vi "pickOffensiveRobots.vi"(8 "error in (no error)":errorcluster, 11 "Game in":refnum<class "Game.lvclass">) -> (0 "error out":errorcluster, 3 "Game out":refnum<class "Game.lvclass">)   [LabVIEW 2021, in "Game.lvclass"]
uses:
  Game.lvclass
  Game.lvclass/Game.ctl
  Team_class/Team.lvclass/Team.ctl
  Playbook_class/Playbook.lvclass/Playbook.ctl
  TestPlay_class/TestPlay.lvclass/TestPlay.ctl
  Robot_class/roles.ctl
  Robot_class/Robot.lvclass/Robot.ctl
  Role_class/Role.lvclass/Role.ctl
  PreparePenaltyAllyPlay_class/PreparePenaltyAllyPlay.lvclass/PreparePenaltyAllyPlay.ctl
  IndirectEnemyPlay_class/IndirectEnemyPlay.lvclass/IndirectEnemyPlay.ctl
  DirectEnemyPlay_class/DirectEnemyPlay.lvclass/DirectEnemyPlay.ctl
  NormalGamePlay_class/NormalGamePlay.lvclass/NormalGamePlay.ctl
  PreparePassInGame1_class/PreparePassInGame1.lvclass/PreparePassInGame1.ctl
  HaltPlay_class/HaltPlay.lvclass/HaltPlay.ctl
  BallOutOfFieldPlay_class/BallOutOfFieldPlay.lvclass/BallOutOfFieldPlay.ctl
  StopOffensivePlay_class/StopOffensivePlay.lvclass/StopOffensivePlay.ctl
  EnemyPossessionAtOurFieldPlay_class/EnemyPossessionAtOurFieldPlay.lvclass/EnemyPossessionAtOurFieldPlay.ctl
  PrepareKickoffAllyPlay_class/PrepareKickoffAllyPlay.lvclass/PrepareKickoffAllyPlay.ctl
  PrepareKickoffEnemyPlay_class/PrepareKickoffEnemyPlay.lvclass/PrepareKickoffEnemyPlay.ctl
  PreparePassPlay_class/PreparePassPlay.lvclass/PreparePassPlay.ctl
  PrepareDoublePassPlay_class/PrepareDoublePassPlay.lvclass/PrepareDoublePassPlay.ctl
  ACBPassPlay_class/ACBPassPlay.lvclass/ACBPassPlay.ctl
  PrepareRollToPassPlay_class/PrepareRollToPassPlay.lvclass/PrepareRollToPassPlay.ctl
  TableWithStrikerPlay_class/TableWithStrikerPlay.lvclass/TableWithStrikerPlay.ctl
  TableWith2ndStrikerPlay_class/TableWith2ndStrikerPlay.lvclass/TableWith2ndStrikerPlay.ctl
  KeeperPassToStrikerPlay_class/KeeperPassToStrikerPlay.lvclass/KeeperPassToStrikerPlay.ctl
  PreparePenaltyEnemyPlay_class/PreparePenaltyEnemyPlay.lvclass/PreparePenaltyEnemyPlay.ctl
  KickPenaltyAllyPlay_class/KickPenaltyAllyPlay.lvclass/KickPenaltyAllyPlay.ctl
  Role_class/Write RobotRef.vi
  TestPlay_class/Read Roles.vi
  Robot_class/Write role.vi
  TestPlay_class/Write Roles.vi
  Playbook_class/Write offensive_plays.vi
  Playbook_class/Read offensive_plays.vi
  TestPlay_class/Read NumberOfRobots.vi
  PreparePenaltyAllyPlay_class/Read Roles.vi
  PreparePenaltyAllyPlay_class/Write Roles.vi
  PreparePenaltyAllyPlay_class/Read NumberOfRobots.vi
  IndirectEnemyPlay_class/Read Roles.vi
  IndirectEnemyPlay_class/Write Roles.vi
  DirectEnemyPlay_class/Read Roles.vi
  DirectEnemyPlay_class/Write Roles.vi
  Read EnemyRef.vi
  Read NewParameters.vi
  Team_class/Read RobotRef.vi
  NormalGamePlay_class/Read Roles.vi
  NormalGamePlay_class/Write Roles.vi
  NormalGamePlay_class/Read NumberOfRobots.vi
  PreparePassInGame1_class/Read Roles.vi
  PreparePassInGame1_class/Write Roles.vi
  HaltPlay_class/Read Roles.vi
  HaltPlay_class/Write Roles.vi
  BallOutOfFieldPlay_class/Read Roles.vi
  BallOutOfFieldPlay_class/Write Roles.vi
  BallOutOfFieldPlay_class/Read NumberOfRobots.vi
  StopOffensivePlay_class/Read Roles.vi
  StopOffensivePlay_class/Write Roles.vi
  StopOffensivePlay_class/Read NumberOfRobots.vi
  EnemyPossessionAtOurFieldPlay_class/Read Roles.vi
  EnemyPossessionAtOurFieldPlay_class/Write Roles.vi
  PrepareKickoffAllyPlay_class/Read Roles.vi
  PrepareKickoffAllyPlay_class/Write Roles.vi
  PrepareKickoffEnemyPlay_class/Read Roles.vi
  PrepareKickoffEnemyPlay_class/Write Roles.vi
  PreparePassPlay_class/Read Roles.vi
  PreparePassPlay_class/Write Roles.vi
  PrepareDoublePassPlay_class/Read Roles.vi
  PrepareDoublePassPlay_class/Write Roles.vi
  PrepareDoublePassPlay_class/Read NumberOfRobots.vi
  ACBPassPlay_class/Read Roles.vi
  ACBPassPlay_class/Write Roles.vi
  ACBPassPlay_class/Read NumberOfRobots.vi
  PrepareRollToPassPlay_class/Read Roles.vi
  PrepareRollToPassPlay_class/Write Roles.vi
  PrepareRollToPassPlay_class/Read NumberOfRobots.vi
  TableWithStrikerPlay_class/Read Roles.vi
  TableWithStrikerPlay_class/Write Roles.vi
  TableWithStrikerPlay_class/Read NumberOfRobots.vi
  TableWith2ndStrikerPlay_class/Read Roles.vi
  TableWith2ndStrikerPlay_class/Write Roles.vi
  TableWith2ndStrikerPlay_class/Read NumberOfRobots.vi
  KeeperPassToStrikerPlay_class/Read Roles.vi
  KeeperPassToStrikerPlay_class/Write Roles.vi
  KeeperPassToStrikerPlay_class/Read NumberOfRobots.vi
  PreparePenaltyEnemyPlay_class/Read roles.vi
  PreparePenaltyEnemyPlay_class/Write roles.vi
  PreparePenaltyEnemyPlay_class/Read NumberOfRobots.vi
  KickPenaltyAllyPlay_class/Read Roles.vi
  KickPenaltyAllyPlay_class/Write Rolesvi.vi
  KickPenaltyAllyPlay_class/Read NumberOfRobots.vi
  Read OffensiveTeam.vi
  Read AllyRef.vi
  Read Referee.vi
  Read TestMode IDs.vi
  Read KeeperTeam.vi
  Team_class/Read OffensivePlay.vi
  Team_class/Write OffensivePlay.vi
  Team_class/Write RobotRef.vi
  Write OffensiveTeam.vi
  Ally_class/Ally.lvclass
  C:/Users/rdapa/Desktop/RoboIME/SSL_AI/Team_class/Team.lvclass
  TestRole_class/TestRole.lvclass
  C:/Users/rdapa/Desktop/RoboIME/SSL_AI/Role_class/Role.lvclass
  PassBestReceiverRole_class/PassBestReceiverRole.lvclass
  5RobotsRole_class/5RobotsRole.lvclass
  AttackerAimGoalRole_class/AttackerAimGoalRole.lvclass
  PenaltyDefenseRole_class/PenaltyDefenseRole.lvclass
  AttackerBlockRole_class/AttackerBlockRole.lvclass
  MarkerRole_class/MarkerRole.lvclass
  Enemy_class/Enemy.lvclass
  ShootRole_class/ShootRole.lvclass
  FollowAttackerRole_class/FollowAttackerRole.lvclass
  AttackerStopRole_class/AttackerStopRole.lvclass
  PassBestRobotRole_class/PassBestRobotRole.lvclass
  PreparePassReceiverRole_class/PreparePassReceiverRole.lvclass
  HaltRole_class/HaltRole.lvclass
  BallOutOfFieldRole_class/BallOutOfFieldRole.lvclass
  ABCFirstKickerRole_class/ABCFirstKickerRole.lvclass
  ABCSecondKicker_class/ABCSecondKicker.lvclass
  ABCThirdKicker_class/ABCThirdKicker.lvclass
  PrepareRollToPassReceiverRole_class/PrepareRollToPassReceiverRole.lvclass
  PrepareRollToPassRollerRole_class/PrepareRollToPassRollerRole.lvclass
  SimplePassReceiverRole_class/SimplePassReceiverRole.lvclass
  SimplePassRollRole_class/SimplePassRollRole.lvclass
  PassKickerRole_class/PassKickerRole.lvclass
  PassReceiverRole_class/PassReceiverRole.lvclass
  PassObserverRole_class/PassObserverRole.lvclass
  TableFinalizerRole_class/TableFinalizerRole.lvclass
  TablerRole_class/TablerRole.lvclass
  WaitPassRole_class/WaitPassRole.lvclass
  PenaltyAttackerRole_class/PenaltyAttackerRole.lvclass
  Referee_class/Referee.lvclass
  Playbook_class/Playbook.lvclass
  Robot_class/Robot.lvclass
  Play_class/Play.lvclass
  TestPlay_class/TestPlay.lvclass
  EnemyPossessionAtEnemyFieldPlay_class/EnemyPossessionAtEnemyFieldPlay.lvclass
  EnemyPossessionAtOurFieldPlay_class/EnemyPossessionAtOurFieldPlay.lvclass
  NormalGamePlay_class/NormalGamePlay.lvclass
  IndirectEnemyPlay_class/IndirectEnemyPlay.lvclass
  PrepareKickoffAllyPlay_class/PrepareKickoffAllyPlay.lvclass
  PrepareKickoffEnemyPlay_class/PrepareKickoffEnemyPlay.lvclass
  KickPenaltyAllyPlay_class/KickPenaltyAllyPlay.lvclass
  PreparePenaltyAllyPlay_class/PreparePenaltyAllyPlay.lvclass
  DirectEnemyPlay_class/DirectEnemyPlay.lvclass
  PreparePenaltyEnemyPlay_class/PreparePenaltyEnemyPlay.lvclass
  BallOutOfFieldPlay_class/BallOutOfFieldPlay.lvclass
  StopOffensivePlay_class/StopOffensivePlay.lvclass
  PassPlay_class/PassPlay.lvclass
  DirectKickPlay_class/DirectKickPlay.lvclass
  HaltPlay_class/HaltPlay.lvclass
  PreparePassPlay_class/PreparePassPlay.lvclass
  PassToStriker_class/PassToStriker.lvclass
  PassTo2ndStriker_class/PassTo2ndStriker.lvclass
  SimplePass_class/SimplePass.lvclass
  PrepareRollToPassPlay_class/PrepareRollToPassPlay.lvclass
  PrepareDoublePassPlay_class/PrepareDoublePassPlay.lvclass
  TableWith2ndStrikerPlay_class/TableWith2ndStrikerPlay.lvclass
  TableWithStrikerPlay_class/TableWithStrikerPlay.lvclass
  PrepareTriplePassPlay_class/PrepareTriplePassPlay.lvclass
  ABCPassPlay_class/ABCPassPlay.lvclass
  PreparePassInGame1_class/PreparePassInGame1.lvclass
  ACBPassPlay_class/ACBPassPlay.lvclass
  PrepareKeeperPassPlay_class/PrepareKeeperPassPlay.lvclass
  KeeperPassToStrikerPlay_class/KeeperPassToStrikerPlay.lvclass
  5RobotsNormalGamePlay_class/5RobotsNormalGamePlay.lvclass
  5RobotsPassGamePlay_class/5RobotsPassGamePlay.lvclass
  5RobotsKeeperGame_class/5RobotsKeeperGame.lvclass
  5PreparePassGamePlay_class/5PreparePassGamePlay.lvclass
  Role_class/Role.lvclass
  SecondMarkerRole_class/SecondMarkerRole.lvclass
  MarkerSkill_class/MarkerSkill.lvclass
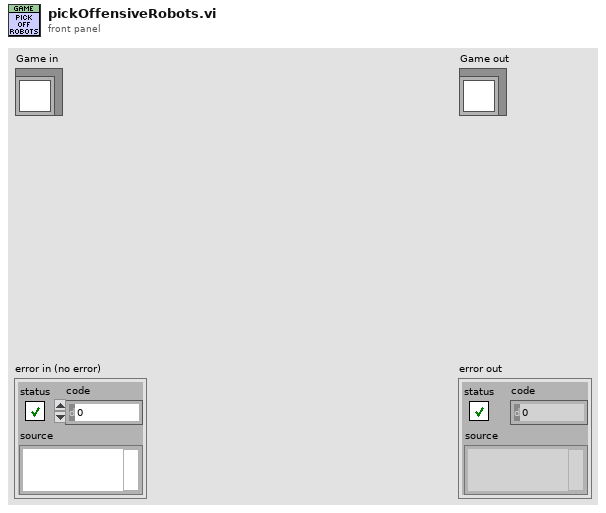
[diagram p1: front panel]
types:
  T1 = typedef "roles.ctl" = enum16{"SimpleBallPlacement", "BallPlacementAllyPasser", "BallPlacementAllyReceiver", "BallPlacementEnemy", "5Robots5th", "PassBestReceiver", "5Robots4th", "5Robots3rd", "5Robots2nd", "5Robots1st", "PassBestRobot", "WaitPass", "ABCThirdKicker", "ABCFirstKicker", "ABCSecondKicker", "Tabler", "TableFinalizer", "PrepareRollToPassRoller", "PrepareRollToPassReceiver", "SimplePassRoll", "SimplePassRollReceiver", "PenaltyDefense", "PreparePassReceiver 2", "PreparePassReceiver 1", "PassObserver", "Timeout", "Goto", "ZigZag", "None", "BallOutOfField", "DefenderArea", "Duelist", "AttackerStop", "FollowAttacker", "KeeperRole", "KickPenalty", "AttackerAimGoal", "AttackerBlock", "Marker", "Halt", "Shoot", "PassKicker", "PassReceiver", "TestRole", "PenaltyAttacker"}
  T2 = typedef "NewParameters.ctl" = cluster{"PenaltyDistance":dbl, "DistanceAttackerToBackBall":dbl, "Division":enum16{"Div B", "Div A"}, "DistanceToAvoidyEnemyRobot":dbl, "BallPlacementDistance":dbl, "DisatanceBehindBallToStealBall":dbl, "MaxDistanceToPositionKickoff":dbl, "BlockEnemyTarget":bool, "MaxStopVAng":dbl, "DistanceMarkerToEnemy":dbl, "IgnoreDribblerContact":bool, "DistanceToBeginEnemyPosession":dbl, "GoToBallWhenEnemyNotMoving":bool, "EnemyDistanceToReduceVelocity":dbl, "TurnOnEnemyDistanceToReduceVelocity":bool, "EnemyDistanceToShootOutBall":dbl, "DefenseKickBall":bool, "MoreKickToGoal? (0-0.3)":dbl, "ChipKickInEnemyField":bool, "ShootOutRobotId":dbl, "FieldLenghtDenominatorInShootOut":dbl, "AdjustPositionInBallPlacement":bool, "PowerGodPass":dbl, "VelocityAbortEnemyPos":dbl, "MaxDistToBeginPass":dbl, "MinDistToBeginPass":dbl, "VelocityInDirects":dbl, "BadDribblerIDs":i32[], "NewKickToDistanceAroundBall":dbl, "PowerAvoidColisionMarker":dbl, "DistanceToAvoidColisionMarker":dbl, "AvoidBallKick":dbl, "DistanceTryKick":dbl, "SuicideKickDIstance":dbl, "FirstKickAtck":bool, "AdjustFirstKickDistance":dbl, "FirstKickDefense":bool, "AvoidAimLessKick":dbl, "DistanceToAvoidyEnemyShootRobot ":dbl, "NumberOfMarkers":dbl, "PotField":bool, "PIDLateral":bool, "MinDistanceFirstKickX":dbl, "MinDistanceFirstKickY":dbl, "FractionOfDistToTouchGround\nAfterChipKick":dbl, "FractionOfKickxWhen\nComposedWithKickz":dbl, "Style":T3, "MoveInTurnState":bool, "DistFromEnemyToConsider\nMoveInTurnState":dbl, "CascadePID":bool, "TurnAroundParameters":cluster{"Radius":dbl, "Multiplier":dbl, "ChordAngle":dbl}, "SafeDriveVel":dbl, "DistanceToGoToBackBall":dbl, "minDistanceToNotFinishEnemyPossession":dbl, "TheBestKickers":i32[]}
  T3 = typedef "Style.ctl" = enum16{"Insanity", "Offensive", "Defensive"}
  T4 = typedef "OffensivePlay.ctl" = enum16{"5RobotsPassGamePlay", "5PreparePassGame", "5RobotsKeeperGame", "KeeperPassToStriker", "5RobotsNormalGamePlay", "PrepareKeeperPass", "ACBPass", "ABCPass", "PrepareTriplePass", "TableWithStriker", "TableWith2ndStrikerPlay", "PrepareDoublePass", "PrepareRollToPass", "SimplePass", "PreparePass", "PassToStriker", "BallOutOfField", "PassTo2ndStriker", "StopOffensive", "Prepare Penalty Enemy", "EnemyPossessionAtEnemyField", "EnemyPossesionAtOurField", "TestPlay", "PreparePenaltyAlly", "KickPenaltyAlly", "PrepareKickoffAlly", "PrepareKickoffEnemy", "IndirectEnemy", "DirectEnemy", "PreparePassInGame1", "NormalGame", "DirectKick", "Pass", "Halt", "Timeout", "PassPlay", "PenaltyEnemy"}
  T5 = typedef "offensive_plays.ctl" = cluster{"Play":refnum<class "Play.lvclass">, "TestPlay":refnum<class "TestPlay.lvclass">, "EnemyPossessionAtEnemyFieldPlay":refnum<class "EnemyPossessionAtEnemyFieldPlay.lvclass">, "EnemyPossessionAtOurFieldPlay":refnum<class "EnemyPossessionAtOurFieldPlay.lvclass">, "NormalGamePlay":refnum<class "NormalGamePlay.lvclass">, "IndirectEnemyPlay":refnum<class "IndirectEnemyPlay.lvclass">, "PrepareKickoffAllyPlay":refnum<class "PrepareKickoffAllyPlay.lvclass">, "PrepareKickoffEnemyPlay":refnum<class "PrepareKickoffEnemyPlay.lvclass">, "KickPenaltyAllyPlay":refnum<class "KickPenaltyAllyPlay.lvclass">, "PreparePenaltyAllyPlay":refnum<class "PreparePenaltyAllyPlay.lvclass">, "DirectEnemyPlay":refnum<class "DirectEnemyPlay.lvclass">, "PreparePenaltyEnemyPlay":refnum<class "PreparePenaltyEnemyPlay.lvclass">, "BallOutOfFieldPlay":refnum<class "BallOutOfFieldPlay.lvclass">, "StopOffensivePlay":refnum<class "StopOffensivePlay.lvclass">, "PassPlay":refnum<class "PassPlay.lvclass">, "DirectKickPlay":refnum<class "DirectKickPlay.lvclass">, "HaltPlay":refnum<class "HaltPlay.lvclass">, "PreparePassPlay":refnum<class "PreparePassPlay.lvclass">, "PassToStrikerPlay":refnum<class "PassToStriker.lvclass">, "PassTo2ndStrikerPlay":refnum<class "PassTo2ndStriker.lvclass">, "SimplePassPlay":refnum<class "SimplePass.lvclass">, "PrepareRollToPassPlay":refnum<class "PrepareRollToPassPlay.lvclass">, "PrepareDoublePassPlay":refnum<class "PrepareDoublePassPlay.lvclass">, "TableWith2ndStrikerPlay":refnum<class "TableWith2ndStrikerPlay.lvclass">, "TableWithStrikerPlay":refnum<class "TableWithStrikerPlay.lvclass">, "PrepareTriplePassPlay":refnum<class "PrepareTriplePassPlay.lvclass">, "ABCPassPlay":refnum<class "ABCPassPlay.lvclass">, "PreparePassInGame1":refnum<class "PreparePassInGame1.lvclass">, "ACBPassPlay":refnum<class "ACBPassPlay.lvclass">, "PrepareKeeperPassPlay":refnum<class "PrepareKeeperPassPlay.lvclass">, "KeeperPassToStrikerPlay":refnum<class "KeeperPassToStrikerPlay.lvclass">, "SimplePass":refnum<class "SimplePass.lvclass">, "SimplePass 2":refnum<class "SimplePass.lvclass">, "5RobotsNormalGamePlay":refnum<class "5RobotsNormalGamePlay.lvclass">, "5RobotsPassGamePlay":refnum<class "5RobotsPassGamePlay.lvclass">, "5RobotsKeeperGame":refnum<class "5RobotsKeeperGame.lvclass">, "5PreparePassGamePlay":refnum<class "5PreparePassGamePlay.lvclass">}
  T6 = cluster{"TestRole 1":refnum<class "TestRole.lvclass">, "Role":refnum<class "Role.lvclass">, "TestRole 2":refnum<class "TestRole.lvclass">, "TestRole 3":refnum<class "TestRole.lvclass">}
  T7 = cluster{"5RobotsRole3rd":refnum<class "5RobotsRole.lvclass">, "5RobotsRole2nd":refnum<class "5RobotsRole.lvclass">, "5RobotsRole1st":refnum<class "5RobotsRole.lvclass">, "5RobotsRole4th":refnum<class "5RobotsRole.lvclass">, "PassBestReceiverRole":refnum<class "PassBestReceiverRole.lvclass">}
  T8 = cluster{"AttackerAimGoalRole":refnum<class "AttackerAimGoalRole.lvclass">, "PenaltyDefenseRole 4":refnum<class "PenaltyDefenseRole.lvclass">, "PenaltyDefenseRole 1":refnum<class "PenaltyDefenseRole.lvclass">, "PenaltyDefenseRole 2":refnum<class "PenaltyDefenseRole.lvclass">, "PenaltyDefenseRole 3":refnum<class "PenaltyDefenseRole.lvclass">}
  T9 = cluster{"AttackerBlockRole":refnum<class "AttackerBlockRole.lvclass">, "MarkerRole":refnum<class "MarkerRole.lvclass">}
  T10 = typedef "directEnemyRoles.ctl" = cluster{"AttackerBlockRole":refnum<class "AttackerBlockRole.lvclass">, "MarkerRole":refnum<class "MarkerRole.lvclass">, "SecondMarkerRole":refnum<class "SecondMarkerRole.lvclass">}
  T11 = cluster{"ShootRole":refnum<class "ShootRole.lvclass">, "FollowAttackerRole":refnum<class "FollowAttackerRole.lvclass">}
  T12 = cluster{"5RobotsRole1st":refnum<class "5RobotsRole.lvclass">, "5RobotsRole2nd ":refnum<class "5RobotsRole.lvclass">, "5RobotsRole3rd":refnum<class "5RobotsRole.lvclass">, "5RobotsRole4th":refnum<class "5RobotsRole.lvclass">, "ShootRole":refnum<class "ShootRole.lvclass">}
  T13 = cluster{"5RobotsRole1st":refnum<class "5RobotsRole.lvclass">, "5RobotsRole2nd ":refnum<class "5RobotsRole.lvclass">, "5RobotsRole3rd":refnum<class "5RobotsRole.lvclass">, "5RobotsRole4th":refnum<class "5RobotsRole.lvclass">, "AttackerStopRole":refnum<class "AttackerStopRole.lvclass">}
  T14 = cluster{"PassBestRobotRole":refnum<class "PassBestRobotRole.lvclass">, "5RobotsRole3rd":refnum<class "5RobotsRole.lvclass">, "5RobotsRole2nd":refnum<class "5RobotsRole.lvclass">, "5RobotsRole1st":refnum<class "5RobotsRole.lvclass">, "PassBestReceiverRole":refnum<class "PassBestReceiverRole.lvclass">}
  T15 = cluster{"PreparePassReceiverRole1":refnum<class "PreparePassReceiverRole.lvclass">, "PreparePassReceiverRole 2":refnum<class "PreparePassReceiverRole.lvclass">}
  T16 = cluster{"ShootRole":refnum<class "ShootRole.lvclass">, "PreparePassReceiverRole1":refnum<class "PreparePassReceiverRole.lvclass">, "PreparePassReceiverRole2":refnum<class "PreparePassReceiverRole.lvclass">}
  T17 = cluster{"HaltRole 1":refnum<class "HaltRole.lvclass">, "HaltRole 2":refnum<class "HaltRole.lvclass">, "HaltRole 3":refnum<class "HaltRole.lvclass">, "HaltRole 4":refnum<class "HaltRole.lvclass">, "HaltRole 5":refnum<class "HaltRole.lvclass">, "HaltRole 6":refnum<class "HaltRole.lvclass">}
  T18 = cluster{"BallOutOfFieldRole":refnum<class "BallOutOfFieldRole.lvclass">, "FollowAttackerRole":refnum<class "FollowAttackerRole.lvclass">}
  T19 = cluster{"MarkerRole":refnum<class "MarkerRole.lvclass">, "AttackerStopRole":refnum<class "AttackerStopRole.lvclass">}
  T20 = typedef "EnemyPossessionAtOurFieldRoles.ctl" = cluster{"ShootRole":refnum<class "ShootRole.lvclass">, "MarkerRole":refnum<class "MarkerRole.lvclass">}
  T21 = cluster{"AttackerAimGoalRole":refnum<class "AttackerAimGoalRole.lvclass">, "FollowAttackerRole":refnum<class "FollowAttackerRole.lvclass">}
  T22 = cluster{"AttackerBlockRole":refnum<class "AttackerBlockRole.lvclass">, "FollowAttackerRole":refnum<class "FollowAttackerRole.lvclass">}
  T23 = cluster{"PreparePassReceiverRole 1":refnum<class "PreparePassReceiverRole.lvclass">, "AttackerStopRole":refnum<class "AttackerStopRole.lvclass">, "PreparePassReceiverRole 2":refnum<class "PreparePassReceiverRole.lvclass">}
  T24 = cluster{"AttackerStopRole":refnum<class "AttackerStopRole.lvclass">, "PreparePassReceiverRole 1":refnum<class "PreparePassReceiverRole.lvclass">, "PreparePassReceiverRole 2":refnum<class "PreparePassReceiverRole.lvclass">}
  T25 = cluster{"PreparePassReceiverRole 1":refnum<class "PreparePassReceiverRole.lvclass">, "PreparePassReceiverRole 2":refnum<class "PreparePassReceiverRole.lvclass">, "AttackerStopRole":refnum<class "AttackerStopRole.lvclass">}
  T26 = cluster{"ABCSecondKicker":refnum<class "ABCSecondKicker.lvclass">, "ABCThirdKicker":refnum<class "ABCThirdKicker.lvclass">, "ABCFirstKickerRole":refnum<class "ABCFirstKickerRole.lvclass">}
  T27 = cluster{"PreparePassReceiverRole 1":refnum<class "PreparePassReceiverRole.lvclass">, "PreparePassReceiverRole 2":refnum<class "PreparePassReceiverRole.lvclass">, "PrepareRollToPassReceiverRole":refnum<class "PrepareRollToPassReceiverRole.lvclass">, "PrepareRollToPassRollerRole":refnum<class "PrepareRollToPassRollerRole.lvclass">}
  T28 = cluster{"SimplePassRollRole":refnum<class "SimplePassRollRole.lvclass">, "SimplePassReceiverRole":refnum<class "SimplePassReceiverRole.lvclass">}
  T29 = cluster{"PassKickerRole":refnum<class "PassKickerRole.lvclass">, "PassReceiverRole":refnum<class "PassReceiverRole.lvclass">, "PassObserverRole":refnum<class "PassObserverRole.lvclass">}
  T30 = cluster{"TableFinalizerRole":refnum<class "TableFinalizerRole.lvclass">, "TablerRole":refnum<class "TablerRole.lvclass">, "PassObserverRole":refnum<class "PassObserverRole.lvclass">}
  T31 = cluster{"WaitPassRole":refnum<class "WaitPassRole.lvclass">, "FollowAttackerRole":refnum<class "FollowAttackerRole.lvclass">}
  T32 = cluster{"PenaltyDefenseRole 1":refnum<class "PenaltyDefenseRole.lvclass">, "PenaltyDefenseRole 2":refnum<class "PenaltyDefenseRole.lvclass">, "PenaltyDefenseRole 3":refnum<class "PenaltyDefenseRole.lvclass">, "PenaltyDefenseRole 4":refnum<class "PenaltyDefenseRole.lvclass">, "PenaltyDefenseRole 5":refnum<class "PenaltyDefenseRole.lvclass">}
  T33 = typedef "kickPenaltyAllyRoles.ctl" = cluster{"PenaltyAttackerRole":refnum<class "PenaltyAttackerRole.lvclass">, "HaltRole":refnum<class "HaltRole.lvclass">, "HaltRole 2":refnum<class "HaltRole.lvclass">, "HaltRole 3":refnum<class "HaltRole.lvclass">, "HaltRole 4":refnum<class "HaltRole.lvclass">, "HaltRole 5":refnum<class "HaltRole.lvclass">}
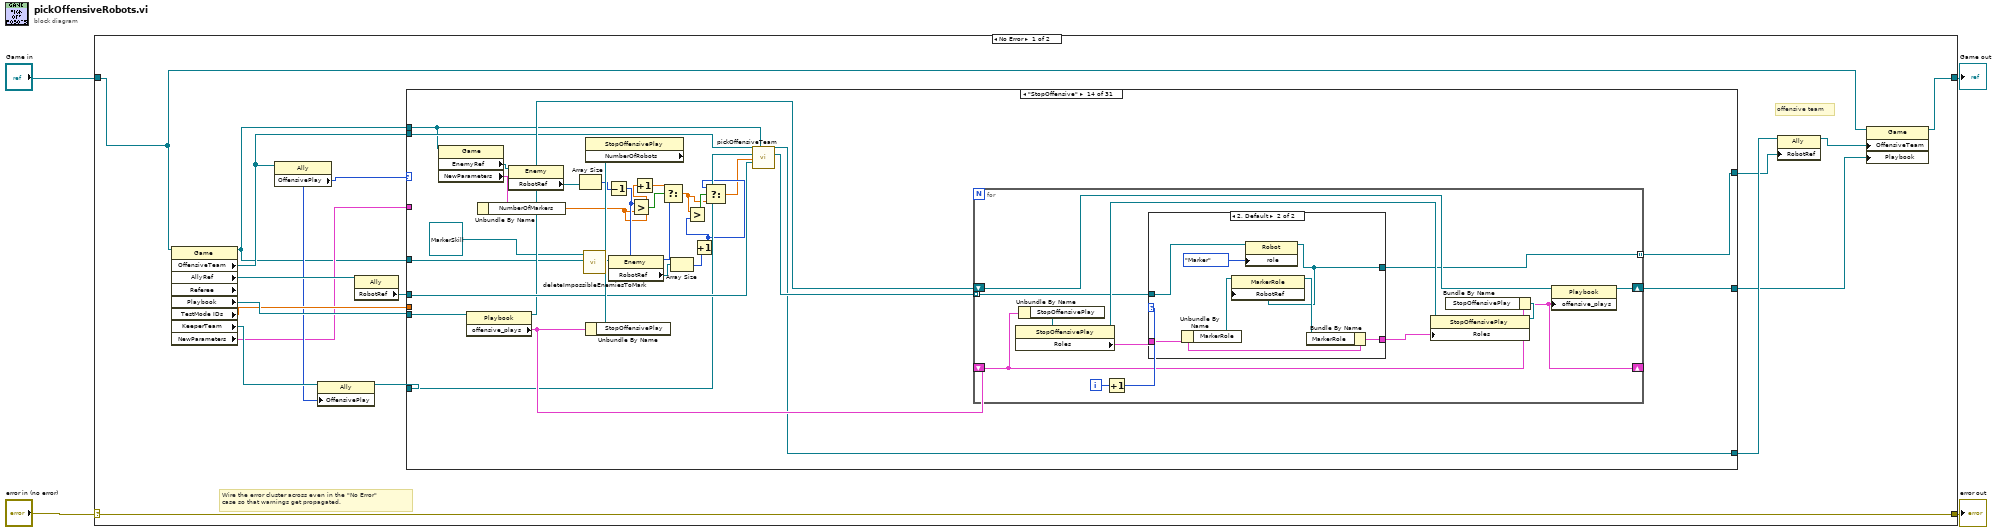
[diagram p0: block diagram]
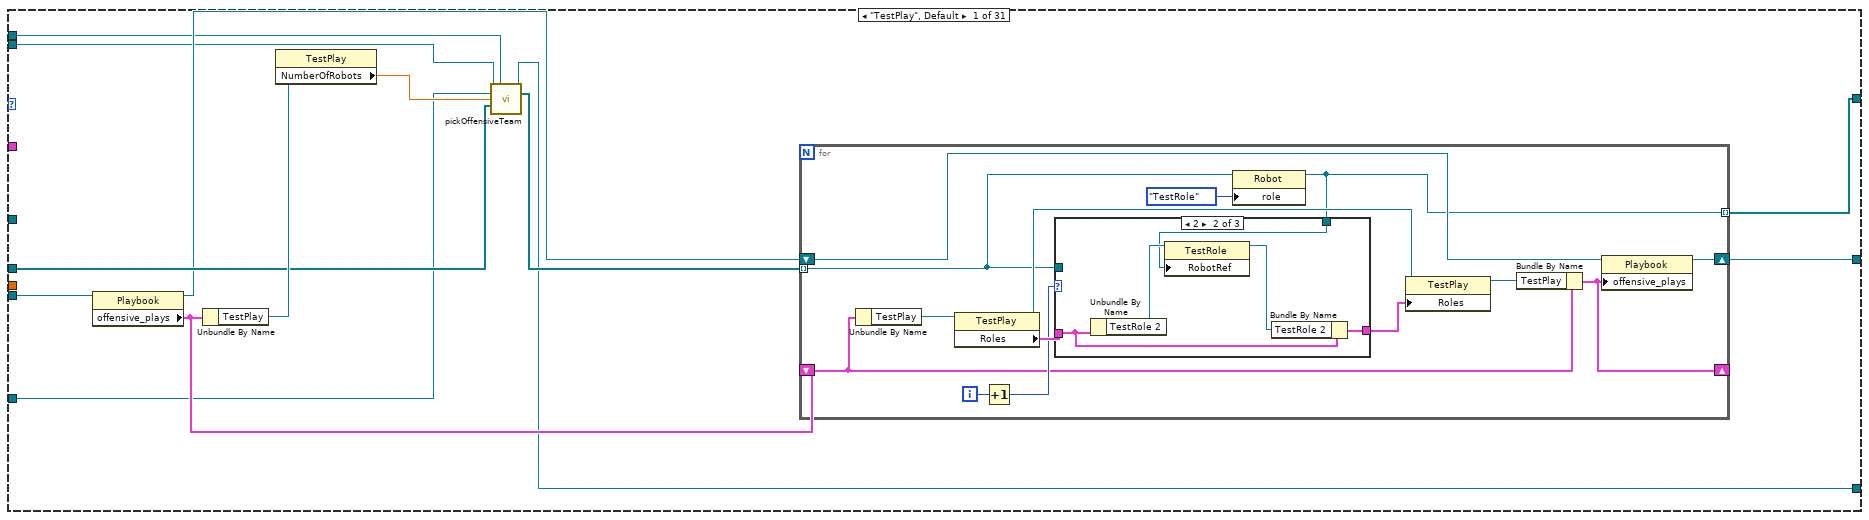
[diagram p2: hidden frame]
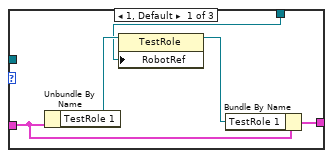
[diagram p3: hidden frame]
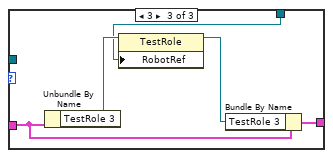
[diagram p4: hidden frame]
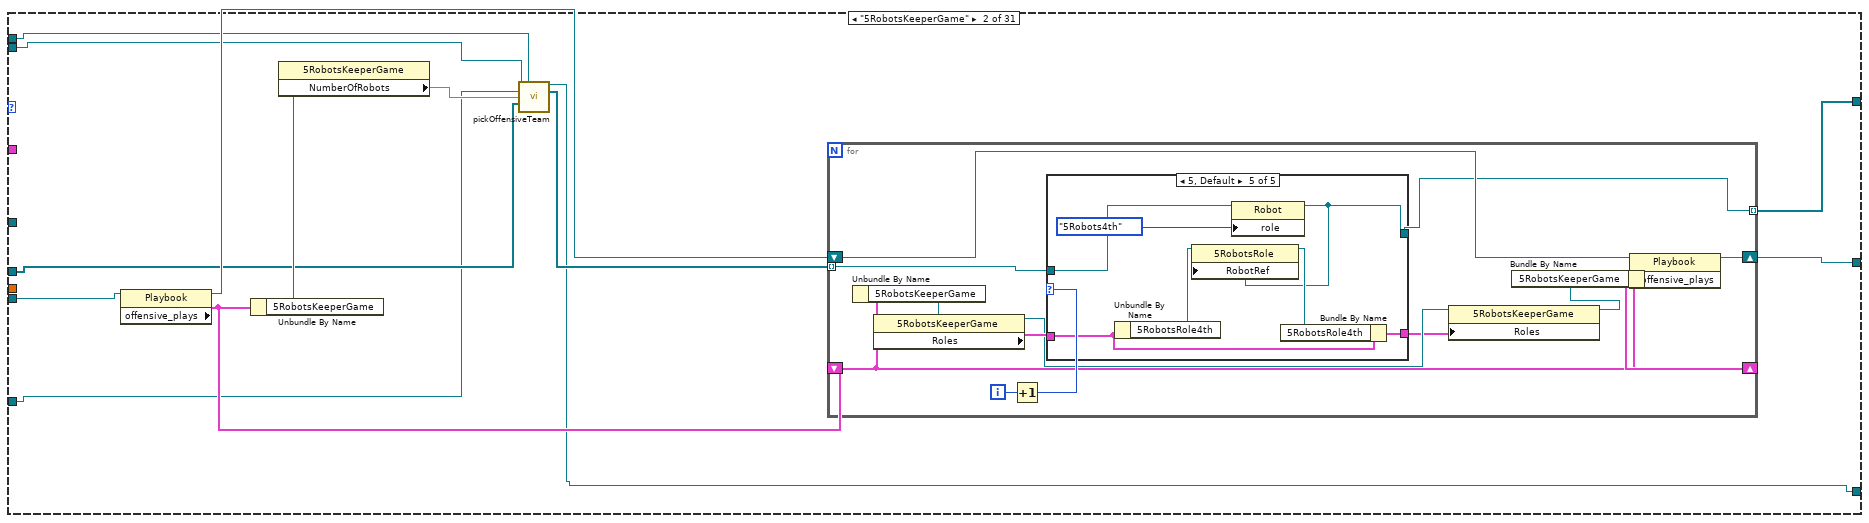
[diagram p5: hidden frame]
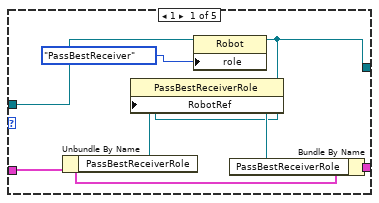
[diagram p6: hidden frame]
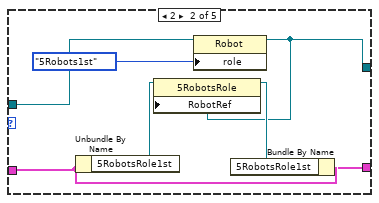
[diagram p7: hidden frame]
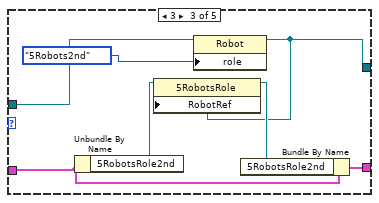
[diagram p8: hidden frame]
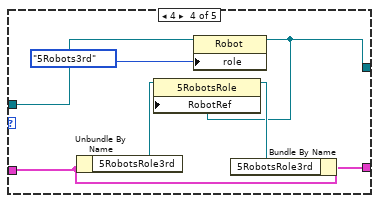
[diagram p9: hidden frame]
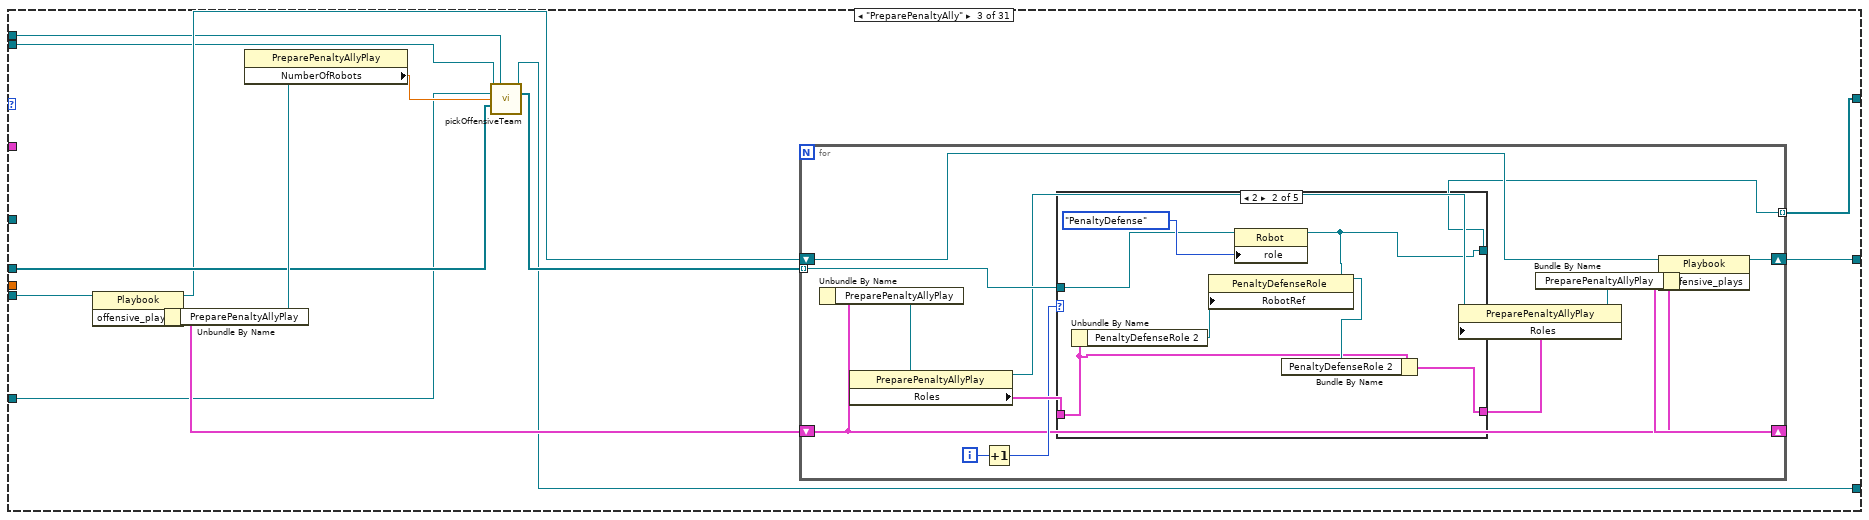
[diagram p10: hidden frame]
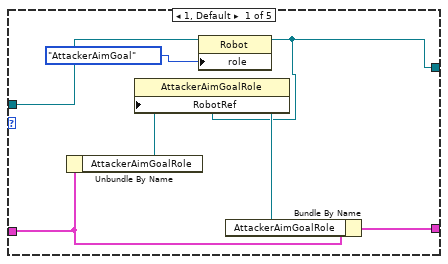
[diagram p11: hidden frame]
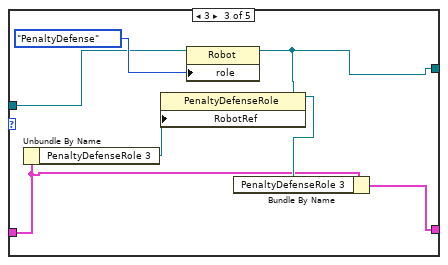
[diagram p12: hidden frame]
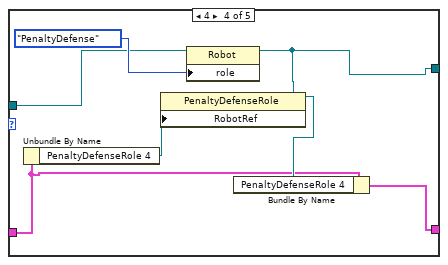
[diagram p13: hidden frame]
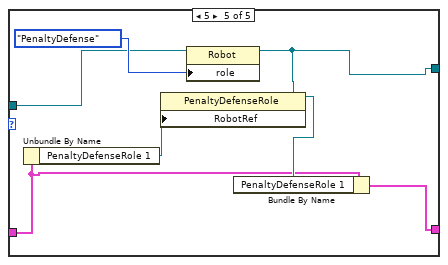
[diagram p14: hidden frame]
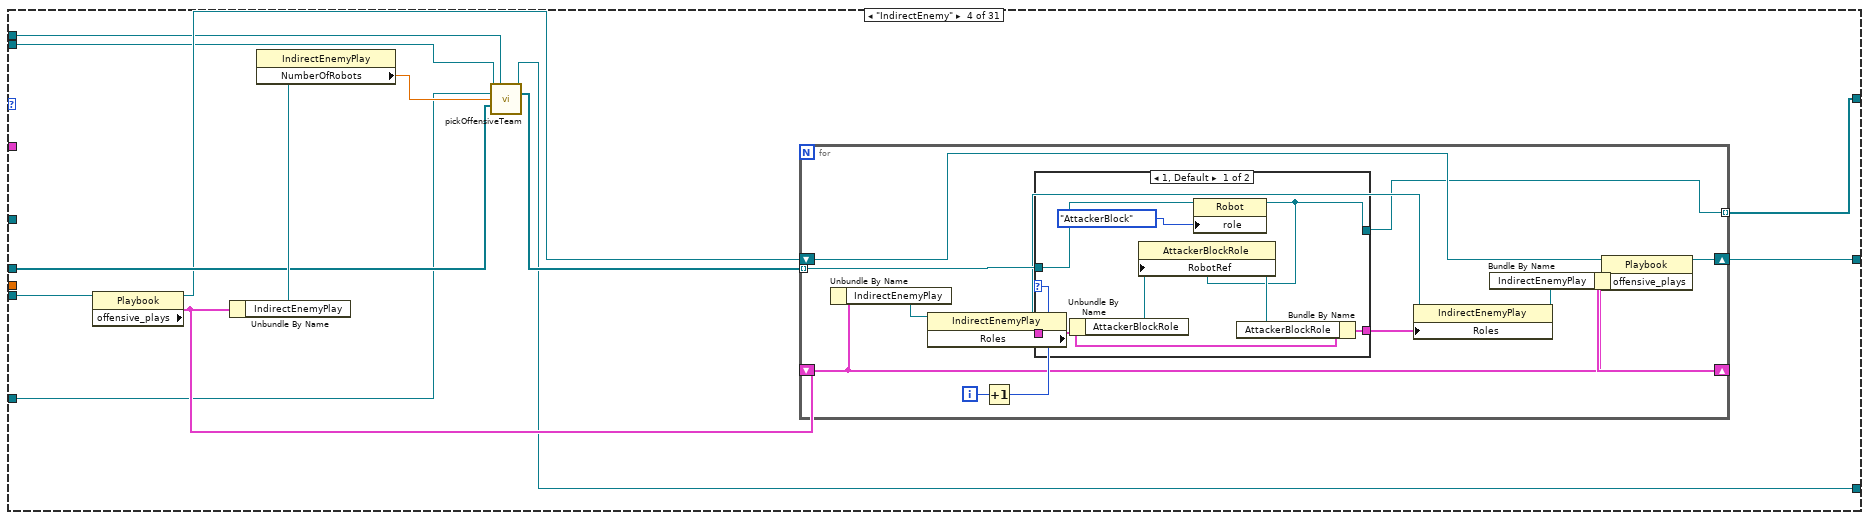
[diagram p15: hidden frame]
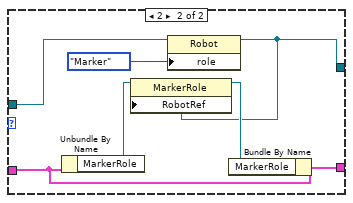
[diagram p16: hidden frame]
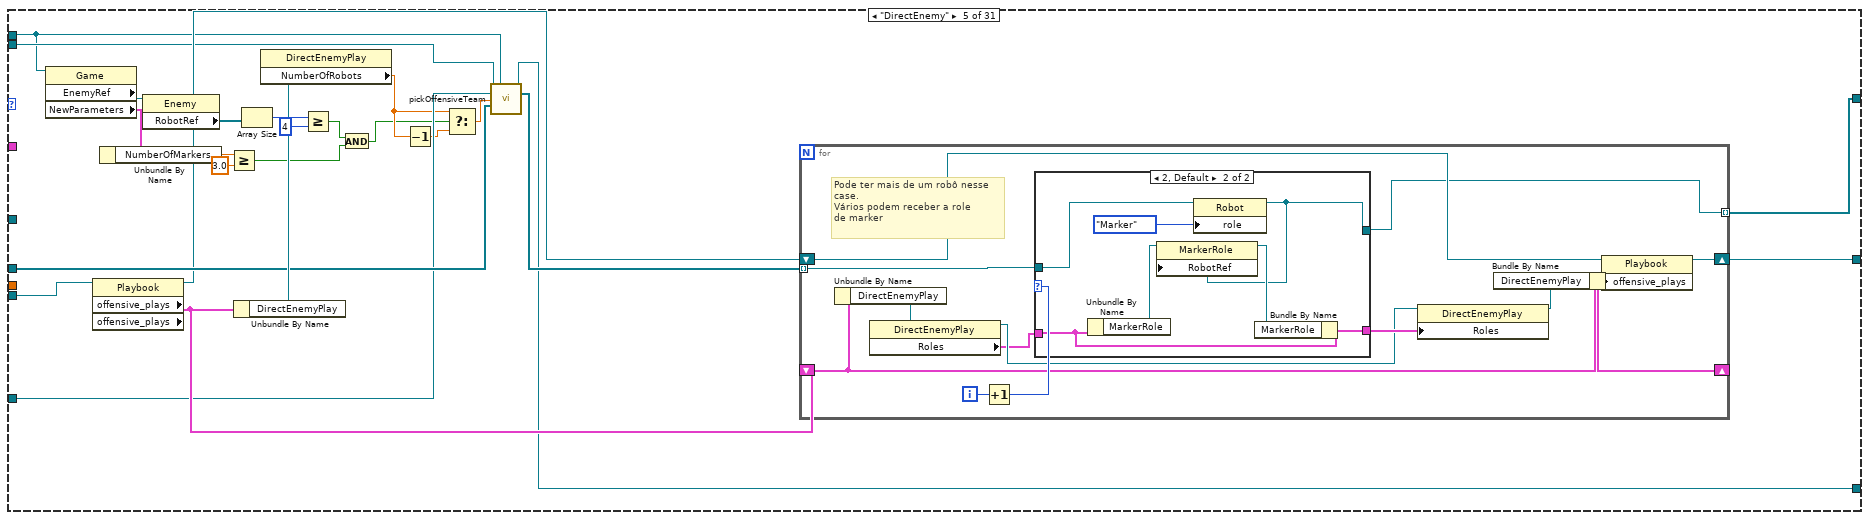
[diagram p17: hidden frame]
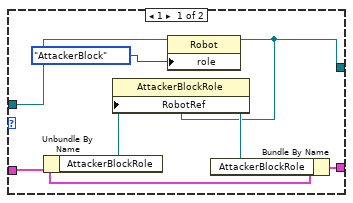
[diagram p18: hidden frame]
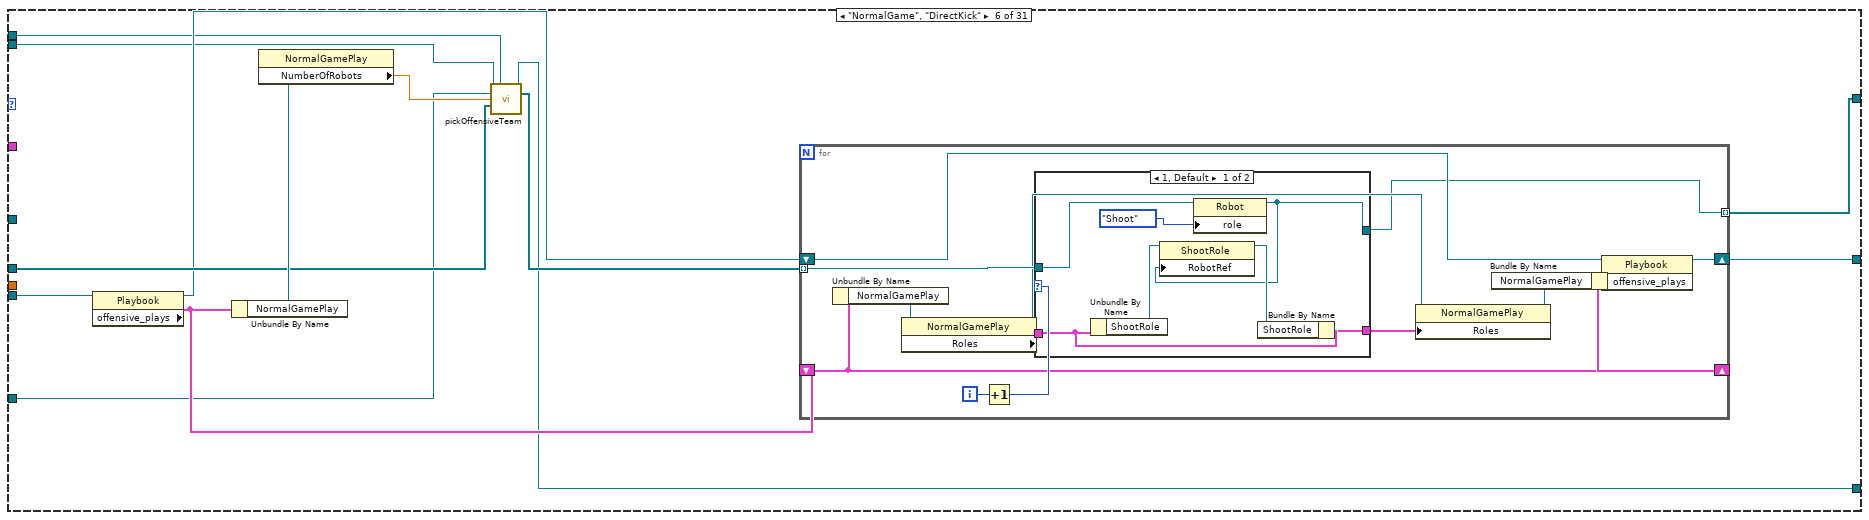
[diagram p19: hidden frame]
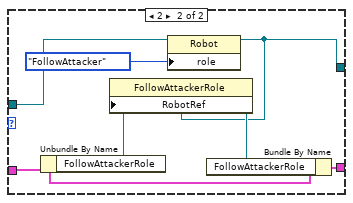
[diagram p20: hidden frame]
diagram:
  n1 = case shown="No Error" "error in (no error)" {
    selector: "error in (no error)" -> [w21 w1560]
    tunnel: [w21 w1560] -> w3
    tunnel: [w14 w1559] -> w1
    tunnel: "Game in" -> [w15 w1559]
    frame No Error {
      # "offensive team"
      # "Wire the error cluster across even in the \"No Error\"\ncase so that warnings get propagated."
      n2 = property class="Game" props=["OffensiveTeam", "AllyRef", "Referee", "Playbook", "TestMode IDs", "KeeperTeam", "NewParameters"](reference=w15) -> (reference out=w5:refnum<class "Game.lvclass">, "OffensiveTeam"=w8:refnum<class "Ally.lvclass">, "AllyRef"=w10:refnum<class "Ally.lvclass">, "Playbook"=w16:refnum<class "Playbook.lvclass">, "TestMode IDs"=w11:dbl[], "KeeperTeam"=w12:refnum<class "Ally.lvclass">, "NewParameters"=w6:T2)  [unwired: 1 in, 2 out]
      n3 = property class="Ally"(reference=w8) -> ("OffensivePlay"=w7:T4)  [unwired: 1 in, 2 out]
      n4 = property class="Ally"(reference=w12, "OffensivePlay"=w7) -> (reference out=w13:refnum<class "Ally.lvclass">)  [unwired: 1 in, 1 out]
      n5 = property class="Ally"(reference=w10) -> ("RobotRef"=w9:refnum<class "Robot.lvclass">[])  [unwired: 1 in, 2 out]
      n6 = case shown="\"StopOffensive\"" w7 {
        tunnel: w16 -> [w34 w68 w137 w198 w250 w290 w321 w384 w447 w519 w559 w608 w676 w732 w772 w812 w852 w887 w934 w981 w1028 w1075 w1123 w1176 w1212 w1263 w1310 w1357 w1404 w1437 w1510]
        tunnel: w9 -> [w28 w69 w131 w192 w245 w284 w326 w389 w452 w513 w553 w598 w670 w727 w767 w806 w846 w886 w933 w980 w1027 w1074 w1122 w1175 w1213 w1264 w1311 w1358 w1405 w1442 w1504]
        tunnel: [w32 w65 w135 w196 w248 w288 w323 w386 w449 w517 w557 w606 w674 w730 w770 w810 w850 w881 w928 w975 w1022 w1069 w1117 w1170 w1215 w1257 w1304 w1351 w1398 w1440 w1508] -> w17
        tunnel: [w31 w64 w134 w195 w247 w287 w322 w385 w448 w516 w556 w605 w673 w729 w769 w809 w849 w880 w927 w974 w1021 w1068 w1116 w1169 w1214 w1256 w1303 w1350 w1397 w1439 w1507] -> w19
        tunnel: [w25 w66 w128 w189 w242 w281 w324 w387 w450 w510 w550 w602 w667 w724 w764 w803 w843 w882 w929 w976 w1023 w1070 w1118 w1171 w1216 w1258 w1305 w1352 w1399 w1441 w1501] -> w20
        tunnel: w13 -> [w24 w67 w127 w188 w241 w280 w325 w388 w451 w509 w549 w601 w666 w723 w763 w802 w842 w888 w935 w982 w1029 w1076 w1124 w1177 w1211 w1262 w1309 w1356 w1403 w1443 w1500]
        tunnel: w8 -> [w23 w70 w126 w187 w240 w279 w327 w390 w453 w508 w548 w600 w665 w722 w762 w801 w841 w885 w932 w979 w1026 w1073 w1121 w1174 w1210 w1259 w1306 w1353 w1400 w1444 w1499]
        tunnel: w5 -> [w22 w71 w125 w186 w239 w278 w328 w391 w454 w507 w547 w599 w664 w718 w761 w800 w840 w884 w931 w978 w1025 w1072 w1120 w1173 w1209 w1260 w1307 w1354 w1401 w1445 w1498]
        tunnel: w11 -> [_ _ _ _ _ _ _ _ _ _ _ w597 _ _ _ _ _ _ _ _ _ _ _ _ _ _ _ _ _ _ _]
        tunnel: w6 -> [_ _ _ _ _ _ w320 w383 w446 _ _ _ _ _ _ _ _ _ _ _ _ _ _ _ _ _ _ _ _ _ _]
        tunnel: w5 -> [_ _ _ _ _ _ _ _ _ _ _ _ _ w712 _ _ _ _ _ _ _ _ _ _ _ _ _ _ _ _ _]
        frame "TestPlay", Default {
          n7 = property class="Playbook"(reference=w34) -> (reference out=w27:refnum<class "Playbook.lvclass">, "offensive_plays"=w33:T5)  [unwired: 1 in, 1 out]
          n8 = Unbundle By Name(w33) -> ("TestPlay"=w30:refnum<class "TestPlay.lvclass">)
          n9 = property class="TestPlay"(reference=w30) -> ("NumberOfRobots"=w29:dbl)  [unwired: 1 in, 2 out]
          n10 = call-dynamic "pickOffensiveTeam.vi"("OffensiveTeam in"=w23, "Game"=w22, "KeeperTeam"=w24, "number_of_robots"=w29, "RobotRef"=w28) -> ("OffensiveTeam out"=w25:refnum<class "Ally.lvclass">, "RobotRef"=w26:refnum<class "Robot.lvclass">[])  [unwired: 8 in, 1 out]
          n11 = for {
            tunnel: [w35] -> w31 mode=indexing
            tunnel: w26 -> [w41] mode=indexing
            shift-right: [w43] -> w32
            shift-left: w27 -> [w44]
            shift-right: [w38] -> _
            shift-left: w33 -> [w37]
            i -> [w40]
            n12 = Unbundle By Name(w37) -> ("TestPlay"=w36:refnum<class "TestPlay.lvclass">)
            n13 = property class="TestPlay"(reference=w36) -> (reference out=w46:refnum<class "TestPlay.lvclass">, "Roles"=w48:T6)  [unwired: 1 in, 1 out]
            n14 = Increment(x=w40) -> (x+1=w39:i32)
            n15 = property class="Robot"(reference=w41, "role"=roles."TestRole") -> (reference out=w35:refnum<class "Robot.lvclass">)  [unwired: 1 in, 1 out]
            n16 = case shown="2" w39 {
              tunnel: w48 -> [w52 w57 w62]
              tunnel: [w50 w55 w60] -> w47
              tunnel: w41 -> [_ _ _]
              tunnel: w35 -> [w49 w54 w59]
              frame 1, Default {
                n17 = Unbundle By Name(w52) -> ("TestRole 1"=w53:refnum<class "TestRole.lvclass">)
                n18 = property class="TestRole"(reference=w53, "RobotRef"=w49) -> (reference out=w51:refnum<class "TestRole.lvclass">)  [unwired: 1 in, 1 out]
                n19 = Bundle By Name(cluster=w52, "TestRole 1"=w51) -> (w50:T6)
              }
              frame 2 {
                n20 = Unbundle By Name(w57) -> ("TestRole 2"=w58:refnum<class "TestRole.lvclass">)
                n21 = property class="TestRole"(reference=w58, "RobotRef"=w54) -> (reference out=w56:refnum<class "TestRole.lvclass">)  [unwired: 1 in, 1 out]
                n22 = Bundle By Name(cluster=w57, "TestRole 2"=w56) -> (w55:T6)
              }
              frame 3 {
                n23 = Unbundle By Name(w62) -> ("TestRole 3"=w63:refnum<class "TestRole.lvclass">)
                n24 = property class="TestRole"(reference=w63, "RobotRef"=w59) -> (reference out=w61:refnum<class "TestRole.lvclass">)  [unwired: 1 in, 1 out]
                n25 = Bundle By Name(cluster=w62, "TestRole 3"=w61) -> (w60:T6)
              }
            }
            n26 = property class="TestPlay"(reference=w46, "Roles"=w47) -> (reference out=w45:refnum<class "TestPlay.lvclass">)  [unwired: 1 in, 1 out]
            n27 = Bundle By Name(cluster=w37, "TestPlay"=w45) -> (w38:T5)
            n28 = property class="Playbook"(reference=w44, "offensive_plays"=w38) -> (reference out=w43:refnum<class "Playbook.lvclass">)  [unwired: 1 in, 1 out]
          }
        }
        frame "5RobotsKeeperGame" {
          n29 = property class="Playbook"(reference=w68) -> (reference out=w74:refnum<class "Playbook.lvclass">, "offensive_plays"=w72:T5)  [unwired: 1 in, 1 out]
          n30 = Unbundle By Name(w72) -> ("5RobotsKeeperGame"=w73:refnum<class "5RobotsKeeperGame.lvclass">)
          n31 = property class="5RobotsKeeperGame"(reference=w73) -> ("NumberOfRobots"=w76:dbl)  [unwired: 1 in, 2 out]
          n32 = call-dynamic "pickOffensiveTeam.vi"("OffensiveTeam in"=w70, "Game"=w71, "KeeperTeam"=w67, "number_of_robots"=w76, "RobotRef"=w69) -> ("OffensiveTeam out"=w66:refnum<class "Ally.lvclass">, "RobotRef"=w75:refnum<class "Robot.lvclass">[])  [unwired: 8 in, 1 out]
          n33 = for {
            tunnel: [w80] -> w64 mode=indexing
            tunnel: w75 -> [w86] mode=indexing
            shift-right: [w87] -> w65
            shift-left: w74 -> [w88]
            shift-right: [w83] -> _
            shift-left: w72 -> [w82]
            i -> [w85]
            n34 = Unbundle By Name(w82) -> ("5RobotsKeeperGame"=w81:refnum<class "5RobotsKeeperGame.lvclass">)
            n35 = property class="5RobotsKeeperGame"(reference=w81) -> (reference out=w78:refnum<class "5RobotsKeeperGame.lvclass">, "Roles"=w89:T7)  [unwired: 1 in, 1 out]
            n36 = Increment(x=w85) -> (x+1=w84:i32)
            n37 = case shown="5, Default" w84 {
              tunnel: w89 -> [w95 w102 w109 w116 w123]
              tunnel: [w93 w100 w107 w114 w121] -> w77
              tunnel: w86 -> [w92 w99 w106 w113 w120]
              tunnel: [w90 w98 w105 w112 w119] -> w80
              frame 1 {
                n38 = Unbundle By Name(w95) -> ("PassBestReceiverRole"=w96:refnum<class "PassBestReceiverRole.lvclass">)
                n39 = property class="Robot"(reference=w92, "role"=roles."PassBestReceiver") -> (reference out=w90:refnum<class "Robot.lvclass">)  [unwired: 1 in, 1 out]
                n40 = property class="PassBestReceiverRole"(reference=w96, "RobotRef"=w90) -> (reference out=w94:refnum<class "PassBestReceiverRole.lvclass">)  [unwired: 1 in, 1 out]
                n41 = Bundle By Name(cluster=w95, "PassBestReceiverRole"=w94) -> (w93:T7)
              }
              frame 2 {
                n42 = Unbundle By Name(w102) -> ("5RobotsRole1st"=w103:refnum<class "5RobotsRole.lvclass">)
                n43 = property class="Robot"(reference=w99, "role"=roles."5Robots1st") -> (reference out=w98:refnum<class "Robot.lvclass">)  [unwired: 1 in, 1 out]
                n44 = property class="5RobotsRole"(reference=w103, "RobotRef"=w98) -> (reference out=w101:refnum<class "5RobotsRole.lvclass">)  [unwired: 1 in, 1 out]
                n45 = Bundle By Name(cluster=w102, "5RobotsRole1st"=w101) -> (w100:T7)
              }
              frame 3 {
                n46 = Unbundle By Name(w109) -> ("5RobotsRole2nd"=w110:refnum<class "5RobotsRole.lvclass">)
                n47 = property class="Robot"(reference=w106, "role"=roles."5Robots2nd") -> (reference out=w105:refnum<class "Robot.lvclass">)  [unwired: 1 in, 1 out]
                n48 = property class="5RobotsRole"(reference=w110, "RobotRef"=w105) -> (reference out=w108:refnum<class "5RobotsRole.lvclass">)  [unwired: 1 in, 1 out]
                n49 = Bundle By Name(cluster=w109, "5RobotsRole2nd"=w108) -> (w107:T7)
              }
              frame 4 {
                n50 = Unbundle By Name(w116) -> ("5RobotsRole3rd"=w117:refnum<class "5RobotsRole.lvclass">)
                n51 = property class="Robot"(reference=w113, "role"=roles."5Robots3rd") -> (reference out=w112:refnum<class "Robot.lvclass">)  [unwired: 1 in, 1 out]
                n52 = property class="5RobotsRole"(reference=w117, "RobotRef"=w112) -> (reference out=w115:refnum<class "5RobotsRole.lvclass">)  [unwired: 1 in, 1 out]
                n53 = Bundle By Name(cluster=w116, "5RobotsRole3rd"=w115) -> (w114:T7)
              }
              frame 5, Default {
                n54 = Unbundle By Name(w123) -> ("5RobotsRole4th"=w124:refnum<class "5RobotsRole.lvclass">)
                n55 = property class="Robot"(reference=w120, "role"=roles."5Robots4th") -> (reference out=w119:refnum<class "Robot.lvclass">)  [unwired: 1 in, 1 out]
                n56 = property class="5RobotsRole"(reference=w124, "RobotRef"=w119) -> (reference out=w122:refnum<class "5RobotsRole.lvclass">)  [unwired: 1 in, 1 out]
                n57 = Bundle By Name(cluster=w123, "5RobotsRole4th"=w122) -> (w121:T7)
              }
            }
            n58 = property class="5RobotsKeeperGame"(reference=w78, "Roles"=w77) -> (reference out=w79:refnum<class "5RobotsKeeperGame.lvclass">)  [unwired: 1 in, 1 out]
            n59 = Bundle By Name(cluster=w82, "5RobotsKeeperGame"=w79) -> (w83:T5)
            n60 = property class="Playbook"(reference=w88, "offensive_plays"=w83) -> (reference out=w87:refnum<class "Playbook.lvclass">)  [unwired: 1 in, 1 out]
          }
        }
        frame "PreparePenaltyAlly" {
          n61 = property class="Playbook"(reference=w137) -> (reference out=w130:refnum<class "Playbook.lvclass">, "offensive_plays"=w136:T5)  [unwired: 1 in, 1 out]
          n62 = Unbundle By Name(w136) -> ("PreparePenaltyAllyPlay"=w133:refnum<class "PreparePenaltyAllyPlay.lvclass">)
          n63 = property class="PreparePenaltyAllyPlay"(reference=w133) -> ("NumberOfRobots"=w132:dbl)  [unwired: 1 in, 2 out]
          n64 = call-dynamic "pickOffensiveTeam.vi"("OffensiveTeam in"=w126, "Game"=w125, "KeeperTeam"=w127, "number_of_robots"=w132, "RobotRef"=w131) -> ("OffensiveTeam out"=w128:refnum<class "Ally.lvclass">, "RobotRef"=w129:refnum<class "Robot.lvclass">[])  [unwired: 8 in, 1 out]
          n65 = for {
            tunnel: [w138] -> w134 mode=indexing
            tunnel: w129 -> [w145] mode=indexing
            shift-right: [w146] -> w135
            shift-left: w130 -> [w147]
            shift-right: [w142] -> _
            shift-left: w136 -> [w141]
            i -> [w144]
            n66 = Unbundle By Name(w141) -> ("PreparePenaltyAllyPlay"=w140:refnum<class "PreparePenaltyAllyPlay.lvclass">)
            n67 = property class="PreparePenaltyAllyPlay"(reference=w140) -> (reference out=w139:refnum<class "PreparePenaltyAllyPlay.lvclass">, "Roles"=w150:T8)  [unwired: 1 in, 1 out]
            n68 = Increment(x=w144) -> (x+1=w143:i32)
            n69 = case shown="2" w143 {
              tunnel: w150 -> [w156 w158 w165 w172 w179]
              tunnel: [w154 w159 w166 w173 w180] -> w149
              tunnel: w145 -> [w153 w161 w168 w175 w182]
              tunnel: [w151 w160 w167 w174 w181] -> w138
              frame 1, Default {
                n70 = Unbundle By Name(w156) -> ("AttackerAimGoalRole"=w157:refnum<class "AttackerAimGoalRole.lvclass">)
                n71 = property class="Robot"(reference=w153, "role"=roles."AttackerAimGoal") -> (reference out=w151:refnum<class "Robot.lvclass">)  [unwired: 1 in, 1 out]
                n72 = property class="AttackerAimGoalRole"(reference=w157, "RobotRef"=w151) -> (reference out=w155:refnum<class "AttackerAimGoalRole.lvclass">)  [unwired: 1 in, 1 out]
                n73 = Bundle By Name(cluster=w156, "AttackerAimGoalRole"=w155) -> (w154:T8)
              }
              frame 2 {
                n74 = Unbundle By Name(w158) -> ("PenaltyDefenseRole 2"=w163:refnum<class "PenaltyDefenseRole.lvclass">)
                n75 = property class="Robot"(reference=w161, "role"=roles."PenaltyDefense") -> (reference out=w160:refnum<class "Robot.lvclass">)  [unwired: 1 in, 1 out]
                n76 = property class="PenaltyDefenseRole"(reference=w163, "RobotRef"=w160) -> (reference out=w164:refnum<class "PenaltyDefenseRole.lvclass">)  [unwired: 1 in, 1 out]
                n77 = Bundle By Name(cluster=w158, "PenaltyDefenseRole 2"=w164) -> (w159:T8)
              }
              frame 3 {
                n78 = Unbundle By Name(w165) -> ("PenaltyDefenseRole 3"=w170:refnum<class "PenaltyDefenseRole.lvclass">)
                n79 = property class="Robot"(reference=w168, "role"=roles."PenaltyDefense") -> (reference out=w167:refnum<class "Robot.lvclass">)  [unwired: 1 in, 1 out]
                n80 = property class="PenaltyDefenseRole"(reference=w170, "RobotRef"=w167) -> (reference out=w171:refnum<class "PenaltyDefenseRole.lvclass">)  [unwired: 1 in, 1 out]
                n81 = Bundle By Name(cluster=w165, "PenaltyDefenseRole 3"=w171) -> (w166:T8)
              }
              frame 4 {
                n82 = Unbundle By Name(w172) -> ("PenaltyDefenseRole 4"=w177:refnum<class "PenaltyDefenseRole.lvclass">)
                n83 = property class="Robot"(reference=w175, "role"=roles."PenaltyDefense") -> (reference out=w174:refnum<class "Robot.lvclass">)  [unwired: 1 in, 1 out]
                n84 = property class="PenaltyDefenseRole"(reference=w177, "RobotRef"=w174) -> (reference out=w178:refnum<class "PenaltyDefenseRole.lvclass">)  [unwired: 1 in, 1 out]
                n85 = Bundle By Name(cluster=w172, "PenaltyDefenseRole 4"=w178) -> (w173:T8)
              }
              frame 5 {
                n86 = Unbundle By Name(w179) -> ("PenaltyDefenseRole 1"=w184:refnum<class "PenaltyDefenseRole.lvclass">)
                n87 = property class="Robot"(reference=w182, "role"=roles."PenaltyDefense") -> (reference out=w181:refnum<class "Robot.lvclass">)  [unwired: 1 in, 1 out]
                n88 = property class="PenaltyDefenseRole"(reference=w184, "RobotRef"=w181) -> (reference out=w185:refnum<class "PenaltyDefenseRole.lvclass">)  [unwired: 1 in, 1 out]
                n89 = Bundle By Name(cluster=w179, "PenaltyDefenseRole 1"=w185) -> (w180:T8)
              }
            }
            n90 = property class="PreparePenaltyAllyPlay"(reference=w139, "Roles"=w149) -> (reference out=w148:refnum<class "PreparePenaltyAllyPlay.lvclass">)  [unwired: 1 in, 1 out]
            n91 = Bundle By Name(cluster=w141, "PreparePenaltyAllyPlay"=w148) -> (w142:T5)
            n92 = property class="Playbook"(reference=w147, "offensive_plays"=w142) -> (reference out=w146:refnum<class "Playbook.lvclass">)  [unwired: 1 in, 1 out]
          }
        }
        frame "IndirectEnemy" {
          n93 = property class="Playbook"(reference=w198) -> (reference out=w191:refnum<class "Playbook.lvclass">, "offensive_plays"=w197:T5)  [unwired: 1 in, 1 out]
          n94 = Unbundle By Name(w197) -> ("IndirectEnemyPlay"=w194:refnum<class "IndirectEnemyPlay.lvclass">)
          n95 = property class="IndirectEnemyPlay"(reference=w194) -> ("NumberOfRobots"=w193:dbl)  [unwired: 1 in, 2 out]
          n96 = call-dynamic "pickOffensiveTeam.vi"("OffensiveTeam in"=w187, "Game"=w186, "KeeperTeam"=w188, "number_of_robots"=w193, "RobotRef"=w192) -> ("OffensiveTeam out"=w189:refnum<class "Ally.lvclass">, "RobotRef"=w190:refnum<class "Robot.lvclass">[])  [unwired: 8 in, 1 out]
          n97 = for {
            tunnel: [w199] -> w195 mode=indexing
            tunnel: w190 -> [w206] mode=indexing
            shift-right: [w207] -> w196
            shift-left: w191 -> [w208]
            shift-right: [w203] -> _
            shift-left: w197 -> [w202]
            i -> [w205]
            n98 = Unbundle By Name(w202) -> ("IndirectEnemyPlay"=w201:refnum<class "IndirectEnemyPlay.lvclass">)
            n99 = property class="IndirectEnemyPlay"(reference=w201) -> (reference out=w200:refnum<class "IndirectEnemyPlay.lvclass">, "Roles"=w211:T9)  [unwired: 1 in, 1 out]
            n100 = Increment(x=w205) -> (x+1=w204:i32)
            n101 = case shown="1, Default" w204 {
              tunnel: w211 -> [w217 w224]
              tunnel: [w215 w222] -> w210
              tunnel: w206 -> [w214 w221]
              tunnel: [w212 w219] -> w199
              frame 1, Default {
                n102 = Unbundle By Name(w217) -> ("AttackerBlockRole"=w218:refnum<class "AttackerBlockRole.lvclass">)
                n103 = property class="Robot"(reference=w214, "role"=roles."AttackerBlock") -> (reference out=w212:refnum<class "Robot.lvclass">)  [unwired: 1 in, 1 out]
                n104 = property class="AttackerBlockRole"(reference=w218, "RobotRef"=w212) -> (reference out=w216:refnum<class "AttackerBlockRole.lvclass">)  [unwired: 1 in, 1 out]
                n105 = Bundle By Name(cluster=w217, "AttackerBlockRole"=w216) -> (w215:T9)
              }
              frame 2 {
                n106 = Unbundle By Name(w224) -> ("MarkerRole"=w225:refnum<class "MarkerRole.lvclass">)
                n107 = property class="Robot"(reference=w221, "role"=roles."Marker") -> (reference out=w219:refnum<class "Robot.lvclass">)  [unwired: 1 in, 1 out]
                n108 = property class="MarkerRole"(reference=w225, "RobotRef"=w219) -> (reference out=w223:refnum<class "MarkerRole.lvclass">)  [unwired: 1 in, 1 out]
                n109 = Bundle By Name(cluster=w224, "MarkerRole"=w223) -> (w222:T9)
              }
            }
            n110 = property class="IndirectEnemyPlay"(reference=w200, "Roles"=w210) -> (reference out=w209:refnum<class "IndirectEnemyPlay.lvclass">)  [unwired: 1 in, 1 out]
            n111 = Bundle By Name(cluster=w202, "IndirectEnemyPlay"=w209) -> (w203:T5)
            n112 = property class="Playbook"(reference=w208, "offensive_plays"=w203) -> (reference out=w207:refnum<class "Playbook.lvclass">)  [unwired: 1 in, 1 out]
          }
        }
        frame "DirectEnemy" {
          n113 = property class="Game"(reference=w239) -> ("EnemyRef"=w238:refnum<class "Enemy.lvclass">, "NewParameters"=w231:T2)  [unwired: 1 in, 2 out]
          n114 = property class="Playbook" props=["offensive_plays", "offensive_plays"](reference=w250) -> (reference out=w244:refnum<class "Playbook.lvclass">, "offensive_plays"=w249:T5)  [unwired: 1 in, 2 out]
          n115 = Unbundle By Name(w231) -> ("NumberOfMarkers"=w229:dbl)
          n116 = property class="Enemy"(reference=w238) -> ("RobotRef"=w237:refnum<class "Robot.lvclass">[])  [unwired: 1 in, 2 out]
          n117 = Greater Or Equal?(x=w229, y=3.0) -> (x >= y?=w227:bool)
          n118 = Unbundle By Name(w249) -> ("DirectEnemyPlay"=w246:refnum<class "DirectEnemyPlay.lvclass">)
          n119 = Array Size(array=w237) -> (size(s)=w236:i32)
          n120 = property class="DirectEnemyPlay"(reference=w246) -> ("NumberOfRobots"=w234:dbl)  [unwired: 1 in, 2 out]
          n121 = Greater Or Equal?(x=w236, y=4) -> (x >= y?=w230:bool)
          n122 = And(x=w230, y=w227) -> (x .and. y?=w226:bool)
          n123 = Decrement(x=w234) -> (x-1=w233:dbl)
          n124 = Select(t=w234, s=w226, f=w233) -> (s? t:f=w232:dbl)
          n125 = call-dynamic "pickOffensiveTeam.vi"("OffensiveTeam in"=w240, "Game"=w239, "KeeperTeam"=w241, "number_of_robots"=w232, "RobotRef"=w245) -> ("OffensiveTeam out"=w242:refnum<class "Ally.lvclass">, "RobotRef"=w243:refnum<class "Robot.lvclass">[])  [unwired: 8 in, 1 out]
          n126 = for {
            tunnel: [w252] -> w247 mode=indexing
            tunnel: w243 -> [w259] mode=indexing
            shift-right: [w260] -> w248
            shift-left: w244 -> [w261]
            shift-right: [w256] -> _
            shift-left: w249 -> [w255]
            i -> [w258]
            # "Pode ter mais de um robô nesse\ncase. \nVários podem receber a role\nde marker"
            n127 = Unbundle By Name(w255) -> ("DirectEnemyPlay"=w254:refnum<class "DirectEnemyPlay.lvclass">)
            n128 = property class="DirectEnemyPlay"(reference=w254) -> (reference out=w253:refnum<class "DirectEnemyPlay.lvclass">, "Roles"=w251:T10)  [unwired: 1 in, 1 out]
            n129 = Increment(x=w258) -> (x+1=w257:i32)
            n130 = case shown="2, Default" w257 {
              tunnel: w251 -> [w269 w276]
              tunnel: [w267 w274] -> w263
              tunnel: w259 -> [w266 w273]
              tunnel: [w264 w271] -> w252
              frame 1 {
                n131 = Unbundle By Name(w269) -> ("AttackerBlockRole"=w270:refnum<class "AttackerBlockRole.lvclass">)
                n132 = property class="Robot"(reference=w266, "role"=roles."AttackerBlock") -> (reference out=w264:refnum<class "Robot.lvclass">)  [unwired: 1 in, 1 out]
                n133 = property class="AttackerBlockRole"(reference=w270, "RobotRef"=w264) -> (reference out=w268:refnum<class "AttackerBlockRole.lvclass">)  [unwired: 1 in, 1 out]
                n134 = Bundle By Name(cluster=w269, "AttackerBlockRole"=w268) -> (w267:T10)
              }
              frame 2, Default {
                n135 = Unbundle By Name(w276) -> ("MarkerRole"=w277:refnum<class "MarkerRole.lvclass">)
                n136 = property class="Robot"(reference=w273, "role"=roles."Marker") -> (reference out=w271:refnum<class "Robot.lvclass">)  [unwired: 1 in, 1 out]
                n137 = property class="MarkerRole"(reference=w277, "RobotRef"=w271) -> (reference out=w275:refnum<class "MarkerRole.lvclass">)  [unwired: 1 in, 1 out]
                n138 = Bundle By Name(cluster=w276, "MarkerRole"=w275) -> (w274:T10)
              }
            }
            n139 = property class="DirectEnemyPlay"(reference=w253, "Roles"=w263) -> (reference out=w262:refnum<class "DirectEnemyPlay.lvclass">)  [unwired: 1 in, 1 out]
            n140 = Bundle By Name(cluster=w255, "DirectEnemyPlay"=w262) -> (w256:T5)
            n141 = property class="Playbook"(reference=w261, "offensive_plays"=w256) -> (reference out=w260:refnum<class "Playbook.lvclass">)  [unwired: 1 in, 1 out]
          }
        }
        frame "NormalGame", "DirectKick" {
          n142 = property class="Playbook"(reference=w290) -> (reference out=w283:refnum<class "Playbook.lvclass">, "offensive_plays"=w289:T5)  [unwired: 1 in, 1 out]
          n143 = Unbundle By Name(w289) -> ("NormalGamePlay"=w286:refnum<class "NormalGamePlay.lvclass">)
          n144 = property class="NormalGamePlay"(reference=w286) -> ("NumberOfRobots"=w285:dbl)  [unwired: 1 in, 2 out]
          n145 = call-dynamic "pickOffensiveTeam.vi"("OffensiveTeam in"=w279, "Game"=w278, "KeeperTeam"=w280, "number_of_robots"=w285, "RobotRef"=w284) -> ("OffensiveTeam out"=w281:refnum<class "Ally.lvclass">, "RobotRef"=w282:refnum<class "Robot.lvclass">[])  [unwired: 8 in, 1 out]
          n146 = for {
            tunnel: [w291] -> w287 mode=indexing
            tunnel: w282 -> [w298] mode=indexing
            shift-right: [w299] -> w288
            shift-left: w283 -> [w300]
            shift-right: [w295] -> _
            shift-left: w289 -> [w294]
            i -> [w297]
            n147 = Unbundle By Name(w294) -> ("NormalGamePlay"=w293:refnum<class "NormalGamePlay.lvclass">)
            n148 = property class="NormalGamePlay"(reference=w293) -> (reference out=w292:refnum<class "NormalGamePlay.lvclass">, "Roles"=w303:T11)  [unwired: 1 in, 1 out]
            n149 = Increment(x=w297) -> (x+1=w296:i32)
            n150 = case shown="1, Default" w296 {
              tunnel: w303 -> [w309 w316]
              tunnel: [w307 w314] -> w302
              tunnel: w298 -> [w306 w313]
              tunnel: [w304 w311] -> w291
              frame 1, Default {
                n151 = Unbundle By Name(w309) -> ("ShootRole"=w310:refnum<class "ShootRole.lvclass">)
                n152 = property class="Robot"(reference=w306, "role"=roles."Shoot") -> (reference out=w304:refnum<class "Robot.lvclass">)  [unwired: 1 in, 1 out]
                n153 = property class="ShootRole"(reference=w310, "RobotRef"=w304) -> (reference out=w308:refnum<class "ShootRole.lvclass">)  [unwired: 1 in, 1 out]
                n154 = Bundle By Name(cluster=w309, "ShootRole"=w308) -> (w307:T11)
              }
              frame 2 {
                n155 = Unbundle By Name(w316) -> ("FollowAttackerRole"=w317:refnum<class "FollowAttackerRole.lvclass">)
                n156 = property class="Robot"(reference=w313, "role"=roles."FollowAttacker") -> (reference out=w311:refnum<class "Robot.lvclass">)  [unwired: 1 in, 1 out]
                n157 = property class="FollowAttackerRole"(reference=w317, "RobotRef"=w311) -> (reference out=w315:refnum<class "FollowAttackerRole.lvclass">)  [unwired: 1 in, 1 out]
                n158 = Bundle By Name(cluster=w316, "FollowAttackerRole"=w315) -> (w314:T11)
              }
            }
            n159 = property class="NormalGamePlay"(reference=w292, "Roles"=w302) -> (reference out=w301:refnum<class "NormalGamePlay.lvclass">)  [unwired: 1 in, 1 out]
            n160 = Bundle By Name(cluster=w294, "NormalGamePlay"=w301) -> (w295:T5)
            n161 = property class="Playbook"(reference=w300, "offensive_plays"=w295) -> (reference out=w299:refnum<class "Playbook.lvclass">)  [unwired: 1 in, 1 out]
          }
        }
        frame "5RobotsNormalGamePlay" {
          n162 = property class="Playbook"(reference=w321) -> (reference out=w330:refnum<class "Playbook.lvclass">, "offensive_plays"=w332:T5)  [unwired: 1 in, 1 out]
          n163 = Unbundle By Name(w320) -> ("TheBestKickers"=w319:i32[])
          n164 = Unbundle By Name(w332) -> ("5RobotsPassGamePlay"=w331:refnum<class "5RobotsPassGamePlay.lvclass">)
          n165 = property class="5RobotsPassGamePlay" props=["NumberOfRobots"](reference=w331) -> ()  [unwired: 1 in, 3 out]
          n166 = Array Size(array=w319) -> (size(s)=w318:i32)
          n167 = call-dynamic "pickOffensiveTeam.vi"("OffensiveTeam in"=w327, "Game"=w328, "KeeperTeam"=w325, "number_of_robots"=w318, "RobotRef"=w326) -> ("OffensiveTeam out"=w324:refnum<class "Ally.lvclass">, "RobotRef"=w329:refnum<class "Robot.lvclass">[])  [unwired: 8 in, 1 out]
          n168 = for {
            tunnel: [w336] -> w322 mode=indexing
            tunnel: w329 -> [w342] mode=indexing
            shift-right: [w343] -> w323
            shift-left: w330 -> [w344]
            shift-right: [w339] -> _
            shift-left: w332 -> [w338]
            i -> [w341]
            n169 = Unbundle By Name(w338) -> ("5RobotsNormalGamePlay"=w337:refnum<class "5RobotsNormalGamePlay.lvclass">)
            n170 = property class="5RobotsNormalGamePlay"(reference=w337) -> (reference out=w334:refnum<class "5RobotsNormalGamePlay.lvclass">, "Roles"=w345:T12)  [unwired: 1 in, 1 out]
            n171 = Increment(x=w341) -> (x+1=w340:i32)
            n172 = case shown="1, Default" w340 {
              tunnel: w345 -> [w351 w358 w365 w372 w379]
              tunnel: [w349 w356 w363 w370 w377] -> w333
              tunnel: w342 -> [w348 w355 w362 w369 w376]
              tunnel: [w346 w354 w361 w368 w375] -> w336
              frame 1, Default {
                n173 = Unbundle By Name(w351) -> ("ShootRole"=w352:refnum<class "ShootRole.lvclass">)
                n174 = property class="Robot"(reference=w348, "role"=roles."Shoot") -> (reference out=w346:refnum<class "Robot.lvclass">)  [unwired: 1 in, 1 out]
                n175 = property class="ShootRole"(reference=w352, "RobotRef"=w346) -> (reference out=w350:refnum<class "ShootRole.lvclass">)  [unwired: 1 in, 1 out]
                n176 = Bundle By Name(cluster=w351, "ShootRole"=w350) -> (w349:T12)
              }
              frame 2 {
                n177 = Unbundle By Name(w358) -> ("5RobotsRole1st"=w359:refnum<class "5RobotsRole.lvclass">)
                n178 = property class="Robot"(reference=w355, "role"=roles."5Robots1st") -> (reference out=w354:refnum<class "Robot.lvclass">)  [unwired: 1 in, 1 out]
                n179 = property class="5RobotsRole"(reference=w359, "RobotRef"=w354) -> (reference out=w357:refnum<class "5RobotsRole.lvclass">)  [unwired: 1 in, 1 out]
                n180 = Bundle By Name(cluster=w358, "5RobotsRole1st"=w357) -> (w356:T12)
              }
              frame 3 {
                n181 = Unbundle By Name(w365) -> ("5RobotsRole2nd"=w366:refnum<class "5RobotsRole.lvclass">)
                n182 = property class="Robot"(reference=w362, "role"=roles."5Robots2nd") -> (reference out=w361:refnum<class "Robot.lvclass">)  [unwired: 1 in, 1 out]
                n183 = property class="5RobotsRole"(reference=w366, "RobotRef"=w361) -> (reference out=w364:refnum<class "5RobotsRole.lvclass">)  [unwired: 1 in, 1 out]
                n184 = Bundle By Name(cluster=w365, "5RobotsRole2nd"=w364) -> (w363:T12)
              }
              frame 4 {
                n185 = Unbundle By Name(w372) -> ("5RobotsRole3rd"=w373:refnum<class "5RobotsRole.lvclass">)
                n186 = property class="Robot"(reference=w369, "role"=roles."5Robots3rd") -> (reference out=w368:refnum<class "Robot.lvclass">)  [unwired: 1 in, 1 out]
                n187 = property class="5RobotsRole"(reference=w373, "RobotRef"=w368) -> (reference out=w371:refnum<class "5RobotsRole.lvclass">)  [unwired: 1 in, 1 out]
                n188 = Bundle By Name(cluster=w372, "5RobotsRole3rd"=w371) -> (w370:T12)
              }
              frame 5 {
                n189 = Unbundle By Name(w379) -> ("5RobotsRole4th"=w380:refnum<class "5RobotsRole.lvclass">)
                n190 = property class="Robot"(reference=w376, "role"=roles."5Robots4th") -> (reference out=w375:refnum<class "Robot.lvclass">)  [unwired: 1 in, 1 out]
                n191 = property class="5RobotsRole"(reference=w380, "RobotRef"=w375) -> (reference out=w378:refnum<class "5RobotsRole.lvclass">)  [unwired: 1 in, 1 out]
                n192 = Bundle By Name(cluster=w379, "5RobotsRole4th"=w378) -> (w377:T12)
              }
            }
            n193 = property class="5RobotsNormalGamePlay"(reference=w334, "Roles"=w333) -> (reference out=w335:refnum<class "5RobotsNormalGamePlay.lvclass">)  [unwired: 1 in, 1 out]
            n194 = Bundle By Name(cluster=w338, "5RobotsNormalGamePlay"=w335) -> (w339:T5)
            n195 = property class="Playbook"(reference=w344, "offensive_plays"=w339) -> (reference out=w343:refnum<class "Playbook.lvclass">)  [unwired: 1 in, 1 out]
          }
        }
        frame "5PreparePassGame" {
          n196 = property class="Playbook"(reference=w384) -> (reference out=w393:refnum<class "Playbook.lvclass">, "offensive_plays"=w395:T5)  [unwired: 1 in, 1 out]
          n197 = Unbundle By Name(w383) -> ("TheBestKickers"=w382:i32[])
          n198 = Unbundle By Name(w395) -> ("5RobotsPassGamePlay"=w394:refnum<class "5RobotsPassGamePlay.lvclass">)
          n199 = property class="5RobotsPassGamePlay" props=["NumberOfRobots"](reference=w394) -> ()  [unwired: 1 in, 3 out]
          n200 = Array Size(array=w382) -> (size(s)=w381:i32)
          n201 = call-dynamic "pickOffensiveTeam.vi"("OffensiveTeam in"=w390, "Game"=w391, "KeeperTeam"=w388, "number_of_robots"=w381, "RobotRef"=w389) -> ("OffensiveTeam out"=w387:refnum<class "Ally.lvclass">, "RobotRef"=w392:refnum<class "Robot.lvclass">[])  [unwired: 8 in, 1 out]
          n202 = for {
            tunnel: [w399] -> w385 mode=indexing
            tunnel: w392 -> [w405] mode=indexing
            shift-right: [w406] -> w386
            shift-left: w393 -> [w407]
            shift-right: [w402] -> _
            shift-left: w395 -> [w401]
            i -> [w404]
            n203 = Unbundle By Name(w401) -> ("5PreparePassGamePlay"=w400:refnum<class "5PreparePassGamePlay.lvclass">)
            n204 = property class="5PreparePassGamePlay"(reference=w400) -> (reference out=w397:refnum<class "5PreparePassGamePlay.lvclass">, "Roles"=w408:T13)  [unwired: 1 in, 1 out]
            n205 = Increment(x=w404) -> (x+1=w403:i32)
            n206 = case shown="5" w403 {
              tunnel: w408 -> [w414 w421 w428 w435 w442]
              tunnel: [w412 w419 w426 w433 w440] -> w396
              tunnel: w405 -> [w411 w418 w425 w432 w439]
              tunnel: [w409 w417 w424 w431 w438] -> w399
              frame 1, Default {
                n207 = Unbundle By Name(w414) -> ("AttackerStopRole"=w415:refnum<class "AttackerStopRole.lvclass">)
                n208 = property class="Robot"(reference=w411, "role"=roles."AttackerStop") -> (reference out=w409:refnum<class "Robot.lvclass">)  [unwired: 1 in, 1 out]
                n209 = property class="AttackerStopRole"(reference=w415, "RobotRef"=w409) -> (reference out=w413:refnum<class "AttackerStopRole.lvclass">)  [unwired: 1 in, 1 out]
                n210 = Bundle By Name(cluster=w414, "AttackerStopRole"=w413) -> (w412:T13)
              }
              frame 2 {
                n211 = Unbundle By Name(w421) -> ("5RobotsRole1st"=w422:refnum<class "5RobotsRole.lvclass">)
                n212 = property class="Robot"(reference=w418, "role"=roles."5Robots1st") -> (reference out=w417:refnum<class "Robot.lvclass">)  [unwired: 1 in, 1 out]
                n213 = property class="5RobotsRole"(reference=w422, "RobotRef"=w417) -> (reference out=w420:refnum<class "5RobotsRole.lvclass">)  [unwired: 1 in, 1 out]
                n214 = Bundle By Name(cluster=w421, "5RobotsRole1st"=w420) -> (w419:T13)
              }
              frame 3 {
                n215 = Unbundle By Name(w428) -> ("5RobotsRole2nd"=w429:refnum<class "5RobotsRole.lvclass">)
                n216 = property class="Robot"(reference=w425, "role"=roles."5Robots2nd") -> (reference out=w424:refnum<class "Robot.lvclass">)  [unwired: 1 in, 1 out]
                n217 = property class="5RobotsRole"(reference=w429, "RobotRef"=w424) -> (reference out=w427:refnum<class "5RobotsRole.lvclass">)  [unwired: 1 in, 1 out]
                n218 = Bundle By Name(cluster=w428, "5RobotsRole2nd"=w427) -> (w426:T13)
              }
              frame 4 {
                n219 = Unbundle By Name(w435) -> ("5RobotsRole3rd"=w436:refnum<class "5RobotsRole.lvclass">)
                n220 = property class="Robot"(reference=w432, "role"=roles."5Robots3rd") -> (reference out=w431:refnum<class "Robot.lvclass">)  [unwired: 1 in, 1 out]
                n221 = property class="5RobotsRole"(reference=w436, "RobotRef"=w431) -> (reference out=w434:refnum<class "5RobotsRole.lvclass">)  [unwired: 1 in, 1 out]
                n222 = Bundle By Name(cluster=w435, "5RobotsRole3rd"=w434) -> (w433:T13)
              }
              frame 5 {
                n223 = Unbundle By Name(w442) -> ("5RobotsRole4th"=w443:refnum<class "5RobotsRole.lvclass">)
                n224 = property class="Robot"(reference=w439, "role"=roles."5Robots4th") -> (reference out=w438:refnum<class "Robot.lvclass">)  [unwired: 1 in, 1 out]
                n225 = property class="5RobotsRole"(reference=w443, "RobotRef"=w438) -> (reference out=w441:refnum<class "5RobotsRole.lvclass">)  [unwired: 1 in, 1 out]
                n226 = Bundle By Name(cluster=w442, "5RobotsRole4th"=w441) -> (w440:T13)
              }
            }
            n227 = property class="5PreparePassGamePlay"(reference=w397, "Roles"=w396) -> (reference out=w398:refnum<class "5PreparePassGamePlay.lvclass">)  [unwired: 1 in, 1 out]
            n228 = Bundle By Name(cluster=w401, "5PreparePassGamePlay"=w398) -> (w402:T5)
            n229 = property class="Playbook"(reference=w407, "offensive_plays"=w402) -> (reference out=w406:refnum<class "Playbook.lvclass">)  [unwired: 1 in, 1 out]
          }
        }
        frame "5RobotsPassGamePlay" {
          n230 = property class="Playbook"(reference=w447) -> (reference out=w456:refnum<class "Playbook.lvclass">, "offensive_plays"=w458:T5)  [unwired: 1 in, 1 out]
          n231 = Unbundle By Name(w446) -> ("TheBestKickers"=w445:i32[])
          n232 = Unbundle By Name(w458) -> ("5RobotsPassGamePlay"=w457:refnum<class "5RobotsPassGamePlay.lvclass">)
          n233 = property class="5RobotsPassGamePlay" props=["NumberOfRobots"](reference=w457) -> ()  [unwired: 1 in, 3 out]
          n234 = Array Size(array=w445) -> (size(s)=w444:i32)
          n235 = call-dynamic "pickOffensiveTeam.vi"("OffensiveTeam in"=w453, "Game"=w454, "KeeperTeam"=w451, "number_of_robots"=w444, "RobotRef"=w452) -> ("OffensiveTeam out"=w450:refnum<class "Ally.lvclass">, "RobotRef"=w455:refnum<class "Robot.lvclass">[])  [unwired: 8 in, 1 out]
          n236 = for {
            tunnel: [w462] -> w448 mode=indexing
            tunnel: w455 -> [w468] mode=indexing
            shift-right: [w469] -> w449
            shift-left: w456 -> [w470]
            shift-right: [w465] -> _
            shift-left: w458 -> [w464]
            i -> [w467]
            n237 = Unbundle By Name(w464) -> ("5RobotsPassGamePlay"=w463:refnum<class "5RobotsPassGamePlay.lvclass">)
            n238 = property class="5RobotsPassGamePlay"(reference=w463) -> (reference out=w460:refnum<class "5RobotsPassGamePlay.lvclass">, "Roles"=w471:T14)  [unwired: 1 in, 1 out]
            n239 = Increment(x=w467) -> (x+1=w466:i32)
            n240 = case shown="2" w466 {
              tunnel: w471 -> [w477 w484 w491 w498 w505]
              tunnel: [w475 w482 w489 w496 w503] -> w459
              tunnel: w468 -> [w474 w481 w488 w495 w502]
              tunnel: [w472 w479 w487 w494 w501] -> w462
              frame 1, Default {
                n241 = Unbundle By Name(w477) -> ("PassBestRobotRole"=w478:refnum<class "PassBestRobotRole.lvclass">)
                n242 = property class="Robot"(reference=w474, "role"=roles."PassBestRobot") -> (reference out=w472:refnum<class "Robot.lvclass">)  [unwired: 1 in, 1 out]
                n243 = property class="PassBestRobotRole"(reference=w478, "RobotRef"=w472) -> (reference out=w476:refnum<class "PassBestRobotRole.lvclass">)  [unwired: 1 in, 1 out]
                n244 = Bundle By Name(cluster=w477, "PassBestRobotRole"=w476) -> (w475:T14)
              }
              frame 2 {
                n245 = Unbundle By Name(w484) -> ("PassBestReceiverRole"=w485:refnum<class "PassBestReceiverRole.lvclass">)
                n246 = property class="Robot"(reference=w481, "role"=roles."PassBestReceiver") -> (reference out=w479:refnum<class "Robot.lvclass">)  [unwired: 1 in, 1 out]
                n247 = property class="PassBestReceiverRole"(reference=w485, "RobotRef"=w479) -> (reference out=w483:refnum<class "PassBestReceiverRole.lvclass">)  [unwired: 1 in, 1 out]
                n248 = Bundle By Name(cluster=w484, "PassBestReceiverRole"=w483) -> (w482:T14)
              }
              frame 3 {
                n249 = Unbundle By Name(w491) -> ("5RobotsRole1st"=w492:refnum<class "5RobotsRole.lvclass">)
                n250 = property class="Robot"(reference=w488, "role"=roles."5Robots1st") -> (reference out=w487:refnum<class "Robot.lvclass">)  [unwired: 1 in, 1 out]
                n251 = property class="5RobotsRole"(reference=w492, "RobotRef"=w487) -> (reference out=w490:refnum<class "5RobotsRole.lvclass">)  [unwired: 1 in, 1 out]
                n252 = Bundle By Name(cluster=w491, "5RobotsRole1st"=w490) -> (w489:T14)
              }
              frame 4 {
                n253 = Unbundle By Name(w498) -> ("5RobotsRole2nd"=w499:refnum<class "5RobotsRole.lvclass">)
                n254 = property class="Robot"(reference=w495, "role"=roles."5Robots2nd") -> (reference out=w494:refnum<class "Robot.lvclass">)  [unwired: 1 in, 1 out]
                n255 = property class="5RobotsRole"(reference=w499, "RobotRef"=w494) -> (reference out=w497:refnum<class "5RobotsRole.lvclass">)  [unwired: 1 in, 1 out]
                n256 = Bundle By Name(cluster=w498, "5RobotsRole2nd"=w497) -> (w496:T14)
              }
              frame 5 {
                n257 = Unbundle By Name(w505) -> ("5RobotsRole3rd"=w506:refnum<class "5RobotsRole.lvclass">)
                n258 = property class="Robot"(reference=w502, "role"=roles."5Robots3rd") -> (reference out=w501:refnum<class "Robot.lvclass">)  [unwired: 1 in, 1 out]
                n259 = property class="5RobotsRole"(reference=w506, "RobotRef"=w501) -> (reference out=w504:refnum<class "5RobotsRole.lvclass">)  [unwired: 1 in, 1 out]
                n260 = Bundle By Name(cluster=w505, "5RobotsRole3rd"=w504) -> (w503:T14)
              }
            }
            n261 = property class="5RobotsPassGamePlay"(reference=w460, "Roles"=w459) -> (reference out=w461:refnum<class "5RobotsPassGamePlay.lvclass">)  [unwired: 1 in, 1 out]
            n262 = Bundle By Name(cluster=w464, "5RobotsPassGamePlay"=w461) -> (w465:T5)
            n263 = property class="Playbook"(reference=w470, "offensive_plays"=w465) -> (reference out=w469:refnum<class "Playbook.lvclass">)  [unwired: 1 in, 1 out]
          }
        }
        frame "PrepareKeeperPass" {
          n264 = property class="Playbook"(reference=w519) -> (reference out=w512:refnum<class "Playbook.lvclass">, "offensive_plays"=w518:T5)  [unwired: 1 in, 1 out]
          n265 = Unbundle By Name(w518) -> ("PrepareKeeperPassPlay"=w515:refnum<class "PrepareKeeperPassPlay.lvclass">)
          n266 = property class="PrepareKeeperPassPlay"(reference=w515) -> ("NumberOfRobots"=w514:dbl)  [unwired: 1 in, 2 out]
          n267 = call-dynamic "pickOffensiveTeam.vi"("OffensiveTeam in"=w508, "Game"=w507, "KeeperTeam"=w509, "number_of_robots"=w514, "RobotRef"=w513) -> ("OffensiveTeam out"=w510:refnum<class "Ally.lvclass">, "RobotRef"=w511:refnum<class "Robot.lvclass">[])  [unwired: 8 in, 1 out]
          n268 = for {
            tunnel: [w520] -> w516 mode=indexing
            tunnel: w511 -> [w527] mode=indexing
            shift-right: [w528] -> w517
            shift-left: w512 -> [w529]
            shift-right: [w524] -> _
            shift-left: w518 -> [w523]
            i -> [w526]
            n269 = Unbundle By Name(w523) -> ("PrepareKeeperPassPlay"=w522:refnum<class "PrepareKeeperPassPlay.lvclass">)
            n270 = property class="PrepareKeeperPassPlay"(reference=w522) -> (reference out=w521:refnum<class "PrepareKeeperPassPlay.lvclass">, "Roles"=w532:T15)  [unwired: 1 in, 1 out]
            n271 = Increment(x=w526) -> (x+1=w525:i32)
            n272 = case shown="1, Default" w525 {
              tunnel: w532 -> [w538 w545]
              tunnel: [w536 w543] -> w531
              tunnel: w527 -> [w535 w542]
              tunnel: [w533 w540] -> w520
              frame 1, Default {
                n273 = Unbundle By Name(w538) -> ("PreparePassReceiverRole1"=w539:refnum<class "PreparePassReceiverRole.lvclass">)
                n274 = property class="Robot"(reference=w535, "role"=roles."PreparePassReceiver 1") -> (reference out=w533:refnum<class "Robot.lvclass">)  [unwired: 1 in, 1 out]
                n275 = property class="PreparePassReceiverRole"(reference=w539, "RobotRef"=w533) -> (reference out=w537:refnum<class "PreparePassReceiverRole.lvclass">)  [unwired: 1 in, 1 out]
                n276 = Bundle By Name(cluster=w538, "PreparePassReceiverRole1"=w537) -> (w536:T15)
              }
              frame 2 {
                n277 = Unbundle By Name(w545) -> ("PreparePassReceiverRole 2"=w546:refnum<class "PreparePassReceiverRole.lvclass">)
                n278 = property class="Robot"(reference=w542, "role"=roles."PreparePassReceiver 2") -> (reference out=w540:refnum<class "Robot.lvclass">)  [unwired: 1 in, 1 out]
                n279 = property class="PreparePassReceiverRole"(reference=w546, "RobotRef"=w540) -> (reference out=w544:refnum<class "PreparePassReceiverRole.lvclass">)  [unwired: 1 in, 1 out]
                n280 = Bundle By Name(cluster=w545, "PreparePassReceiverRole 2"=w544) -> (w543:T15)
              }
            }
            n281 = property class="PrepareKeeperPassPlay"(reference=w521, "Roles"=w531) -> (reference out=w530:refnum<class "PrepareKeeperPassPlay.lvclass">)  [unwired: 1 in, 1 out]
            n282 = Bundle By Name(cluster=w523, "PrepareKeeperPassPlay"=w530) -> (w524:T5)
            n283 = property class="Playbook"(reference=w529, "offensive_plays"=w524) -> (reference out=w528:refnum<class "Playbook.lvclass">)  [unwired: 1 in, 1 out]
          }
        }
        frame "PreparePassInGame1" {
          n284 = property class="Playbook"(reference=w559) -> (reference out=w552:refnum<class "Playbook.lvclass">, "offensive_plays"=w558:T5)  [unwired: 1 in, 1 out]
          n285 = Unbundle By Name(w558) -> ("PreparePassInGame1"=w555:refnum<class "PreparePassInGame1.lvclass">)
          n286 = property class="PreparePassInGame1"(reference=w555) -> ("NumberOfRobots"=w554:dbl)  [unwired: 1 in, 2 out]
          n287 = call-dynamic "pickOffensiveTeam.vi"("OffensiveTeam in"=w548, "Game"=w547, "KeeperTeam"=w549, "number_of_robots"=w554, "RobotRef"=w553) -> ("OffensiveTeam out"=w550:refnum<class "Ally.lvclass">, "RobotRef"=w551:refnum<class "Robot.lvclass">[])  [unwired: 8 in, 1 out]
          n288 = for {
            tunnel: [w560] -> w556 mode=indexing
            tunnel: w551 -> [w567] mode=indexing
            shift-right: [w568] -> w557
            shift-left: w552 -> [w569]
            shift-right: [w564] -> _
            shift-left: w558 -> [w563]
            i -> [w566]
            n289 = Unbundle By Name(w563) -> ("PreparePassInGame1"=w562:refnum<class "PreparePassInGame1.lvclass">)
            n290 = property class="PreparePassInGame1"(reference=w562) -> (reference out=w561:refnum<class "PreparePassInGame1.lvclass">, "Roles"=w572:T16)  [unwired: 1 in, 1 out]
            n291 = Increment(x=w566) -> (x+1=w565:i32)
            n292 = case shown="1, Default" w565 {
              tunnel: w572 -> [w578 w585 w592]
              tunnel: [w576 w583 w590] -> w571
              tunnel: w567 -> [w575 w582 w589]
              tunnel: [w573 w580 w587] -> w560
              frame 1, Default {
                n293 = Unbundle By Name(w578) -> ("ShootRole"=w579:refnum<class "ShootRole.lvclass">)
                n294 = property class="Robot"(reference=w575, "role"=roles."Shoot") -> (reference out=w573:refnum<class "Robot.lvclass">)  [unwired: 1 in, 1 out]
                n295 = property class="ShootRole"(reference=w579, "RobotRef"=w573) -> (reference out=w577:refnum<class "ShootRole.lvclass">)  [unwired: 1 in, 1 out]
                n296 = Bundle By Name(cluster=w578, "ShootRole"=w577) -> (w576:T16)
              }
              frame 2 {
                n297 = Unbundle By Name(w585) -> ("PreparePassReceiverRole1"=w586:refnum<class "PreparePassReceiverRole.lvclass">)
                n298 = property class="Robot"(reference=w582, "role"=roles."PreparePassReceiver 1") -> (reference out=w580:refnum<class "Robot.lvclass">)  [unwired: 1 in, 1 out]
                n299 = property class="PreparePassReceiverRole"(reference=w586, "RobotRef"=w580) -> (reference out=w584:refnum<class "PreparePassReceiverRole.lvclass">)  [unwired: 1 in, 1 out]
                n300 = Bundle By Name(cluster=w585, "PreparePassReceiverRole1"=w584) -> (w583:T16)
              }
              frame 3 {
                n301 = Unbundle By Name(w592) -> ("PreparePassReceiverRole2"=w593:refnum<class "PreparePassReceiverRole.lvclass">)
                n302 = property class="Robot"(reference=w589, "role"=roles."PreparePassReceiver 2") -> (reference out=w587:refnum<class "Robot.lvclass">)  [unwired: 1 in, 1 out]
                n303 = property class="PreparePassReceiverRole"(reference=w593, "RobotRef"=w587) -> (reference out=w591:refnum<class "PreparePassReceiverRole.lvclass">)  [unwired: 1 in, 1 out]
                n304 = Bundle By Name(cluster=w592, "PreparePassReceiverRole2"=w591) -> (w590:T16)
              }
            }
            n305 = property class="PreparePassInGame1"(reference=w561, "Roles"=w571) -> (reference out=w570:refnum<class "PreparePassInGame1.lvclass">)  [unwired: 1 in, 1 out]
            n306 = Bundle By Name(cluster=w563, "PreparePassInGame1"=w570) -> (w564:T5)
            n307 = property class="Playbook"(reference=w569, "offensive_plays"=w564) -> (reference out=w568:refnum<class "Playbook.lvclass">)  [unwired: 1 in, 1 out]
          }
        }
        frame "Halt" {
          n308 = property class="Playbook"(reference=w608) -> (reference out=w604:refnum<class "Playbook.lvclass">, "offensive_plays"=w607:T5)  [unwired: 1 in, 1 out]
          n309 = Array Size(array=w598) -> (size(s)=w596:i32)
          n310 = Array Size(array=w597) -> (size(s)=w595:i32)
          n311 = Subtract(x=w596, y=w595) -> (x-y=w594:i32)
          n312 = call-dynamic "pickOffensiveTeam.vi"("OffensiveTeam in"=w600, "Game"=w599, "KeeperTeam"=w601, "number_of_robots"=w594, "RobotRef"=w598) -> ("OffensiveTeam out"=w602:refnum<class "Ally.lvclass">, "RobotRef"=w603:refnum<class "Robot.lvclass">[])  [unwired: 8 in, 1 out]
          n313 = for {
            tunnel: [w609] -> w605 mode=indexing
            tunnel: w603 -> [w615] mode=indexing
            shift-right: [w616] -> w606
            shift-left: w604 -> [w617]
            shift-right: [w612] -> _
            shift-left: w607 -> [w611]
            i -> [w614]
            n314 = Unbundle By Name(w611) -> ("HaltPlay"=w610:refnum<class "HaltPlay.lvclass">)
            n315 = property class="HaltPlay"(reference=w610) -> (reference out=w619:refnum<class "HaltPlay.lvclass">, "Roles"=w621:T17)  [unwired: 1 in, 1 out]
            n316 = Increment(x=w614) -> (x+1=w613:i32)
            n317 = case shown="6" w613 {
              tunnel: w621 -> [w627 w634 w641 w648 w655 w662]
              tunnel: [w625 w632 w639 w646 w653 w660] -> w620
              tunnel: w615 -> [w624 w631 w638 w645 w652 w659]
              tunnel: [w622 w629 w636 w643 w650 w657] -> w609
              frame 1, Default {
                n318 = Unbundle By Name(w627) -> ("HaltRole 1"=w628:refnum<class "HaltRole.lvclass">)
                n319 = property class="Robot"(reference=w624, "role"=roles."Halt") -> (reference out=w622:refnum<class "Robot.lvclass">)  [unwired: 1 in, 1 out]
                n320 = property class="HaltRole"(reference=w628, "RobotRef"=w622) -> (reference out=w626:refnum<class "HaltRole.lvclass">)  [unwired: 1 in, 1 out]
                n321 = Bundle By Name(cluster=w627, "HaltRole 1"=w626) -> (w625:T17)
              }
              frame 2 {
                n322 = Unbundle By Name(w634) -> ("HaltRole 2"=w635:refnum<class "HaltRole.lvclass">)
                n323 = property class="Robot"(reference=w631, "role"=roles."Halt") -> (reference out=w629:refnum<class "Robot.lvclass">)  [unwired: 1 in, 1 out]
                n324 = property class="HaltRole"(reference=w635, "RobotRef"=w629) -> (reference out=w633:refnum<class "HaltRole.lvclass">)  [unwired: 1 in, 1 out]
                n325 = Bundle By Name(cluster=w634, "HaltRole 2"=w633) -> (w632:T17)
              }
              frame 3 {
                n326 = Unbundle By Name(w641) -> ("HaltRole 3"=w642:refnum<class "HaltRole.lvclass">)
                n327 = property class="Robot"(reference=w638, "role"=roles."Halt") -> (reference out=w636:refnum<class "Robot.lvclass">)  [unwired: 1 in, 1 out]
                n328 = property class="HaltRole"(reference=w642, "RobotRef"=w636) -> (reference out=w640:refnum<class "HaltRole.lvclass">)  [unwired: 1 in, 1 out]
                n329 = Bundle By Name(cluster=w641, "HaltRole 3"=w640) -> (w639:T17)
              }
              frame 4 {
                n330 = Unbundle By Name(w648) -> ("HaltRole 4"=w649:refnum<class "HaltRole.lvclass">)
                n331 = property class="Robot"(reference=w645, "role"=roles."Halt") -> (reference out=w643:refnum<class "Robot.lvclass">)  [unwired: 1 in, 1 out]
                n332 = property class="HaltRole"(reference=w649, "RobotRef"=w643) -> (reference out=w647:refnum<class "HaltRole.lvclass">)  [unwired: 1 in, 1 out]
                n333 = Bundle By Name(cluster=w648, "HaltRole 4"=w647) -> (w646:T17)
              }
              frame 5 {
                n334 = Unbundle By Name(w655) -> ("HaltRole 5"=w656:refnum<class "HaltRole.lvclass">)
                n335 = property class="Robot"(reference=w652, "role"=roles."Halt") -> (reference out=w650:refnum<class "Robot.lvclass">)  [unwired: 1 in, 1 out]
                n336 = property class="HaltRole"(reference=w656, "RobotRef"=w650) -> (reference out=w654:refnum<class "HaltRole.lvclass">)  [unwired: 1 in, 1 out]
                n337 = Bundle By Name(cluster=w655, "HaltRole 5"=w654) -> (w653:T17)
              }
              frame 6 {
                n338 = Unbundle By Name(w662) -> ("HaltRole 6"=w663:refnum<class "HaltRole.lvclass">)
                n339 = property class="Robot"(reference=w659, "role"=roles."Halt") -> (reference out=w657:refnum<class "Robot.lvclass">)  [unwired: 1 in, 1 out]
                n340 = property class="HaltRole"(reference=w663, "RobotRef"=w657) -> (reference out=w661:refnum<class "HaltRole.lvclass">)  [unwired: 1 in, 1 out]
                n341 = Bundle By Name(cluster=w662, "HaltRole 6"=w661) -> (w660:T17)
              }
            }
            n342 = property class="HaltPlay"(reference=w619, "Roles"=w620) -> (reference out=w618:refnum<class "HaltPlay.lvclass">)  [unwired: 1 in, 1 out]
            n343 = Bundle By Name(cluster=w611, "HaltPlay"=w618) -> (w612:T5)
            n344 = property class="Playbook"(reference=w617, "offensive_plays"=w612) -> (reference out=w616:refnum<class "Playbook.lvclass">)  [unwired: 1 in, 1 out]
          }
        }
        frame "BallOutOfField" {
          n345 = property class="Playbook"(reference=w676) -> (reference out=w669:refnum<class "Playbook.lvclass">, "offensive_plays"=w675:T5)  [unwired: 1 in, 1 out]
          n346 = Unbundle By Name(w675) -> ("BallOutOfFieldPlay"=w672:refnum<class "BallOutOfFieldPlay.lvclass">)
          n347 = property class="BallOutOfFieldPlay"(reference=w672) -> ("NumberOfRobots"=w671:dbl)  [unwired: 1 in, 2 out]
          n348 = call-dynamic "pickOffensiveTeam.vi"("OffensiveTeam in"=w665, "Game"=w664, "KeeperTeam"=w666, "number_of_robots"=w671, "RobotRef"=w670) -> ("OffensiveTeam out"=w667:refnum<class "Ally.lvclass">, "RobotRef"=w668:refnum<class "Robot.lvclass">[])  [unwired: 8 in, 1 out]
          n349 = for {
            tunnel: [w677] -> w673 mode=indexing
            tunnel: w668 -> [w683] mode=indexing
            shift-right: [w684] -> w674
            shift-left: w669 -> [w685]
            shift-right: [w680] -> _
            shift-left: w675 -> [w679]
            i -> [w682]
            n350 = Unbundle By Name(w679) -> ("BallOutOfFieldPlay"=w678:refnum<class "BallOutOfFieldPlay.lvclass">)
            n351 = property class="BallOutOfFieldPlay"(reference=w678) -> (reference out=w687:refnum<class "BallOutOfFieldPlay.lvclass">, "Roles"=w689:T18)  [unwired: 1 in, 1 out]
            n352 = Increment(x=w682) -> (x+1=w681:i32)
            n353 = case shown="2" w681 {
              tunnel: w689 -> [w695 w702]
              tunnel: [w693 w700] -> w688
              tunnel: w683 -> [w692 w698]
              tunnel: [w690 w697] -> w677
              frame 1, Default {
                n354 = Unbundle By Name(w695) -> ("BallOutOfFieldRole"=w696:refnum<class "BallOutOfFieldRole.lvclass">)
                n355 = property class="Robot"(reference=w692, "role"=roles."BallOutOfField") -> (reference out=w690:refnum<class "Robot.lvclass">)  [unwired: 1 in, 1 out]
                n356 = property class="BallOutOfFieldRole"(reference=w696, "RobotRef"=w690) -> (reference out=w694:refnum<class "BallOutOfFieldRole.lvclass">)  [unwired: 1 in, 1 out]
                n357 = Bundle By Name(cluster=w695, "BallOutOfFieldRole"=w694) -> (w693:T18)
              }
              frame 2 {
                n358 = Unbundle By Name(w702) -> ("FollowAttackerRole"=w703:refnum<class "FollowAttackerRole.lvclass">)
                n359 = property class="Robot"(reference=w698, "role"=roles."FollowAttacker") -> (reference out=w697:refnum<class "Robot.lvclass">)  [unwired: 1 in, 1 out]
                n360 = property class="FollowAttackerRole"(reference=w703, "RobotRef"=w697) -> (reference out=w701:refnum<class "FollowAttackerRole.lvclass">)  [unwired: 1 in, 1 out]
                n361 = Bundle By Name(cluster=w702, "FollowAttackerRole"=w701) -> (w700:T18)
              }
            }
            n362 = property class="BallOutOfFieldPlay"(reference=w687, "Roles"=w688) -> (reference out=w686:refnum<class "BallOutOfFieldPlay.lvclass">)  [unwired: 1 in, 1 out]
            n363 = Bundle By Name(cluster=w679, "BallOutOfFieldPlay"=w686) -> (w680:T5)
            n364 = property class="Playbook"(reference=w685, "offensive_plays"=w680) -> (reference out=w684:refnum<class "Playbook.lvclass">)  [unwired: 1 in, 1 out]
          }
        }
        frame "StopOffensive" {
          n365 = property class="Game"(reference=w718) -> ("EnemyRef"=w721:refnum<class "Enemy.lvclass">, "NewParameters"=w719:T2)  [unwired: 1 in, 2 out]
          n366 = property class="Playbook"(reference=w732) -> (reference out=w726:refnum<class "Playbook.lvclass">, "offensive_plays"=w731:T5)  [unwired: 1 in, 1 out]
          n367 = Unbundle By Name(w719) -> ("NumberOfMarkers"=w714:dbl)
          n368 = property class="Enemy"(reference=w721) -> ("RobotRef"=w720:refnum<class "Robot.lvclass">[])  [unwired: 1 in, 2 out]
          n369 = Array Size(array=w720) -> (size(s)=w716:i32)
          n370 = call "deleteImpossibleEnemiesToMark.vi"("Game"=w712, "MarkerSkill in"=refnum<class "MarkerSkill.lvclass"> refnum) -> ("PossibleEnemiesToMark"=w710:refnum<class "Enemy.lvclass">)  [unwired: 6 in, 3 out]
          n371 = Unbundle By Name(w731) -> ("StopOffensivePlay"=w728:refnum<class "StopOffensivePlay.lvclass">)
          n372 = property class="StopOffensivePlay" props=["NumberOfRobots"](reference=w728) -> ()  [unwired: 1 in, 3 out]
          n373 = Decrement(x=w716) -> (x-1=w715:i32)
          n374 = property class="Enemy"(reference=w710) -> ("RobotRef"=w709:refnum<class "Robot.lvclass">[])  [unwired: 1 in, 2 out]
          n375 = Greater?(x=w715, y=w714) -> (0:w717:bool)
          n376 = Increment(x=w714) -> (x+1=w713:dbl)
          n377 = Select(t=w713, s=w717, f=w715) -> (s? t:f=w705:dbl)
          n378 = Array Size(array=w709) -> (size(s)=w708:i32)
          n379 = Increment(x=w708) -> (x+1=w706:i32)
          n380 = Greater?(x=w705, y=w706) -> (0:w707:bool)
          n381 = Select(t=w706, s=w707, f=w705) -> (s? t:f=w704:dbl)
          n382 = call-dynamic "pickOffensiveTeam.vi"("OffensiveTeam in"=w722, "Game"=w718, "KeeperTeam"=w723, "number_of_robots"=w704, "RobotRef"=w727) -> ("OffensiveTeam out"=w724:refnum<class "Ally.lvclass">, "RobotRef"=w725:refnum<class "Robot.lvclass">[])  [unwired: 8 in, 1 out]
          n383 = for {
            tunnel: [w733] -> w729 mode=indexing
            tunnel: w725 -> [w739] mode=indexing
            shift-right: [w740] -> w730
            shift-left: w726 -> [w741]
            shift-right: [w736] -> _
            shift-left: w731 -> [w735]
            i -> [w738]
            n384 = Unbundle By Name(w735) -> ("StopOffensivePlay"=w734:refnum<class "StopOffensivePlay.lvclass">)
            n385 = property class="StopOffensivePlay"(reference=w734) -> (reference out=w743:refnum<class "StopOffensivePlay.lvclass">, "Roles"=w745:T19)  [unwired: 1 in, 1 out]
            n386 = Increment(x=w738) -> (x+1=w737:i32)
            n387 = case shown="2, Default" w737 {
              tunnel: w745 -> [w751 w758]
              tunnel: [w749 w756] -> w744
              tunnel: w739 -> [w748 w754]
              tunnel: [w746 w753] -> w733
              frame 1 {
                n388 = Unbundle By Name(w751) -> ("AttackerStopRole"=w752:refnum<class "AttackerStopRole.lvclass">)
                n389 = property class="Robot"(reference=w748, "role"=roles."AttackerStop") -> (reference out=w746:refnum<class "Robot.lvclass">)  [unwired: 1 in, 1 out]
                n390 = property class="AttackerStopRole"(reference=w752, "RobotRef"=w746) -> (reference out=w750:refnum<class "AttackerStopRole.lvclass">)  [unwired: 1 in, 1 out]
                n391 = Bundle By Name(cluster=w751, "AttackerStopRole"=w750) -> (w749:T19)
              }
              frame 2, Default {
                n392 = Unbundle By Name(w758) -> ("MarkerRole"=w759:refnum<class "MarkerRole.lvclass">)
                n393 = property class="Robot"(reference=w754, "role"=roles."Marker") -> (reference out=w753:refnum<class "Robot.lvclass">)  [unwired: 1 in, 1 out]
                n394 = property class="MarkerRole"(reference=w759, "RobotRef"=w753) -> (reference out=w757:refnum<class "MarkerRole.lvclass">)  [unwired: 1 in, 1 out]
                n395 = Bundle By Name(cluster=w758, "MarkerRole"=w757) -> (w756:T19)
              }
            }
            n396 = property class="StopOffensivePlay"(reference=w743, "Roles"=w744) -> (reference out=w742:refnum<class "StopOffensivePlay.lvclass">)  [unwired: 1 in, 1 out]
            n397 = Bundle By Name(cluster=w735, "StopOffensivePlay"=w742) -> (w736:T5)
            n398 = property class="Playbook"(reference=w741, "offensive_plays"=w736) -> (reference out=w740:refnum<class "Playbook.lvclass">)  [unwired: 1 in, 1 out]
          }
        }
        frame "EnemyPossesionAtOurField" {
          n399 = property class="Playbook"(reference=w772) -> (reference out=w766:refnum<class "Playbook.lvclass">, "offensive_plays"=w771:T5)  [unwired: 1 in, 1 out]
          n400 = Unbundle By Name(w771) -> ("EnemyPossessionAtOurFieldPlay"=w768:refnum<class "EnemyPossessionAtOurFieldPlay.lvclass">)
          n401 = property class="EnemyPossessionAtOurFieldPlay"(reference=w768) -> ("NumberOfRobots"=w760:dbl)  [unwired: 1 in, 2 out]
          n402 = call-dynamic "pickOffensiveTeam.vi"("OffensiveTeam in"=w762, "Game"=w761, "KeeperTeam"=w763, "number_of_robots"=w760, "RobotRef"=w767) -> ("OffensiveTeam out"=w764:refnum<class "Ally.lvclass">, "RobotRef"=w765:refnum<class "Robot.lvclass">[])  [unwired: 8 in, 1 out]
          n403 = for {
            tunnel: [w773] -> w769 mode=indexing
            tunnel: w765 -> [w779] mode=indexing
            shift-right: [w780] -> w770
            shift-left: w766 -> [w781]
            shift-right: [w776] -> _
            shift-left: w771 -> [w775]
            i -> [w778]
            # "Pode ter mais de um robô nesse\ncase. \nVários podem receber a role\nde marker"
            n404 = Unbundle By Name(w775) -> ("EnemyPossessionAtOurFieldPlay"=w774:refnum<class "EnemyPossessionAtOurFieldPlay.lvclass">)
            n405 = property class="EnemyPossessionAtOurFieldPlay"(reference=w774) -> (reference out=w783:refnum<class "EnemyPossessionAtOurFieldPlay.lvclass">, "Roles"=w785:T20)  [unwired: 1 in, 1 out]
            n406 = Increment(x=w778) -> (x+1=w777:i32)
            n407 = case shown="2, Default" w777 {
              tunnel: w785 -> [w791 w798]
              tunnel: [w789 w796] -> w784
              tunnel: w779 -> [w788 w794]
              tunnel: [w786 w793] -> w773
              frame 1 {
                n408 = Unbundle By Name(w791) -> ("ShootRole"=w792:refnum<class "ShootRole.lvclass">)
                n409 = property class="Robot"(reference=w788, "role"=roles."Shoot") -> (reference out=w786:refnum<class "Robot.lvclass">)  [unwired: 1 in, 1 out]
                n410 = property class="ShootRole"(reference=w792, "RobotRef"=w786) -> (reference out=w790:refnum<class "ShootRole.lvclass">)  [unwired: 1 in, 1 out]
                n411 = Bundle By Name(cluster=w791, "ShootRole"=w790) -> (w789:T20)
              }
              frame 2, Default {
                n412 = Unbundle By Name(w798) -> ("MarkerRole"=w799:refnum<class "MarkerRole.lvclass">)
                n413 = property class="Robot"(reference=w794, "role"=roles."Marker") -> (reference out=w793:refnum<class "Robot.lvclass">)  [unwired: 1 in, 1 out]
                n414 = property class="MarkerRole"(reference=w799, "RobotRef"=w793) -> (reference out=w797:refnum<class "MarkerRole.lvclass">)  [unwired: 1 in, 1 out]
                n415 = Bundle By Name(cluster=w798, "MarkerRole"=w797) -> (w796:T20)
              }
            }
            n416 = property class="EnemyPossessionAtOurFieldPlay"(reference=w783, "Roles"=w784) -> (reference out=w782:refnum<class "EnemyPossessionAtOurFieldPlay.lvclass">)  [unwired: 1 in, 1 out]
            n417 = Bundle By Name(cluster=w775, "EnemyPossessionAtOurFieldPlay"=w782) -> (w776:T5)
            n418 = property class="Playbook"(reference=w781, "offensive_plays"=w776) -> (reference out=w780:refnum<class "Playbook.lvclass">)  [unwired: 1 in, 1 out]
          }
        }
        frame "PrepareKickoffAlly" {
          n419 = property class="Playbook"(reference=w812) -> (reference out=w805:refnum<class "Playbook.lvclass">, "offensive_plays"=w811:T5)  [unwired: 1 in, 1 out]
          n420 = Unbundle By Name(w811) -> ("PrepareKickoffAllyPlay"=w808:refnum<class "PrepareKickoffAllyPlay.lvclass">)
          n421 = property class="PrepareKickoffAllyPlay"(reference=w808) -> ("NumberOfRobots"=w807:dbl)  [unwired: 1 in, 2 out]
          n422 = call-dynamic "pickOffensiveTeam.vi"("OffensiveTeam in"=w801, "Game"=w800, "KeeperTeam"=w802, "number_of_robots"=w807, "RobotRef"=w806) -> ("OffensiveTeam out"=w803:refnum<class "Ally.lvclass">, "RobotRef"=w804:refnum<class "Robot.lvclass">[])  [unwired: 8 in, 1 out]
          n423 = for {
            tunnel: [w813] -> w809 mode=indexing
            tunnel: w804 -> [w819] mode=indexing
            shift-right: [w820] -> w810
            shift-left: w805 -> [w821]
            shift-right: [w816] -> _
            shift-left: w811 -> [w815]
            i -> [w818]
            n424 = Unbundle By Name(w815) -> ("PrepareKickoffAllyPlay"=w814:refnum<class "PrepareKickoffAllyPlay.lvclass">)
            n425 = property class="PrepareKickoffAllyPlay"(reference=w814) -> (reference out=w823:refnum<class "PrepareKickoffAllyPlay.lvclass">, "Roles"=w825:T21)  [unwired: 1 in, 1 out]
            n426 = Increment(x=w818) -> (x+1=w817:i32)
            n427 = case shown="1, Default" w817 {
              tunnel: w825 -> [w831 w838]
              tunnel: [w829 w836] -> w824
              tunnel: w819 -> [w828 w834]
              tunnel: [w826 w833] -> w813
              frame 1, Default {
                n428 = Unbundle By Name(w831) -> ("AttackerAimGoalRole"=w832:refnum<class "AttackerAimGoalRole.lvclass">)
                n429 = property class="Robot"(reference=w828, "role"=roles."AttackerAimGoal") -> (reference out=w826:refnum<class "Robot.lvclass">)  [unwired: 1 in, 1 out]
                n430 = property class="AttackerAimGoalRole"(reference=w832, "RobotRef"=w826) -> (reference out=w830:refnum<class "AttackerAimGoalRole.lvclass">)  [unwired: 1 in, 1 out]
                n431 = Bundle By Name(cluster=w831, "AttackerAimGoalRole"=w830) -> (w829:T21)
              }
              frame 2 {
                n432 = Unbundle By Name(w838) -> ("FollowAttackerRole"=w839:refnum<class "FollowAttackerRole.lvclass">)
                n433 = property class="Robot"(reference=w834, "role"=roles."FollowAttacker") -> (reference out=w833:refnum<class "Robot.lvclass">)  [unwired: 1 in, 1 out]
                n434 = property class="FollowAttackerRole"(reference=w839, "RobotRef"=w833) -> (reference out=w837:refnum<class "FollowAttackerRole.lvclass">)  [unwired: 1 in, 1 out]
                n435 = Bundle By Name(cluster=w838, "FollowAttackerRole"=w837) -> (w836:T21)
              }
            }
            n436 = property class="PrepareKickoffAllyPlay"(reference=w823, "Roles"=w824) -> (reference out=w822:refnum<class "PrepareKickoffAllyPlay.lvclass">)  [unwired: 1 in, 1 out]
            n437 = Bundle By Name(cluster=w815, "PrepareKickoffAllyPlay"=w822) -> (w816:T5)
            n438 = property class="Playbook"(reference=w821, "offensive_plays"=w816) -> (reference out=w820:refnum<class "Playbook.lvclass">)  [unwired: 1 in, 1 out]
          }
        }
        frame "PrepareKickoffEnemy" {
          n439 = property class="Playbook"(reference=w852) -> (reference out=w845:refnum<class "Playbook.lvclass">, "offensive_plays"=w851:T5)  [unwired: 1 in, 1 out]
          n440 = Unbundle By Name(w851) -> ("PrepareKickoffEnemyPlay"=w848:refnum<class "PrepareKickoffEnemyPlay.lvclass">)
          n441 = property class="PrepareKickoffEnemyPlay"(reference=w848) -> ("NumberOfRobots"=w847:dbl)  [unwired: 1 in, 2 out]
          n442 = call-dynamic "pickOffensiveTeam.vi"("OffensiveTeam in"=w841, "Game"=w840, "KeeperTeam"=w842, "number_of_robots"=w847, "RobotRef"=w846) -> ("OffensiveTeam out"=w843:refnum<class "Ally.lvclass">, "RobotRef"=w844:refnum<class "Robot.lvclass">[])  [unwired: 8 in, 1 out]
          n443 = for {
            tunnel: [w853] -> w849 mode=indexing
            tunnel: w844 -> [w859] mode=indexing
            shift-right: [w860] -> w850
            shift-left: w845 -> [w861]
            shift-right: [w856] -> _
            shift-left: w851 -> [w855]
            i -> [w858]
            n444 = Unbundle By Name(w855) -> ("PrepareKickoffEnemyPlay"=w854:refnum<class "PrepareKickoffEnemyPlay.lvclass">)
            n445 = property class="PrepareKickoffEnemyPlay"(reference=w854) -> (reference out=w863:refnum<class "PrepareKickoffEnemyPlay.lvclass">, "Roles"=w865:T22)  [unwired: 1 in, 1 out]
            n446 = Increment(x=w858) -> (x+1=w857:i32)
            n447 = case shown="2" w857 {
              tunnel: w865 -> [w871 w878]
              tunnel: [w869 w876] -> w864
              tunnel: w859 -> [w868 w874]
              tunnel: [w866 w873] -> w853
              frame 1, Default {
                n448 = Unbundle By Name(w871) -> ("AttackerBlockRole"=w872:refnum<class "AttackerBlockRole.lvclass">)
                n449 = property class="Robot"(reference=w868, "role"=roles."AttackerBlock") -> (reference out=w866:refnum<class "Robot.lvclass">)  [unwired: 1 in, 1 out]
                n450 = property class="AttackerBlockRole"(reference=w872, "RobotRef"=w866) -> (reference out=w870:refnum<class "AttackerBlockRole.lvclass">)  [unwired: 1 in, 1 out]
                n451 = Bundle By Name(cluster=w871, "AttackerBlockRole"=w870) -> (w869:T22)
              }
              frame 2 {
                n452 = Unbundle By Name(w878) -> ("FollowAttackerRole"=w879:refnum<class "FollowAttackerRole.lvclass">)
                n453 = property class="Robot"(reference=w874, "role"=roles."FollowAttacker") -> (reference out=w873:refnum<class "Robot.lvclass">)  [unwired: 1 in, 1 out]
                n454 = property class="FollowAttackerRole"(reference=w879, "RobotRef"=w873) -> (reference out=w877:refnum<class "FollowAttackerRole.lvclass">)  [unwired: 1 in, 1 out]
                n455 = Bundle By Name(cluster=w878, "FollowAttackerRole"=w877) -> (w876:T22)
              }
            }
            n456 = property class="PrepareKickoffEnemyPlay"(reference=w863, "Roles"=w864) -> (reference out=w862:refnum<class "PrepareKickoffEnemyPlay.lvclass">)  [unwired: 1 in, 1 out]
            n457 = Bundle By Name(cluster=w855, "PrepareKickoffEnemyPlay"=w862) -> (w856:T5)
            n458 = property class="Playbook"(reference=w861, "offensive_plays"=w856) -> (reference out=w860:refnum<class "Playbook.lvclass">)  [unwired: 1 in, 1 out]
          }
        }
        frame "PreparePass" {
          n459 = property class="Playbook"(reference=w887) -> (reference out=w883:refnum<class "Playbook.lvclass">, "offensive_plays"=w892:T5)  [unwired: 1 in, 1 out]
          n460 = Unbundle By Name(w892) -> ("PreparePassPlay"=w891:refnum<class "PreparePassPlay.lvclass">)
          n461 = property class="PreparePassPlay"(reference=w891) -> ("NumberOfRobots"=w890:dbl)  [unwired: 1 in, 2 out]
          n462 = call-dynamic "pickOffensiveTeam.vi"("OffensiveTeam in"=w885, "Game"=w884, "KeeperTeam"=w888, "number_of_robots"=w890, "RobotRef"=w886) -> ("OffensiveTeam out"=w882:refnum<class "Ally.lvclass">, "RobotRef"=w889:refnum<class "Robot.lvclass">[])  [unwired: 8 in, 1 out]
          n463 = for {
            tunnel: [w893] -> w880 mode=indexing
            tunnel: w889 -> [w899] mode=indexing
            shift-right: [w900] -> w881
            shift-left: w883 -> [w901]
            shift-right: [w896] -> _
            shift-left: w892 -> [w895]
            i -> [w898]
            n464 = Unbundle By Name(w895) -> ("PreparePassPlay"=w894:refnum<class "PreparePassPlay.lvclass">)
            n465 = property class="PreparePassPlay"(reference=w894) -> (reference out=w903:refnum<class "PreparePassPlay.lvclass">, "Roles"=w905:T23)  [unwired: 1 in, 1 out]
            n466 = Increment(x=w898) -> (x+1=w897:i32)
            n467 = case shown="3" w897 {
              tunnel: w905 -> [w911 w918 w922]
              tunnel: [w909 w916 w921] -> w904
              tunnel: w899 -> [w908 w914 w923]
              tunnel: [w907 w913 w920] -> w893
              frame 1, Default {
                n468 = Unbundle By Name(w911) -> ("AttackerStopRole"=w912:refnum<class "AttackerStopRole.lvclass">)
                n469 = property class="Robot"(reference=w908, "role"=roles."AttackerStop") -> (reference out=w907:refnum<class "Robot.lvclass">)  [unwired: 1 in, 1 out]
                n470 = property class="AttackerStopRole"(reference=w912, "RobotRef"=w907) -> (reference out=w910:refnum<class "AttackerStopRole.lvclass">)  [unwired: 1 in, 1 out]
                n471 = Bundle By Name(cluster=w911, "AttackerStopRole"=w910) -> (w909:T23)
              }
              frame 2 {
                n472 = Unbundle By Name(w918) -> ("PreparePassReceiverRole 1"=w919:refnum<class "PreparePassReceiverRole.lvclass">)
                n473 = property class="Robot"(reference=w914, "role"=roles."PreparePassReceiver 1") -> (reference out=w913:refnum<class "Robot.lvclass">)  [unwired: 1 in, 1 out]
                n474 = property class="PreparePassReceiverRole"(reference=w919, "RobotRef"=w913) -> (reference out=w917:refnum<class "PreparePassReceiverRole.lvclass">)  [unwired: 1 in, 1 out]
                n475 = Bundle By Name(cluster=w918, "PreparePassReceiverRole 1"=w917) -> (w916:T23)
              }
              frame 3 {
                n476 = Unbundle By Name(w922) -> ("PreparePassReceiverRole 2"=w926:refnum<class "PreparePassReceiverRole.lvclass">)
                n477 = property class="Robot"(reference=w923, "role"=roles."PreparePassReceiver 2") -> (reference out=w920:refnum<class "Robot.lvclass">)  [unwired: 1 in, 1 out]
                n478 = property class="PreparePassReceiverRole"(reference=w926, "RobotRef"=w920) -> (reference out=w925:refnum<class "PreparePassReceiverRole.lvclass">)  [unwired: 1 in, 1 out]
                n479 = Bundle By Name(cluster=w922, "PreparePassReceiverRole 2"=w925) -> (w921:T23)
              }
            }
            n480 = property class="PreparePassPlay"(reference=w903, "Roles"=w904) -> (reference out=w902:refnum<class "PreparePassPlay.lvclass">)  [unwired: 1 in, 1 out]
            n481 = Bundle By Name(cluster=w895, "PreparePassPlay"=w902) -> (w896:T5)
            n482 = property class="Playbook"(reference=w901, "offensive_plays"=w896) -> (reference out=w900:refnum<class "Playbook.lvclass">)  [unwired: 1 in, 1 out]
          }
        }
        frame "PrepareDoublePass" {
          n483 = property class="Playbook"(reference=w934) -> (reference out=w930:refnum<class "Playbook.lvclass">, "offensive_plays"=w939:T5)  [unwired: 1 in, 1 out]
          n484 = Unbundle By Name(w939) -> ("PrepareDoublePassPlay"=w938:refnum<class "PrepareDoublePassPlay.lvclass">)
          n485 = property class="PrepareDoublePassPlay"(reference=w938) -> ("NumberOfRobots"=w937:dbl)  [unwired: 1 in, 2 out]
          n486 = call-dynamic "pickOffensiveTeam.vi"("OffensiveTeam in"=w932, "Game"=w931, "KeeperTeam"=w935, "number_of_robots"=w937, "RobotRef"=w933) -> ("OffensiveTeam out"=w929:refnum<class "Ally.lvclass">, "RobotRef"=w936:refnum<class "Robot.lvclass">[])  [unwired: 8 in, 1 out]
          n487 = for {
            tunnel: [w940] -> w927 mode=indexing
            tunnel: w936 -> [w946] mode=indexing
            shift-right: [w947] -> w928
            shift-left: w930 -> [w948]
            shift-right: [w943] -> _
            shift-left: w939 -> [w942]
            i -> [w945]
            n488 = Unbundle By Name(w942) -> ("PrepareDoublePassPlay"=w941:refnum<class "PrepareDoublePassPlay.lvclass">)
            n489 = property class="PrepareDoublePassPlay"(reference=w941) -> (reference out=w950:refnum<class "PrepareDoublePassPlay.lvclass">, "Roles"=w952:T24)  [unwired: 1 in, 1 out]
            n490 = Increment(x=w945) -> (x+1=w944:i32)
            n491 = case shown="3" w944 {
              tunnel: w952 -> [w958 w962 w972]
              tunnel: [w956 w961 w970] -> w951
              tunnel: w946 -> [w955 w963 w968]
              tunnel: [w954 w960 w967] -> w940
              frame 1, Default {
                n492 = Unbundle By Name(w958) -> ("AttackerStopRole"=w959:refnum<class "AttackerStopRole.lvclass">)
                n493 = property class="Robot"(reference=w955, "role"=roles."AttackerStop") -> (reference out=w954:refnum<class "Robot.lvclass">)  [unwired: 1 in, 1 out]
                n494 = property class="AttackerStopRole"(reference=w959, "RobotRef"=w954) -> (reference out=w957:refnum<class "AttackerStopRole.lvclass">)  [unwired: 1 in, 1 out]
                n495 = Bundle By Name(cluster=w958, "AttackerStopRole"=w957) -> (w956:T24)
              }
              frame 2 {
                n496 = Unbundle By Name(w962) -> ("PreparePassReceiverRole 1"=w966:refnum<class "PreparePassReceiverRole.lvclass">)
                n497 = property class="Robot"(reference=w963, "role"=roles."PreparePassReceiver 1") -> (reference out=w960:refnum<class "Robot.lvclass">)  [unwired: 1 in, 1 out]
                n498 = property class="PreparePassReceiverRole"(reference=w966, "RobotRef"=w960) -> (reference out=w965:refnum<class "PreparePassReceiverRole.lvclass">)  [unwired: 1 in, 1 out]
                n499 = Bundle By Name(cluster=w962, "PreparePassReceiverRole 1"=w965) -> (w961:T24)
              }
              frame 3 {
                n500 = Unbundle By Name(w972) -> ("PreparePassReceiverRole 2"=w973:refnum<class "PreparePassReceiverRole.lvclass">)
                n501 = property class="Robot"(reference=w968, "role"=roles."PreparePassReceiver 2") -> (reference out=w967:refnum<class "Robot.lvclass">)  [unwired: 1 in, 1 out]
                n502 = property class="PreparePassReceiverRole"(reference=w973, "RobotRef"=w967) -> (reference out=w971:refnum<class "PreparePassReceiverRole.lvclass">)  [unwired: 1 in, 1 out]
                n503 = Bundle By Name(cluster=w972, "PreparePassReceiverRole 2"=w971) -> (w970:T24)
              }
            }
            n504 = property class="PrepareDoublePassPlay"(reference=w950, "Roles"=w951) -> (reference out=w949:refnum<class "PrepareDoublePassPlay.lvclass">)  [unwired: 1 in, 1 out]
            n505 = Bundle By Name(cluster=w942, "PrepareDoublePassPlay"=w949) -> (w943:T5)
            n506 = property class="Playbook"(reference=w948, "offensive_plays"=w943) -> (reference out=w947:refnum<class "Playbook.lvclass">)  [unwired: 1 in, 1 out]
          }
        }
        frame "PrepareTriplePass" {
          n507 = property class="Playbook"(reference=w981) -> (reference out=w977:refnum<class "Playbook.lvclass">, "offensive_plays"=w986:T5)  [unwired: 1 in, 1 out]
          n508 = Unbundle By Name(w986) -> ("PrepareDoublePassPlay"=w985:refnum<class "PrepareDoublePassPlay.lvclass">)
          n509 = property class="PrepareDoublePassPlay"(reference=w985) -> ("NumberOfRobots"=w984:dbl)  [unwired: 1 in, 2 out]
          n510 = call-dynamic "pickOffensiveTeam.vi"("OffensiveTeam in"=w979, "Game"=w978, "KeeperTeam"=w982, "number_of_robots"=w984, "RobotRef"=w980) -> ("OffensiveTeam out"=w976:refnum<class "Ally.lvclass">, "RobotRef"=w983:refnum<class "Robot.lvclass">[])  [unwired: 8 in, 1 out]
          n511 = for {
            tunnel: [w987] -> w974 mode=indexing
            tunnel: w983 -> [w993] mode=indexing
            shift-right: [w994] -> w975
            shift-left: w977 -> [w995]
            shift-right: [w990] -> _
            shift-left: w986 -> [w989]
            i -> [w992]
            n512 = Unbundle By Name(w989) -> ("PrepareTriplePassPlay"=w988:refnum<class "PrepareTriplePassPlay.lvclass">)
            n513 = property class="PrepareTriplePassPlay"(reference=w988) -> (reference out=w997:refnum<class "PrepareTriplePassPlay.lvclass">, "Roles"=w999:T25)  [unwired: 1 in, 1 out]
            n514 = Increment(x=w992) -> (x+1=w991:i32)
            n515 = case shown="2" w991 {
              tunnel: w999 -> [w1005 w1009 w1019]
              tunnel: [w1003 w1008 w1017] -> w998
              tunnel: w993 -> [w1002 w1010 w1015]
              tunnel: [w1001 w1007 w1014] -> w987
              frame 1, Default {
                n516 = Unbundle By Name(w1005) -> ("AttackerStopRole"=w1006:refnum<class "AttackerStopRole.lvclass">)
                n517 = property class="Robot"(reference=w1002, "role"=roles."AttackerStop") -> (reference out=w1001:refnum<class "Robot.lvclass">)  [unwired: 1 in, 1 out]
                n518 = property class="AttackerStopRole"(reference=w1006, "RobotRef"=w1001) -> (reference out=w1004:refnum<class "AttackerStopRole.lvclass">)  [unwired: 1 in, 1 out]
                n519 = Bundle By Name(cluster=w1005, "AttackerStopRole"=w1004) -> (w1003:T25)
              }
              frame 2 {
                n520 = Unbundle By Name(w1009) -> ("PreparePassReceiverRole 1"=w1013:refnum<class "PreparePassReceiverRole.lvclass">)
                n521 = property class="Robot"(reference=w1010, "role"=roles."PreparePassReceiver 1") -> (reference out=w1007:refnum<class "Robot.lvclass">)  [unwired: 1 in, 1 out]
                n522 = property class="PreparePassReceiverRole"(reference=w1013, "RobotRef"=w1007) -> (reference out=w1012:refnum<class "PreparePassReceiverRole.lvclass">)  [unwired: 1 in, 1 out]
                n523 = Bundle By Name(cluster=w1009, "PreparePassReceiverRole 1"=w1012) -> (w1008:T25)
              }
              frame 3 {
                n524 = Unbundle By Name(w1019) -> ("PreparePassReceiverRole 2"=w1020:refnum<class "PreparePassReceiverRole.lvclass">)
                n525 = property class="Robot"(reference=w1015, "role"=roles."PreparePassReceiver 2") -> (reference out=w1014:refnum<class "Robot.lvclass">)  [unwired: 1 in, 1 out]
                n526 = property class="PreparePassReceiverRole"(reference=w1020, "RobotRef"=w1014) -> (reference out=w1018:refnum<class "PreparePassReceiverRole.lvclass">)  [unwired: 1 in, 1 out]
                n527 = Bundle By Name(cluster=w1019, "PreparePassReceiverRole 2"=w1018) -> (w1017:T25)
              }
            }
            n528 = property class="PrepareTriplePassPlay"(reference=w997, "Roles"=w998) -> (reference out=w996:refnum<class "PrepareTriplePassPlay.lvclass">)  [unwired: 1 in, 1 out]
            n529 = Bundle By Name(cluster=w989, "PrepareTriplePassPlay"=w996) -> (w990:T5)
            n530 = property class="Playbook"(reference=w995, "offensive_plays"=w990) -> (reference out=w994:refnum<class "Playbook.lvclass">)  [unwired: 1 in, 1 out]
          }
        }
        frame "ABCPass" {
          n531 = property class="Playbook"(reference=w1028) -> (reference out=w1024:refnum<class "Playbook.lvclass">, "offensive_plays"=w1033:T5)  [unwired: 1 in, 1 out]
          n532 = Unbundle By Name(w1033) -> ("ABCPassPlay"=w1032:refnum<class "ABCPassPlay.lvclass">)
          n533 = property class="ABCPassPlay"(reference=w1032) -> ("NumberOfRobots"=w1031:dbl)  [unwired: 1 in, 2 out]
          n534 = call-dynamic "pickOffensiveTeam.vi"("OffensiveTeam in"=w1026, "Game"=w1025, "KeeperTeam"=w1029, "number_of_robots"=w1031, "RobotRef"=w1027) -> ("OffensiveTeam out"=w1023:refnum<class "Ally.lvclass">, "RobotRef"=w1030:refnum<class "Robot.lvclass">[])  [unwired: 8 in, 1 out]
          n535 = for {
            tunnel: [w1034] -> w1021 mode=indexing
            tunnel: w1030 -> [w1040] mode=indexing
            shift-right: [w1041] -> w1022
            shift-left: w1024 -> [w1042]
            shift-right: [w1037] -> _
            shift-left: w1033 -> [w1036]
            i -> [w1039]
            n536 = Unbundle By Name(w1036) -> ("ABCPassPlay"=w1035:refnum<class "ABCPassPlay.lvclass">)
            n537 = property class="ABCPassPlay"(reference=w1035) -> (reference out=w1044:refnum<class "ABCPassPlay.lvclass">, "Roles"=w1046:T26)  [unwired: 1 in, 1 out]
            n538 = Increment(x=w1039) -> (x+1=w1038:i32)
            n539 = case shown="3" w1038 {
              tunnel: w1046 -> [w1052 w1056 w1066]
              tunnel: [w1050 w1055 w1064] -> w1045
              tunnel: w1040 -> [w1049 w1057 w1062]
              tunnel: [w1048 w1054 w1061] -> w1034
              frame 1, Default {
                n540 = Unbundle By Name(w1052) -> ("ABCFirstKickerRole"=w1053:refnum<class "ABCFirstKickerRole.lvclass">)
                n541 = property class="Robot"(reference=w1049, "role"=roles."ABCFirstKicker") -> (reference out=w1048:refnum<class "Robot.lvclass">)  [unwired: 1 in, 1 out]
                n542 = property class="ABCFirstKickerRole"(reference=w1053, "RobotRef"=w1048) -> (reference out=w1051:refnum<class "ABCFirstKickerRole.lvclass">)  [unwired: 1 in, 1 out]
                n543 = Bundle By Name(cluster=w1052, "ABCFirstKickerRole"=w1051) -> (w1050:T26)
              }
              frame 2 {
                n544 = Unbundle By Name(w1056) -> ("ABCSecondKicker"=w1060:refnum<class "ABCSecondKicker.lvclass">)
                n545 = property class="Robot"(reference=w1057, "role"=roles."ABCSecondKicker") -> (reference out=w1054:refnum<class "Robot.lvclass">)  [unwired: 1 in, 1 out]
                n546 = property class="ABCSecondKicker"(reference=w1060, "RobotRef"=w1054) -> (reference out=w1059:refnum<class "ABCSecondKicker.lvclass">)  [unwired: 1 in, 1 out]
                n547 = Bundle By Name(cluster=w1056, "ABCSecondKicker"=w1059) -> (w1055:T26)
              }
              frame 3 {
                n548 = Unbundle By Name(w1066) -> ("ABCThirdKicker"=w1067:refnum<class "ABCThirdKicker.lvclass">)
                n549 = property class="Robot"(reference=w1062, "role"=roles."ABCThirdKicker") -> (reference out=w1061:refnum<class "Robot.lvclass">)  [unwired: 1 in, 1 out]
                n550 = property class="ABCThirdKicker"(reference=w1067, "RobotRef"=w1061) -> (reference out=w1065:refnum<class "ABCThirdKicker.lvclass">)  [unwired: 1 in, 1 out]
                n551 = Bundle By Name(cluster=w1066, "ABCThirdKicker"=w1065) -> (w1064:T26)
              }
            }
            n552 = property class="ABCPassPlay"(reference=w1044, "Roles"=w1045) -> (reference out=w1043:refnum<class "ABCPassPlay.lvclass">)  [unwired: 1 in, 1 out]
            n553 = Bundle By Name(cluster=w1036, "ABCPassPlay"=w1043) -> (w1037:T5)
            n554 = property class="Playbook"(reference=w1042, "offensive_plays"=w1037) -> (reference out=w1041:refnum<class "Playbook.lvclass">)  [unwired: 1 in, 1 out]
          }
        }
        frame "ACBPass" {
          n555 = property class="Playbook"(reference=w1075) -> (reference out=w1071:refnum<class "Playbook.lvclass">, "offensive_plays"=w1080:T5)  [unwired: 1 in, 1 out]
          n556 = Unbundle By Name(w1080) -> ("ACBPassPlay"=w1079:refnum<class "ACBPassPlay.lvclass">)
          n557 = property class="ACBPassPlay"(reference=w1079) -> ("NumberOfRobots"=w1078:dbl)  [unwired: 1 in, 2 out]
          n558 = call-dynamic "pickOffensiveTeam.vi"("OffensiveTeam in"=w1073, "Game"=w1072, "KeeperTeam"=w1076, "number_of_robots"=w1078, "RobotRef"=w1074) -> ("OffensiveTeam out"=w1070:refnum<class "Ally.lvclass">, "RobotRef"=w1077:refnum<class "Robot.lvclass">[])  [unwired: 8 in, 1 out]
          n559 = for {
            tunnel: [w1081] -> w1068 mode=indexing
            tunnel: w1077 -> [w1087] mode=indexing
            shift-right: [w1088] -> w1069
            shift-left: w1071 -> [w1089]
            shift-right: [w1084] -> _
            shift-left: w1080 -> [w1083]
            i -> [w1086]
            n560 = Unbundle By Name(w1083) -> ("ACBPassPlay"=w1082:refnum<class "ACBPassPlay.lvclass">)
            n561 = property class="ACBPassPlay"(reference=w1082) -> (reference out=w1091:refnum<class "ACBPassPlay.lvclass">, "Roles"=w1093:T26)  [unwired: 1 in, 1 out]
            n562 = Increment(x=w1086) -> (x+1=w1085:i32)
            n563 = case shown="2" w1085 {
              tunnel: w1093 -> [w1099 w1103 w1113]
              tunnel: [w1097 w1102 w1111] -> w1092
              tunnel: w1087 -> [w1096 w1104 w1109]
              tunnel: [w1095 w1101 w1108] -> w1081
              frame 1, Default {
                n564 = Unbundle By Name(w1099) -> ("ABCFirstKickerRole"=w1100:refnum<class "ABCFirstKickerRole.lvclass">)
                n565 = property class="Robot"(reference=w1096, "role"=roles."ABCFirstKicker") -> (reference out=w1095:refnum<class "Robot.lvclass">)  [unwired: 1 in, 1 out]
                n566 = property class="ABCFirstKickerRole"(reference=w1100, "RobotRef"=w1095) -> (reference out=w1098:refnum<class "ABCFirstKickerRole.lvclass">)  [unwired: 1 in, 1 out]
                n567 = Bundle By Name(cluster=w1099, "ABCFirstKickerRole"=w1098) -> (w1097:T26)
              }
              frame 2 {
                n568 = Unbundle By Name(w1103) -> ("ABCThirdKicker"=w1107:refnum<class "ABCThirdKicker.lvclass">)
                n569 = property class="Robot"(reference=w1104, "role"=roles."ABCThirdKicker") -> (reference out=w1101:refnum<class "Robot.lvclass">)  [unwired: 1 in, 1 out]
                n570 = property class="ABCThirdKicker"(reference=w1107, "RobotRef"=w1101) -> (reference out=w1106:refnum<class "ABCThirdKicker.lvclass">)  [unwired: 1 in, 1 out]
                n571 = Bundle By Name(cluster=w1103, "ABCThirdKicker"=w1106) -> (w1102:T26)
              }
              frame 3 {
                n572 = Unbundle By Name(w1113) -> ("ABCSecondKicker"=w1114:refnum<class "ABCSecondKicker.lvclass">)
                n573 = property class="Robot"(reference=w1109, "role"=roles."ABCSecondKicker") -> (reference out=w1108:refnum<class "Robot.lvclass">)  [unwired: 1 in, 1 out]
                n574 = property class="ABCSecondKicker"(reference=w1114, "RobotRef"=w1108) -> (reference out=w1112:refnum<class "ABCSecondKicker.lvclass">)  [unwired: 1 in, 1 out]
                n575 = Bundle By Name(cluster=w1113, "ABCSecondKicker"=w1112) -> (w1111:T26)
              }
            }
            n576 = property class="ACBPassPlay"(reference=w1091, "Roles"=w1092) -> (reference out=w1090:refnum<class "ACBPassPlay.lvclass">)  [unwired: 1 in, 1 out]
            n577 = Bundle By Name(cluster=w1083, "ACBPassPlay"=w1090) -> (w1084:T5)
            n578 = property class="Playbook"(reference=w1089, "offensive_plays"=w1084) -> (reference out=w1088:refnum<class "Playbook.lvclass">)  [unwired: 1 in, 1 out]
          }
        }
        frame "PrepareRollToPass" {
          n579 = property class="Playbook"(reference=w1123) -> (reference out=w1119:refnum<class "Playbook.lvclass">, "offensive_plays"=w1127:T5)  [unwired: 1 in, 1 out]
          n580 = Unbundle By Name(w1127) -> ("PrepareRollToPassPlay"=w1126:refnum<class "PrepareRollToPassPlay.lvclass">)
          n581 = property class="PrepareRollToPassPlay"(reference=w1126) -> ("NumberOfRobots"=w1115:dbl)  [unwired: 1 in, 2 out]
          n582 = call-dynamic "pickOffensiveTeam.vi"("OffensiveTeam in"=w1121, "Game"=w1120, "KeeperTeam"=w1124, "number_of_robots"=w1115, "RobotRef"=w1122) -> ("OffensiveTeam out"=w1118:refnum<class "Ally.lvclass">, "RobotRef"=w1125:refnum<class "Robot.lvclass">[])  [unwired: 8 in, 1 out]
          n583 = for {
            tunnel: [w1129] -> w1116 mode=indexing
            tunnel: w1125 -> [w1135] mode=indexing
            shift-right: [w1136] -> w1117
            shift-left: w1119 -> [w1137]
            shift-right: [w1132] -> _
            shift-left: w1127 -> [w1131]
            i -> [w1134]
            n584 = Unbundle By Name(w1131) -> ("PrepareRollToPassPlay"=w1130:refnum<class "PrepareRollToPassPlay.lvclass">)
            n585 = Increment(x=w1134) -> (x+1=w1133:i32)
            n586 = property class="PrepareRollToPassPlay"(reference=w1130) -> (reference out=w1139:refnum<class "PrepareRollToPassPlay.lvclass">, "Roles"=w1128:T27)  [unwired: 1 in, 1 out]
            n587 = case shown="4" w1133 {
              tunnel: w1128 -> [w1146 w1153 w1157 w1164]
              tunnel: [w1144 w1151 w1156 w1163] -> w1140
              tunnel: w1135 -> [w1143 w1149 w1158 w1165]
              tunnel: [w1141 w1148 w1155 w1162] -> w1129
              frame 1, Default {
                n588 = Unbundle By Name(w1146) -> ("PrepareRollToPassReceiverRole"=w1147:refnum<class "PrepareRollToPassReceiverRole.lvclass">)
                n589 = property class="Robot"(reference=w1143, "role"=roles."PrepareRollToPassReceiver") -> (reference out=w1141:refnum<class "Robot.lvclass">)  [unwired: 1 in, 1 out]
                n590 = property class="PrepareRollToPassReceiverRole"(reference=w1147, "RobotRef"=w1141) -> (reference out=w1145:refnum<class "PrepareRollToPassReceiverRole.lvclass">)  [unwired: 1 in, 1 out]
                n591 = Bundle By Name(cluster=w1146, "PrepareRollToPassReceiverRole"=w1145) -> (w1144:T27)
              }
              frame 2 {
                n592 = Unbundle By Name(w1153) -> ("PreparePassReceiverRole 1"=w1154:refnum<class "PreparePassReceiverRole.lvclass">)
                n593 = property class="Robot"(reference=w1149, "role"=roles."PreparePassReceiver 1") -> (reference out=w1148:refnum<class "Robot.lvclass">)  [unwired: 1 in, 1 out]
                n594 = property class="PreparePassReceiverRole"(reference=w1154, "RobotRef"=w1148) -> (reference out=w1152:refnum<class "PreparePassReceiverRole.lvclass">)  [unwired: 1 in, 1 out]
                n595 = Bundle By Name(cluster=w1153, "PreparePassReceiverRole 1"=w1152) -> (w1151:T27)
              }
              frame 3 {
                n596 = Unbundle By Name(w1157) -> ("PrepareRollToPassRollerRole"=w1161:refnum<class "PrepareRollToPassRollerRole.lvclass">)
                n597 = property class="Robot"(reference=w1158, "role"=roles."PrepareRollToPassRoller") -> (reference out=w1155:refnum<class "Robot.lvclass">)  [unwired: 1 in, 1 out]
                n598 = property class="PrepareRollToPassRollerRole"(reference=w1161, "RobotRef"=w1155) -> (reference out=w1160:refnum<class "PrepareRollToPassRollerRole.lvclass">)  [unwired: 1 in, 1 out]
                n599 = Bundle By Name(cluster=w1157, "PrepareRollToPassRollerRole"=w1160) -> (w1156:T27)
              }
              frame 4 {
                n600 = Unbundle By Name(w1164) -> ("PreparePassReceiverRole 2"=w1168:refnum<class "PreparePassReceiverRole.lvclass">)
                n601 = property class="Robot"(reference=w1165, "role"=roles."PreparePassReceiver 2") -> (reference out=w1162:refnum<class "Robot.lvclass">)  [unwired: 1 in, 1 out]
                n602 = property class="PreparePassReceiverRole"(reference=w1168, "RobotRef"=w1162) -> (reference out=w1167:refnum<class "PreparePassReceiverRole.lvclass">)  [unwired: 1 in, 1 out]
                n603 = Bundle By Name(cluster=w1164, "PreparePassReceiverRole 2"=w1167) -> (w1163:T27)
              }
            }
            n604 = property class="PrepareRollToPassPlay"(reference=w1139, "Roles"=w1140) -> (reference out=w1138:refnum<class "PrepareRollToPassPlay.lvclass">)  [unwired: 1 in, 1 out]
            n605 = Bundle By Name(cluster=w1131, "PrepareRollToPassPlay"=w1138) -> (w1132:T5)
            n606 = property class="Playbook"(reference=w1137, "offensive_plays"=w1132) -> (reference out=w1136:refnum<class "Playbook.lvclass">)  [unwired: 1 in, 1 out]
          }
        }
        frame "SimplePass" {
          n607 = property class="Playbook"(reference=w1176) -> (reference out=w1172:refnum<class "Playbook.lvclass">, "offensive_plays"=w1181:T5)  [unwired: 1 in, 1 out]
          n608 = Unbundle By Name(w1181) -> ("SimplePassPlay"=w1180:refnum<class "SimplePass.lvclass">)
          n609 = property class="SimplePass"(reference=w1180) -> ("NumberOfRobots"=w1179:dbl)  [unwired: 1 in, 2 out]
          n610 = call-dynamic "pickOffensiveTeam.vi"("OffensiveTeam in"=w1174, "Game"=w1173, "KeeperTeam"=w1177, "number_of_robots"=w1179, "RobotRef"=w1175) -> ("OffensiveTeam out"=w1171:refnum<class "Ally.lvclass">, "RobotRef"=w1178:refnum<class "Robot.lvclass">[])  [unwired: 8 in, 1 out]
          n611 = for {
            tunnel: [w1182] -> w1169 mode=indexing
            tunnel: w1178 -> [w1188] mode=indexing
            shift-right: [w1189] -> w1170
            shift-left: w1172 -> [w1190]
            shift-right: [w1185] -> _
            shift-left: w1181 -> [w1184]
            i -> [w1187]
            n612 = Unbundle By Name(w1184) -> ("SimplePassPlay"=w1183:refnum<class "SimplePass.lvclass">)
            n613 = property class="SimplePass"(reference=w1183) -> (reference out=w1192:refnum<class "SimplePass.lvclass">, "Roles"=w1194:T28)  [unwired: 1 in, 1 out]
            n614 = Increment(x=w1187) -> (x+1=w1186:i32)
            n615 = case shown="2" w1186 {
              tunnel: w1194 -> [w1197 w1207]
              tunnel: [w1196 w1205] -> w1193
              tunnel: w1188 -> [w1198 w1204]
              tunnel: [w1195 w1202] -> w1182
              frame 1, Default {
                n616 = Unbundle By Name(w1197) -> ("SimplePassReceiverRole"=w1201:refnum<class "SimplePassReceiverRole.lvclass">)
                n617 = property class="Robot"(reference=w1198, "role"=roles."SimplePassRollReceiver") -> (reference out=w1195:refnum<class "Robot.lvclass">)  [unwired: 1 in, 1 out]
                n618 = property class="SimplePassReceiverRole"(reference=w1201, "RobotRef"=w1195) -> (reference out=w1200:refnum<class "SimplePassReceiverRole.lvclass">)  [unwired: 1 in, 1 out]
                n619 = Bundle By Name(cluster=w1197, "SimplePassReceiverRole"=w1200) -> (w1196:T28)
              }
              frame 2 {
                n620 = Unbundle By Name(w1207) -> ("SimplePassRollRole"=w1208:refnum<class "SimplePassRollRole.lvclass">)
                n621 = property class="Robot"(reference=w1204, "role"=roles."SimplePassRoll") -> (reference out=w1202:refnum<class "Robot.lvclass">)  [unwired: 1 in, 1 out]
                n622 = property class="SimplePassRollRole"(reference=w1208, "RobotRef"=w1202) -> (reference out=w1206:refnum<class "SimplePassRollRole.lvclass">)  [unwired: 1 in, 1 out]
                n623 = Bundle By Name(cluster=w1207, "SimplePassRollRole"=w1206) -> (w1205:T28)
              }
            }
            n624 = property class="SimplePass"(reference=w1192, "Roles"=w1193) -> (reference out=w1191:refnum<class "SimplePass.lvclass">)  [unwired: 1 in, 1 out]
            n625 = Bundle By Name(cluster=w1184, "SimplePassPlay"=w1191) -> (w1185:T5)
            n626 = property class="Playbook"(reference=w1190, "offensive_plays"=w1185) -> (reference out=w1189:refnum<class "Playbook.lvclass">)  [unwired: 1 in, 1 out]
          }
        }
        frame "PassToStriker" {
          n627 = property class="Playbook"(reference=w1212) -> (reference out=w1218:refnum<class "Playbook.lvclass">, "offensive_plays"=w1221:T5)  [unwired: 1 in, 1 out]
          n628 = Unbundle By Name(w1221) -> ("PassToStrikerPlay"=w1220:refnum<class "PassToStriker.lvclass">)
          n629 = property class="PassToStriker"(reference=w1220) -> ("NumberOfRobots"=w1219:dbl)  [unwired: 1 in, 2 out]
          n630 = call-dynamic "pickOffensiveTeam.vi"("OffensiveTeam in"=w1210, "Game"=w1209, "KeeperTeam"=w1211, "number_of_robots"=w1219, "RobotRef"=w1213) -> ("OffensiveTeam out"=w1216:refnum<class "Ally.lvclass">, "RobotRef"=w1217:refnum<class "Robot.lvclass">[])  [unwired: 8 in, 1 out]
          n631 = for {
            tunnel: [w1222] -> w1214 mode=indexing
            tunnel: w1217 -> [w1228] mode=indexing
            shift-right: [w1229] -> w1215
            shift-left: w1218 -> [w1230]
            shift-right: [w1225] -> _
            shift-left: w1221 -> [w1224]
            i -> [w1227]
            n632 = Unbundle By Name(w1224) -> ("PassToStrikerPlay"=w1223:refnum<class "PassToStriker.lvclass">)
            n633 = property class="PassToStriker"(reference=w1223) -> (reference out=w1232:refnum<class "PassToStriker.lvclass">, "Roles"=w1234:T29)  [unwired: 1 in, 1 out]
            n634 = Increment(x=w1227) -> (x+1=w1226:i32)
            n635 = case shown="2" w1226 {
              tunnel: w1234 -> [w1240 w1247 w1251]
              tunnel: [w1238 w1245 w1250] -> w1233
              tunnel: w1228 -> [w1237 w1243 w1252]
              tunnel: [w1235 w1242 w1249] -> w1222
              frame 1, Default {
                n636 = Unbundle By Name(w1240) -> ("PassKickerRole"=w1241:refnum<class "PassKickerRole.lvclass">)
                n637 = property class="Robot"(reference=w1237, "role"=roles."PassKicker") -> (reference out=w1235:refnum<class "Robot.lvclass">)  [unwired: 1 in, 1 out]
                n638 = property class="PassKickerRole"(reference=w1241, "RobotRef"=w1235) -> (reference out=w1239:refnum<class "PassKickerRole.lvclass">)  [unwired: 1 in, 1 out]
                n639 = Bundle By Name(cluster=w1240, "PassKickerRole"=w1239) -> (w1238:T29)
              }
              frame 2 {
                n640 = Unbundle By Name(w1247) -> ("PassReceiverRole"=w1248:refnum<class "PassReceiverRole.lvclass">)
                n641 = property class="Robot"(reference=w1243, "role"=roles."PassReceiver") -> (reference out=w1242:refnum<class "Robot.lvclass">)  [unwired: 1 in, 1 out]
                n642 = property class="PassReceiverRole"(reference=w1248, "RobotRef"=w1242) -> (reference out=w1246:refnum<class "PassReceiverRole.lvclass">)  [unwired: 1 in, 1 out]
                n643 = Bundle By Name(cluster=w1247, "PassReceiverRole"=w1246) -> (w1245:T29)
              }
              frame 3 {
                n644 = Unbundle By Name(w1251) -> ("PassObserverRole"=w1255:refnum<class "PassObserverRole.lvclass">)
                n645 = property class="Robot"(reference=w1252, "role"=roles."PassObserver") -> (reference out=w1249:refnum<class "Robot.lvclass">)  [unwired: 1 in, 1 out]
                n646 = property class="PassObserverRole"(reference=w1255, "RobotRef"=w1249) -> (reference out=w1254:refnum<class "PassObserverRole.lvclass">)  [unwired: 1 in, 1 out]
                n647 = Bundle By Name(cluster=w1251, "PassObserverRole"=w1254) -> (w1250:T29)
              }
            }
            n648 = property class="PassToStriker"(reference=w1232, "Roles"=w1233) -> (reference out=w1231:refnum<class "PassToStriker.lvclass">)  [unwired: 1 in, 1 out]
            n649 = Bundle By Name(cluster=w1224, "PassToStrikerPlay"=w1231) -> (w1225:T5)
            n650 = property class="Playbook"(reference=w1230, "offensive_plays"=w1225) -> (reference out=w1229:refnum<class "Playbook.lvclass">)  [unwired: 1 in, 1 out]
          }
        }
        frame "PassTo2ndStriker" {
          n651 = property class="Playbook"(reference=w1263) -> (reference out=w1261:refnum<class "Playbook.lvclass">, "offensive_plays"=w1268:T5)  [unwired: 1 in, 1 out]
          n652 = Unbundle By Name(w1268) -> ("PassTo2ndStrikerPlay"=w1267:refnum<class "PassTo2ndStriker.lvclass">)
          n653 = property class="PassTo2ndStriker"(reference=w1267) -> ("NumberOfRobots"=w1266:dbl)  [unwired: 1 in, 2 out]
          n654 = call-dynamic "pickOffensiveTeam.vi"("OffensiveTeam in"=w1259, "Game"=w1260, "KeeperTeam"=w1262, "number_of_robots"=w1266, "RobotRef"=w1264) -> ("OffensiveTeam out"=w1258:refnum<class "Ally.lvclass">, "RobotRef"=w1265:refnum<class "Robot.lvclass">[])  [unwired: 8 in, 1 out]
          n655 = for {
            tunnel: [w1269] -> w1256 mode=indexing
            tunnel: w1265 -> [w1275] mode=indexing
            shift-right: [w1276] -> w1257
            shift-left: w1261 -> [w1277]
            shift-right: [w1272] -> _
            shift-left: w1268 -> [w1271]
            i -> [w1274]
            n656 = Unbundle By Name(w1271) -> ("PassTo2ndStrikerPlay"=w1270:refnum<class "PassTo2ndStriker.lvclass">)
            n657 = property class="PassTo2ndStriker"(reference=w1270) -> (reference out=w1279:refnum<class "PassTo2ndStriker.lvclass">, "Roles"=w1281:T29)  [unwired: 1 in, 1 out]
            n658 = Increment(x=w1274) -> (x+1=w1273:i32)
            n659 = case shown="3" w1273 {
              tunnel: w1281 -> [w1287 w1294 w1298]
              tunnel: [w1285 w1292 w1297] -> w1280
              tunnel: w1275 -> [w1284 w1290 w1299]
              tunnel: [w1282 w1289 w1296] -> w1269
              frame 1, Default {
                n660 = Unbundle By Name(w1287) -> ("PassKickerRole"=w1288:refnum<class "PassKickerRole.lvclass">)
                n661 = property class="Robot"(reference=w1284, "role"=roles."PassKicker") -> (reference out=w1282:refnum<class "Robot.lvclass">)  [unwired: 1 in, 1 out]
                n662 = property class="PassKickerRole"(reference=w1288, "RobotRef"=w1282) -> (reference out=w1286:refnum<class "PassKickerRole.lvclass">)  [unwired: 1 in, 1 out]
                n663 = Bundle By Name(cluster=w1287, "PassKickerRole"=w1286) -> (w1285:T29)
              }
              frame 2 {
                n664 = Unbundle By Name(w1294) -> ("PassObserverRole"=w1295:refnum<class "PassObserverRole.lvclass">)
                n665 = property class="Robot"(reference=w1290, "role"=roles."PassObserver") -> (reference out=w1289:refnum<class "Robot.lvclass">)  [unwired: 1 in, 1 out]
                n666 = property class="PassObserverRole"(reference=w1295, "RobotRef"=w1289) -> (reference out=w1293:refnum<class "PassObserverRole.lvclass">)  [unwired: 1 in, 1 out]
                n667 = Bundle By Name(cluster=w1294, "PassObserverRole"=w1293) -> (w1292:T29)
              }
              frame 3 {
                n668 = Unbundle By Name(w1298) -> ("PassReceiverRole"=w1302:refnum<class "PassReceiverRole.lvclass">)
                n669 = property class="Robot"(reference=w1299, "role"=roles."PassReceiver") -> (reference out=w1296:refnum<class "Robot.lvclass">)  [unwired: 1 in, 1 out]
                n670 = property class="PassReceiverRole"(reference=w1302, "RobotRef"=w1296) -> (reference out=w1301:refnum<class "PassReceiverRole.lvclass">)  [unwired: 1 in, 1 out]
                n671 = Bundle By Name(cluster=w1298, "PassReceiverRole"=w1301) -> (w1297:T29)
              }
            }
            n672 = property class="PassTo2ndStriker"(reference=w1279, "Roles"=w1280) -> (reference out=w1278:refnum<class "PassTo2ndStriker.lvclass">)  [unwired: 1 in, 1 out]
            n673 = Bundle By Name(cluster=w1271, "PassTo2ndStrikerPlay"=w1278) -> (w1272:T5)
            n674 = property class="Playbook"(reference=w1277, "offensive_plays"=w1272) -> (reference out=w1276:refnum<class "Playbook.lvclass">)  [unwired: 1 in, 1 out]
          }
        }
        frame "TableWithStriker" {
          n675 = property class="Playbook"(reference=w1310) -> (reference out=w1308:refnum<class "Playbook.lvclass">, "offensive_plays"=w1315:T5)  [unwired: 1 in, 1 out]
          n676 = Unbundle By Name(w1315) -> ("TableWithStrikerPlay"=w1314:refnum<class "TableWithStrikerPlay.lvclass">)
          n677 = property class="TableWithStrikerPlay"(reference=w1314) -> ("NumberOfRobots"=w1313:dbl)  [unwired: 1 in, 2 out]
          n678 = call-dynamic "pickOffensiveTeam.vi"("OffensiveTeam in"=w1306, "Game"=w1307, "KeeperTeam"=w1309, "number_of_robots"=w1313, "RobotRef"=w1311) -> ("OffensiveTeam out"=w1305:refnum<class "Ally.lvclass">, "RobotRef"=w1312:refnum<class "Robot.lvclass">[])  [unwired: 8 in, 1 out]
          n679 = for {
            tunnel: [w1316] -> w1303 mode=indexing
            tunnel: w1312 -> [w1322] mode=indexing
            shift-right: [w1323] -> w1304
            shift-left: w1308 -> [w1324]
            shift-right: [w1319] -> _
            shift-left: w1315 -> [w1318]
            i -> [w1321]
            n680 = Unbundle By Name(w1318) -> ("TableWithStrikerPlay"=w1317:refnum<class "TableWithStrikerPlay.lvclass">)
            n681 = property class="TableWithStrikerPlay"(reference=w1317) -> (reference out=w1326:refnum<class "TableWithStrikerPlay.lvclass">, "Roles"=w1328:T30)  [unwired: 1 in, 1 out]
            n682 = Increment(x=w1321) -> (x+1=w1320:i32)
            n683 = case shown="1, Default" w1320 {
              tunnel: w1328 -> [w1334 w1341 w1345]
              tunnel: [w1332 w1339 w1344] -> w1327
              tunnel: w1322 -> [w1331 w1337 w1346]
              tunnel: [w1329 w1336 w1343] -> w1316
              frame 1, Default {
                n684 = Unbundle By Name(w1334) -> ("TableFinalizerRole"=w1335:refnum<class "TableFinalizerRole.lvclass">)
                n685 = property class="Robot"(reference=w1331, "role"=roles."TableFinalizer") -> (reference out=w1329:refnum<class "Robot.lvclass">)  [unwired: 1 in, 1 out]
                n686 = property class="TableFinalizerRole"(reference=w1335, "RobotRef"=w1329) -> (reference out=w1333:refnum<class "TableFinalizerRole.lvclass">)  [unwired: 1 in, 1 out]
                n687 = Bundle By Name(cluster=w1334, "TableFinalizerRole"=w1333) -> (w1332:T30)
              }
              frame 2 {
                n688 = Unbundle By Name(w1341) -> ("TablerRole"=w1342:refnum<class "TablerRole.lvclass">)
                n689 = property class="Robot"(reference=w1337, "role"=roles."Tabler") -> (reference out=w1336:refnum<class "Robot.lvclass">)  [unwired: 1 in, 1 out]
                n690 = property class="TablerRole"(reference=w1342, "RobotRef"=w1336) -> (reference out=w1340:refnum<class "TablerRole.lvclass">)  [unwired: 1 in, 1 out]
                n691 = Bundle By Name(cluster=w1341, "TablerRole"=w1340) -> (w1339:T30)
              }
              frame 3 {
                n692 = Unbundle By Name(w1345) -> ("PassObserverRole"=w1349:refnum<class "PassObserverRole.lvclass">)
                n693 = property class="Robot"(reference=w1346, "role"=roles."PassObserver") -> (reference out=w1343:refnum<class "Robot.lvclass">)  [unwired: 1 in, 1 out]
                n694 = property class="PassObserverRole"(reference=w1349, "RobotRef"=w1343) -> (reference out=w1348:refnum<class "PassObserverRole.lvclass">)  [unwired: 1 in, 1 out]
                n695 = Bundle By Name(cluster=w1345, "PassObserverRole"=w1348) -> (w1344:T30)
              }
            }
            n696 = property class="TableWithStrikerPlay"(reference=w1326, "Roles"=w1327) -> (reference out=w1325:refnum<class "TableWithStrikerPlay.lvclass">)  [unwired: 1 in, 1 out]
            n697 = Bundle By Name(cluster=w1318, "TableWithStrikerPlay"=w1325) -> (w1319:T5)
            n698 = property class="Playbook"(reference=w1324, "offensive_plays"=w1319) -> (reference out=w1323:refnum<class "Playbook.lvclass">)  [unwired: 1 in, 1 out]
          }
        }
        frame "TableWith2ndStrikerPlay" {
          n699 = property class="Playbook"(reference=w1357) -> (reference out=w1355:refnum<class "Playbook.lvclass">, "offensive_plays"=w1362:T5)  [unwired: 1 in, 1 out]
          n700 = Unbundle By Name(w1362) -> ("TableWith2ndStrikerPlay"=w1361:refnum<class "TableWith2ndStrikerPlay.lvclass">)
          n701 = property class="TablePlay"(reference=w1361) -> ("NumberOfRobots"=w1360:dbl)  [unwired: 1 in, 2 out]
          n702 = call-dynamic "pickOffensiveTeam.vi"("OffensiveTeam in"=w1353, "Game"=w1354, "KeeperTeam"=w1356, "number_of_robots"=w1360, "RobotRef"=w1358) -> ("OffensiveTeam out"=w1352:refnum<class "Ally.lvclass">, "RobotRef"=w1359:refnum<class "Robot.lvclass">[])  [unwired: 8 in, 1 out]
          n703 = for {
            tunnel: [w1363] -> w1350 mode=indexing
            tunnel: w1359 -> [w1369] mode=indexing
            shift-right: [w1370] -> w1351
            shift-left: w1355 -> [w1371]
            shift-right: [w1366] -> _
            shift-left: w1362 -> [w1365]
            i -> [w1368]
            n704 = Unbundle By Name(w1365) -> ("TableWith2ndStrikerPlay"=w1364:refnum<class "TableWith2ndStrikerPlay.lvclass">)
            n705 = property class="TablePlay"(reference=w1364) -> (reference out=w1373:refnum<class "TableWith2ndStrikerPlay.lvclass">, "Roles"=w1375:T30)  [unwired: 1 in, 1 out]
            n706 = Increment(x=w1368) -> (x+1=w1367:i32)
            n707 = case shown="2" w1367 {
              tunnel: w1375 -> [w1381 w1388 w1392]
              tunnel: [w1379 w1386 w1391] -> w1374
              tunnel: w1369 -> [w1378 w1384 w1393]
              tunnel: [w1376 w1383 w1390] -> w1363
              frame 1, Default {
                n708 = Unbundle By Name(w1381) -> ("TableFinalizerRole"=w1382:refnum<class "TableFinalizerRole.lvclass">)
                n709 = property class="Robot"(reference=w1378, "role"=roles."TableFinalizer") -> (reference out=w1376:refnum<class "Robot.lvclass">)  [unwired: 1 in, 1 out]
                n710 = property class="TableFinalizerRole"(reference=w1382, "RobotRef"=w1376) -> (reference out=w1380:refnum<class "TableFinalizerRole.lvclass">)  [unwired: 1 in, 1 out]
                n711 = Bundle By Name(cluster=w1381, "TableFinalizerRole"=w1380) -> (w1379:T30)
              }
              frame 2 {
                n712 = Unbundle By Name(w1388) -> ("PassObserverRole"=w1389:refnum<class "PassObserverRole.lvclass">)
                n713 = property class="Robot"(reference=w1384, "role"=roles."PassObserver") -> (reference out=w1383:refnum<class "Robot.lvclass">)  [unwired: 1 in, 1 out]
                n714 = property class="PassObserverRole"(reference=w1389, "RobotRef"=w1383) -> (reference out=w1387:refnum<class "PassObserverRole.lvclass">)  [unwired: 1 in, 1 out]
                n715 = Bundle By Name(cluster=w1388, "PassObserverRole"=w1387) -> (w1386:T30)
              }
              frame 3 {
                n716 = Unbundle By Name(w1392) -> ("TablerRole"=w1396:refnum<class "TablerRole.lvclass">)
                n717 = property class="Robot"(reference=w1393, "role"=roles."Tabler") -> (reference out=w1390:refnum<class "Robot.lvclass">)  [unwired: 1 in, 1 out]
                n718 = property class="TablerRole"(reference=w1396, "RobotRef"=w1390) -> (reference out=w1395:refnum<class "TablerRole.lvclass">)  [unwired: 1 in, 1 out]
                n719 = Bundle By Name(cluster=w1392, "TablerRole"=w1395) -> (w1391:T30)
              }
            }
            n720 = property class="TablePlay"(reference=w1373, "Roles"=w1374) -> (reference out=w1372:refnum<class "TableWith2ndStrikerPlay.lvclass">)  [unwired: 1 in, 1 out]
            n721 = Bundle By Name(cluster=w1365, "TableWith2ndStrikerPlay"=w1372) -> (w1366:T5)
            n722 = property class="Playbook"(reference=w1371, "offensive_plays"=w1366) -> (reference out=w1370:refnum<class "Playbook.lvclass">)  [unwired: 1 in, 1 out]
          }
        }
        frame "KeeperPassToStriker" {
          n723 = property class="Playbook"(reference=w1404) -> (reference out=w1402:refnum<class "Playbook.lvclass">, "offensive_plays"=w1409:T5)  [unwired: 1 in, 1 out]
          n724 = Unbundle By Name(w1409) -> ("KeeperPassToStrikerPlay"=w1408:refnum<class "KeeperPassToStrikerPlay.lvclass">)
          n725 = property class="KeeperPassToStrikerPlay"(reference=w1408) -> ("NumberOfRobots"=w1407:dbl)  [unwired: 1 in, 2 out]
          n726 = call-dynamic "pickOffensiveTeam.vi"("OffensiveTeam in"=w1400, "Game"=w1401, "KeeperTeam"=w1403, "number_of_robots"=w1407, "RobotRef"=w1405) -> ("OffensiveTeam out"=w1399:refnum<class "Ally.lvclass">, "RobotRef"=w1406:refnum<class "Robot.lvclass">[])  [unwired: 8 in, 1 out]
          n727 = for {
            tunnel: [w1410] -> w1397 mode=indexing
            tunnel: w1406 -> [w1416] mode=indexing
            shift-right: [w1417] -> w1398
            shift-left: w1402 -> [w1418]
            shift-right: [w1413] -> _
            shift-left: w1409 -> [w1412]
            i -> [w1415]
            n728 = Unbundle By Name(w1412) -> ("KeeperPassToStrikerPlay"=w1411:refnum<class "KeeperPassToStrikerPlay.lvclass">)
            n729 = property class="KeeperPassToStrikerPlay"(reference=w1411) -> (reference out=w1420:refnum<class "KeeperPassToStrikerPlay.lvclass">, "Roles"=w1422:T31)  [unwired: 1 in, 1 out]
            n730 = Increment(x=w1415) -> (x+1=w1414:i32)
            n731 = case shown="1, Default" w1414 {
              tunnel: w1422 -> [w1428 w1435]
              tunnel: [w1426 w1433] -> w1421
              tunnel: w1416 -> [w1425 w1431]
              tunnel: [w1423 w1430] -> w1410
              frame 2 {
                n732 = Unbundle By Name(w1428) -> ("WaitPassRole"=w1429:refnum<class "WaitPassRole.lvclass">)
                n733 = property class="Robot"(reference=w1425, "role"=roles."WaitPass") -> (reference out=w1423:refnum<class "Robot.lvclass">)  [unwired: 1 in, 1 out]
                n734 = property class="WaitPassRole"(reference=w1429, "RobotRef"=w1423) -> (reference out=w1427:refnum<class "WaitPassRole.lvclass">)  [unwired: 1 in, 1 out]
                n735 = Bundle By Name(cluster=w1428, "WaitPassRole"=w1427) -> (w1426:T31)
              }
              frame 1, Default {
                n736 = Unbundle By Name(w1435) -> ("FollowAttackerRole"=w1436:refnum<class "FollowAttackerRole.lvclass">)
                n737 = property class="Robot"(reference=w1431, "role"=roles."FollowAttacker") -> (reference out=w1430:refnum<class "Robot.lvclass">)  [unwired: 1 in, 1 out]
                n738 = property class="FollowAttackerRole"(reference=w1436, "RobotRef"=w1430) -> (reference out=w1434:refnum<class "FollowAttackerRole.lvclass">)  [unwired: 1 in, 1 out]
                n739 = Bundle By Name(cluster=w1435, "FollowAttackerRole"=w1434) -> (w1433:T31)
              }
            }
            n740 = property class="KeeperPassToStrikerPlay"(reference=w1420, "Roles"=w1421) -> (reference out=w1419:refnum<class "KeeperPassToStrikerPlay.lvclass">)  [unwired: 1 in, 1 out]
            n741 = Bundle By Name(cluster=w1412, "KeeperPassToStrikerPlay"=w1419) -> (w1413:T5)
            n742 = property class="Playbook"(reference=w1418, "offensive_plays"=w1413) -> (reference out=w1417:refnum<class "Playbook.lvclass">)  [unwired: 1 in, 1 out]
          }
        }
        frame "Prepare Penalty Enemy" {
          n743 = property class="Playbook"(reference=w1437) -> (reference out=w1447:refnum<class "Playbook.lvclass">, "offensive_plays"=w1449:T5)  [unwired: 1 in, 1 out]
          n744 = Unbundle By Name(w1449) -> ("PreparePenaltyEnemyPlay"=w1448:refnum<class "PreparePenaltyEnemyPlay.lvclass">)
          n745 = property class="PreparePenaltyEnemyPlay"(reference=w1448) -> ("NumberOfRobots"=w1438:dbl)  [unwired: 1 in, 2 out]
          n746 = call-dynamic "pickOffensiveTeam.vi"("OffensiveTeam in"=w1444, "Game"=w1445, "KeeperTeam"=w1443, "number_of_robots"=w1438, "RobotRef"=w1442) -> ("OffensiveTeam out"=w1441:refnum<class "Ally.lvclass">, "RobotRef"=w1446:refnum<class "Robot.lvclass">[])  [unwired: 8 in, 1 out]
          n747 = for {
            tunnel: [w1450] -> w1439 mode=indexing
            tunnel: w1446 -> [w1456] mode=indexing
            shift-right: [w1457] -> w1440
            shift-left: w1447 -> [w1458]
            shift-right: [w1453] -> _
            shift-left: w1449 -> [w1452]
            i -> [w1455]
            n748 = Unbundle By Name(w1452) -> ("PreparePenaltyEnemyPlay"=w1451:refnum<class "PreparePenaltyEnemyPlay.lvclass">)
            n749 = property class="PreparePenaltyEnemyPlay"(reference=w1451) -> (reference out=w1460:refnum<class "PreparePenaltyEnemyPlay.lvclass">, "roles"=w1462:T32)  [unwired: 1 in, 1 out]
            n750 = Increment(x=w1455) -> (x+1=w1454:i32)
            n751 = case shown="1, Default" w1454 {
              tunnel: w1462 -> [w1468 w1475 w1482 w1489 w1491]
              tunnel: [w1467 w1474 w1481 w1488 w1493] -> w1461
              tunnel: w1456 -> [w1466 w1472 w1479 w1486 w1492]
              tunnel: [w1465 w1471 w1478 w1485 w1494] -> w1450
              frame 2 {
                n752 = Unbundle By Name(w1468) -> ("PenaltyDefenseRole 2"=w1469:refnum<class "PenaltyDefenseRole.lvclass">)
                n753 = property class="Robot"(reference=w1466, "role"=roles."PenaltyDefense") -> (reference out=w1465:refnum<class "Robot.lvclass">)  [unwired: 1 in, 1 out]
                n754 = property class="PenaltyDefenseRole"(reference=w1469, "RobotRef"=w1465) -> (reference out=w1464:refnum<class "PenaltyDefenseRole.lvclass">)  [unwired: 1 in, 1 out]
                n755 = Bundle By Name(cluster=w1468, "PenaltyDefenseRole 2"=w1464) -> (w1467:T32)
              }
              frame 3 {
                n756 = Unbundle By Name(w1475) -> ("PenaltyDefenseRole 3"=w1476:refnum<class "PenaltyDefenseRole.lvclass">)
                n757 = property class="Robot"(reference=w1472, "role"=roles."PenaltyDefense") -> (reference out=w1471:refnum<class "Robot.lvclass">)  [unwired: 1 in, 1 out]
                n758 = property class="PenaltyDefenseRole"(reference=w1476, "RobotRef"=w1471) -> (reference out=w1470:refnum<class "PenaltyDefenseRole.lvclass">)  [unwired: 1 in, 1 out]
                n759 = Bundle By Name(cluster=w1475, "PenaltyDefenseRole 3"=w1470) -> (w1474:T32)
              }
              frame 4 {
                n760 = Unbundle By Name(w1482) -> ("PenaltyDefenseRole 4"=w1483:refnum<class "PenaltyDefenseRole.lvclass">)
                n761 = property class="Robot"(reference=w1479, "role"=roles."PenaltyDefense") -> (reference out=w1478:refnum<class "Robot.lvclass">)  [unwired: 1 in, 1 out]
                n762 = property class="PenaltyDefenseRole"(reference=w1483, "RobotRef"=w1478) -> (reference out=w1477:refnum<class "PenaltyDefenseRole.lvclass">)  [unwired: 1 in, 1 out]
                n763 = Bundle By Name(cluster=w1482, "PenaltyDefenseRole 4"=w1477) -> (w1481:T32)
              }
              frame 5 {
                n764 = Unbundle By Name(w1489) -> ("PenaltyDefenseRole 5"=w1490:refnum<class "PenaltyDefenseRole.lvclass">)
                n765 = property class="Robot"(reference=w1486, "role"=roles."PenaltyDefense") -> (reference out=w1485:refnum<class "Robot.lvclass">)  [unwired: 1 in, 1 out]
                n766 = property class="PenaltyDefenseRole"(reference=w1490, "RobotRef"=w1485) -> (reference out=w1484:refnum<class "PenaltyDefenseRole.lvclass">)  [unwired: 1 in, 1 out]
                n767 = Bundle By Name(cluster=w1489, "PenaltyDefenseRole 5"=w1484) -> (w1488:T32)
              }
              frame 1, Default {
                n768 = Unbundle By Name(w1491) -> ("PenaltyDefenseRole 1"=w1497:refnum<class "PenaltyDefenseRole.lvclass">)
                n769 = property class="Robot"(reference=w1492, "role"=roles."PenaltyDefense") -> (reference out=w1494:refnum<class "Robot.lvclass">)  [unwired: 1 in, 1 out]
                n770 = property class="PenaltyDefenseRole"(reference=w1497, "RobotRef"=w1494) -> (reference out=w1495:refnum<class "PenaltyDefenseRole.lvclass">)  [unwired: 1 in, 1 out]
                n771 = Bundle By Name(cluster=w1491, "PenaltyDefenseRole 1"=w1495) -> (w1493:T32)
              }
            }
            n772 = property class="PreparePenaltyEnemyPlay"(reference=w1460, "roles"=w1461) -> (reference out=w1459:refnum<class "PreparePenaltyEnemyPlay.lvclass">)  [unwired: 1 in, 1 out]
            n773 = Bundle By Name(cluster=w1452, "PreparePenaltyEnemyPlay"=w1459) -> (w1453:T5)
            n774 = property class="Playbook"(reference=w1458, "offensive_plays"=w1453) -> (reference out=w1457:refnum<class "Playbook.lvclass">)  [unwired: 1 in, 1 out]
          }
        }
        frame "KickPenaltyAlly" {
          n775 = property class="Playbook"(reference=w1510) -> (reference out=w1503:refnum<class "Playbook.lvclass">, "offensive_plays"=w1509:T5)  [unwired: 1 in, 1 out]
          n776 = Unbundle By Name(w1509) -> ("KickPenaltyAllyPlay"=w1506:refnum<class "KickPenaltyAllyPlay.lvclass">)
          n777 = property class="KickPenaltyAllyPlay"(reference=w1506) -> ("NumberOfRobots"=w1505:dbl)  [unwired: 1 in, 2 out]
          n778 = call-dynamic "pickOffensiveTeam.vi"("OffensiveTeam in"=w1499, "Game"=w1498, "KeeperTeam"=w1500, "number_of_robots"=w1505, "RobotRef"=w1504) -> ("OffensiveTeam out"=w1501:refnum<class "Ally.lvclass">, "RobotRef"=w1502:refnum<class "Robot.lvclass">[])  [unwired: 8 in, 1 out]
          n779 = for {
            tunnel: [w1511] -> w1507 mode=indexing
            tunnel: w1502 -> [w1517] mode=indexing
            shift-right: [w1518] -> w1508
            shift-left: w1503 -> [w1519]
            shift-right: [w1514] -> _
            shift-left: w1509 -> [w1513]
            i -> [w1516]
            n780 = Unbundle By Name(w1513) -> ("KickPenaltyAllyPlay"=w1512:refnum<class "KickPenaltyAllyPlay.lvclass">)
            n781 = property class="KickPenaltyAllyPlay"(reference=w1512) -> (reference out=w1521:refnum<class "KickPenaltyAllyPlay.lvclass">, "Roles"=w1523:T33)  [unwired: 1 in, 1 out]
            n782 = Increment(x=w1516) -> (x+1=w1515:i32)
            n783 = case shown="5" w1515 {
              tunnel: w1523 -> [w1529 w1536 w1543 w1550 w1557]
              tunnel: [w1527 w1534 w1541 w1548 w1555] -> w1522
              tunnel: w1517 -> [w1526 w1533 w1540 w1547 w1554]
              tunnel: [w1524 w1531 w1538 w1545 w1552] -> w1511
              frame 1, Default {
                n784 = Unbundle By Name(w1529) -> ("PenaltyAttackerRole"=w1530:refnum<class "PenaltyAttackerRole.lvclass">)
                n785 = property class="Robot"(reference=w1526, "role"=roles."PenaltyAttacker") -> (reference out=w1524:refnum<class "Robot.lvclass">)  [unwired: 1 in, 1 out]
                n786 = property class="PenaltyAttackerRole"(reference=w1530, "RobotRef"=w1524) -> (reference out=w1528:refnum<class "PenaltyAttackerRole.lvclass">)  [unwired: 1 in, 1 out]
                n787 = Bundle By Name(cluster=w1529, "PenaltyAttackerRole"=w1528) -> (w1527:T33)
              }
              frame 2 {
                n788 = Unbundle By Name(w1536) -> ("HaltRole"=w1537:refnum<class "HaltRole.lvclass">)
                n789 = property class="Robot"(reference=w1533, "role"=roles."Halt") -> (reference out=w1531:refnum<class "Robot.lvclass">)  [unwired: 1 in, 1 out]
                n790 = property class="HaltRole"(reference=w1537, "RobotRef"=w1531) -> (reference out=w1535:refnum<class "HaltRole.lvclass">)  [unwired: 1 in, 1 out]
                n791 = Bundle By Name(cluster=w1536, "HaltRole"=w1535) -> (w1534:T33)
              }
              frame 3 {
                n792 = Unbundle By Name(w1543) -> ("HaltRole 2"=w1544:refnum<class "HaltRole.lvclass">)
                n793 = property class="Robot"(reference=w1540, "role"=roles."Halt") -> (reference out=w1538:refnum<class "Robot.lvclass">)  [unwired: 1 in, 1 out]
                n794 = property class="HaltRole"(reference=w1544, "RobotRef"=w1538) -> (reference out=w1542:refnum<class "HaltRole.lvclass">)  [unwired: 1 in, 1 out]
                n795 = Bundle By Name(cluster=w1543, "HaltRole 2"=w1542) -> (w1541:T33)
              }
              frame 4 {
                n796 = Unbundle By Name(w1550) -> ("HaltRole 3"=w1551:refnum<class "HaltRole.lvclass">)
                n797 = property class="Robot"(reference=w1547, "role"=roles."Halt") -> (reference out=w1545:refnum<class "Robot.lvclass">)  [unwired: 1 in, 1 out]
                n798 = property class="HaltRole"(reference=w1551, "RobotRef"=w1545) -> (reference out=w1549:refnum<class "HaltRole.lvclass">)  [unwired: 1 in, 1 out]
                n799 = Bundle By Name(cluster=w1550, "HaltRole 3"=w1549) -> (w1548:T33)
              }
              frame 5 {
                n800 = Unbundle By Name(w1557) -> ("HaltRole 4"=w1558:refnum<class "HaltRole.lvclass">)
                n801 = property class="Robot"(reference=w1554, "role"=roles."Halt") -> (reference out=w1552:refnum<class "Robot.lvclass">)  [unwired: 1 in, 1 out]
                n802 = property class="HaltRole"(reference=w1558, "RobotRef"=w1552) -> (reference out=w1556:refnum<class "HaltRole.lvclass">)  [unwired: 1 in, 1 out]
                n803 = Bundle By Name(cluster=w1557, "HaltRole 4"=w1556) -> (w1555:T33)
              }
            }
            n804 = property class="KickPenaltyAllyPlay"(reference=w1521, "Roles"=w1522) -> (reference out=w1520:refnum<class "KickPenaltyAllyPlay.lvclass">)  [unwired: 1 in, 1 out]
            n805 = Bundle By Name(cluster=w1513, "KickPenaltyAllyPlay"=w1520) -> (w1514:T5)
            n806 = property class="Playbook"(reference=w1519, "offensive_plays"=w1514) -> (reference out=w1518:refnum<class "Playbook.lvclass">)  [unwired: 1 in, 1 out]
          }
        }
      }
      n807 = property class="Ally"(reference=w20, "RobotRef"=w19) -> (reference out=w18:refnum<class "Ally.lvclass">)  [unwired: 1 in, 1 out]
      n808 = property class="Game"(reference=w15, "OffensiveTeam"=w18, "Playbook"=w17) -> (reference out=w14:refnum<class "Game.lvclass">)  [unwired: 1 in, 1 out]
    }
    frame Error {
    }
  }
  "error out" <- w3
  "Game out" <- w1
